vi "f dependence NLH_2Dsweep.vi"() -> ()   [LabVIEW 2022 SP3]
uses:
  C:/Program Files/National Instruments/LabVIEW 2022/instr.lib/OptiCool/QDInstrument.dll
  <vilib>/Analysis/baseanly.llb/Mean (DBL).vi
  <vilib>/Utility/file.llb/Write Delimited Spreadsheet (DBL).vi
  <vilib>/Analysis/NI_AALBase.lvlib
panel:
  in  "Log Step":dbl=1.0
  in  "End Value (Hz)":dbl=40000.0
  in  "Start Value (Hz)":dbl=17.7
  out "Frequency":dbl
  out "error out":errorcluster
  out "Instrument Ref Out":refnum<k24>
  in  "Temperature \n& Field Function":bool=TRUE
  in  "IP Address 2":string="169.254.170.239"
  in  "Remote":bool=TRUE
  in  "Delay":dbl=5.0
  in  "WaitForTemperature":bool=TRUE
  in  "WaitForField":bool=TRUE
  in  "Set  T  (K)":dbl=2.0
  in  "T  Rate (K/min)":dbl=10.0
  in  "Temperature Approach":i32(ring)=1 items=["FastSettle", "NoOvershoot"]
  in  "Mode":i32(ring) items=["Persistent", "Driven"]
  in  "Set F (Oe)":dbl format="%#_13g"
  in  "F Rate (Oe/s)":dbl=100.0 format="%#_13g"
  in  "Field Approach":i32(ring) items=["Linear", "NoOvershoot", "Oscillate"]
  out "Measuring":bool
  out "Temperature":dbl=2.045465922355652
  out "Field":dbl=-0.1023246817290783
  out "Field Status":i32(ring)=4 items=["MagnetUnknown"=0, "StablePersistent"=1, "WarmingSwitch"=2, "CoolingSwitch"=3, "StableDriven"=4, "Iterating"=5, "Charging"=6, "Discharging"=7, "CurrentError"=8, "MagnetFailure"=15]
  out "Temperature Status":i32(ring)=1 items=["TemperatureUnknown"=0, "Stable"=1, "Tracking"=2, "Near"=5, "Chasing"=6, "Filling"=7, "Standby"=10, "Disabled"=13, "ImpedanceNotFunction"=14, "TempFailure"=15]
  out "Ri_2 phase":cluster{dbl[], dbl[]}(graph)={[0.09999999999999998, 0.12, 0.14, 0.16000000000000003, 0.17999999999999994, 0.19999999999999996, 0.21999999999999997, 0.24, 0.26, 0.28, 0.29999999999999993, 0.31999999999999995, 0.33999999999999997, 0.36, 0.38, 0.4, 0.42000000000000004, 0.43999999999999995, 0.45999999999999996, 0.48, 0.5, 0.52, 0.54, 0.56, 0.5800000000000001, 0.6, 0.62, 0.64, 0.6599999999999999, 0.6799999999999999, 0.7, 0.72, 0.74, 0.76, 0.78, 0.8, 0.8200000000000001, 0.84, 0.86, 0.88, 0.9, 0.92, 0.94, 0.96, 0.98, 1.0, 0.98, 0.96, 0.94, 0.92, 0.9, 0.88, 0.86, 0.84, 0.82, 0.8, 0.78, 0.76, 0.74, 0.72, 0.7, 0.6799999999999999, 0.66, 0.64, 0.62, 0.6, 0.58, 0.56, 0.54, 0.52, 0.5, 0.48, 0.45999999999999996, 0.44000000000000006, 0.42000000000000004, 0.4, 0.38, 0.36, 0.33999999999999997, 0.32, 0.30000000000000004, 0.28, 0.26, 0.24000000000000002, 0.22, 0.2, 0.18, 0.16, 0.14, 0.12000000000000001, 0.1, 0.09999999999999998, 0.12, 0.14, 0.16000000000000003, 0.17999999999999994, 0.19999999999999996, 0.21999999999999997, 0.24, 0.26, 0.28, 0.29999999999999993, 0.31999999999999995, 0.33999999999999997, 0.36, 0.38, 0.4, 0.42000000000000004, 0.43999999999999995, 0.45999999999999996, 0.48, 0.5, 0.52, 0.54, 0.56, 0.5800000000000001, 0.6, 0.62, 0.64, 0.6599999999999999, 0.6799999999999999, 0.7, 0.72, 0.74, 0.76, 0.78, 0.8, 0.8200000000000001, 0.84, 0.86, 0.88, 0.9, 0.92, 0.94, 0.96, 0.98, 1.0, 0.98, 0.96, 0.94, 0.92, 0.9, 0.88, 0.86, 0.84, 0.82, 0.8, 0.78, 0.76, 0.74, 0.72, 0.7, 0.6799999999999999, 0.66, 0.64, 0.62, 0.6, 0.58, 0.56, 0.54, 0.52, 0.5, 0.48, 0.45999999999999996, 0.44000000000000006, 0.42000000000000004, 0.4, 0.38, 0.36, 0.33999999999999997, 0.32, 0.30000000000000004, 0.28, 0.26, 0.24000000000000002, 0.22, 0.2, 0.18, 0.16, 0.14, 0.12000000000000001, 0.1], [-135.0737798780838, -134.6738634306522, -134.37974821597692, -134.1329191164491, -133.93959648319287, -133.82499792211388, -133.72512789792637, -133.65178972403427, -133.51483265219323, -133.47620113245185, -133.49883143367305, -133.37910330366344, -133.21293365173887, -133.27350677537933, -133.27106017405902, -133.21754869761966, -133.21281374202516, -133.1841427403462, -133.16708735849346, -133.1229624716472, -133.09716887007846, -133.0742714725264, -133.06316615999822, -133.04544862618698, -133.02604088036725, -133.03034506308185, -133.00064263870803, -132.98704248472112, -132.95992367769645, -132.96773298284512, -132.9462513593375, -132.92388738374774, -132.93487095070657, -132.92245049681333, -132.91747172466938, -132.90231743575433, -132.88556409154268, -132.881237082976, -132.87117074587596, -132.86576987764798, -132.85386852066148, -132.84708304664974, -132.84538130977083, -132.83586557346655, -132.8255489140817, -132.82629889245763, -132.8177816715776, -132.82326025843324, -132.8336140133908, -132.8454189176914, -132.8516410833353, -132.85806140932092, -132.84285801056097, -132.84644282891838, -132.84700096802584, -132.84976756233482, -132.86482634382176, -132.86727458409388, -132.8588624021069, -132.88644179903636, -132.9058800327217, -132.87699682828833, -132.88999304396324, -132.91108879474103, -132.92301179840743, -132.92346083291895, -132.93641029158624, -132.94113870472373, -132.9606516890803, -132.96437166584263, -132.98433647368265, -132.9875119411151, -133.01231262066918, -133.0688900958854, -133.09190630466588, -133.1264003742024, -133.15155411140012, -133.93832528791813, -133.13251976736467, -133.22378740142432, -133.3539090592655, -133.3970887669385, -133.4425242756172, -133.49287186771852, -133.60223065290106, -133.75321879185125, -133.92848825397414, -134.11303813477105, -134.45190508345792, -135.10675452695267, -124.76072580560799, -89.50174321642196, -89.14605038980542, -88.84594353514626, -88.65669391405325, -88.50217230984028, -88.2292578588941, -88.20060177628105, -88.09441994431185, -88.00398201709041, -87.92508441731627, -87.88589798731445, -87.82014491326349, -87.79601841325153, -87.73700247935645, -87.69563779511853, -87.64024863816759, -87.6394010617623, -87.60257219060512, -87.55344363152862, -87.54324222165285, -87.51258348919042, -87.49839628540947, -87.48024090287525, -87.4663422228203, -87.44267105162086, -87.43676483856159, -87.40019935701899, -87.40049945685288, -87.38876942892429, -87.3757429912223, -87.35429406648153, -87.34428274476673, -87.33889962417248, -87.33853163161574, -87.32024261424039, -87.31903405804312, -87.30663336163828, -87.28680101385758, -87.28627293404885, -87.27451339574941, -87.26365333274687, -87.25364549630169, -87.24446928127777, -87.23761000479438, -87.24664691292533, -87.2206145740333, -87.22117860050086, -87.2360405527259, -87.23323381946209, -87.26842924538664, -87.23137885199706, -87.2385360459189, -87.25273929485618, -87.26039540250387, -87.25517989532322, -87.26120027002698, -87.25416045268364, -87.28418213348777, -87.29625747302379, -87.29755965406775, -87.29328958611812, -87.29095955610856, -87.30159590257846, -87.29739952834753, -87.32502449307063, -87.31280059465371, -87.34807549336224, -87.35104915499241, -87.35270893749001, -87.38974493852264, -87.42258216936716, -87.38265602907923, -87.42896961420581, -87.45151311724116, -87.47074471126548, -87.51773574830506, -87.56305113613072, -87.39521544539879, -87.67315367482476, -87.74315739254689, -87.74764259560797, -87.78722254082936, -87.87871776739563, -88.01195362145981, -88.22210844624024, -88.26255081520787, -88.37855415135323, -88.88064210120181, -89.15599768975594, -89.43545944095864, -67.88194047928333, -67.88194047928333]}
  out "Ri_1 phase":cluster{dbl[], dbl[]}(graph)={[0.09999999999999998, 0.12, 0.14, 0.16000000000000003, 0.17999999999999994, 0.19999999999999996, 0.21999999999999997, 0.24, 0.26, 0.28, 0.29999999999999993, 0.31999999999999995, 0.33999999999999997, 0.36, 0.38, 0.4, 0.42000000000000004, 0.43999999999999995, 0.45999999999999996, 0.48, 0.5, 0.52, 0.54, 0.56, 0.5800000000000001, 0.6, 0.62, 0.64, 0.6599999999999999, 0.6799999999999999, 0.7, 0.72, 0.74, 0.76, 0.78, 0.8, 0.8200000000000001, 0.84, 0.86, 0.88, 0.9, 0.92, 0.94, 0.96, 0.98, 1.0, 0.98, 0.96, 0.94, 0.92, 0.9, 0.88, 0.86, 0.84, 0.82, 0.8, 0.78, 0.76, 0.74, 0.72, 0.7, 0.6799999999999999, 0.66, 0.64, 0.62, 0.6, 0.58, 0.56, 0.54, 0.52, 0.5, 0.48, 0.45999999999999996, 0.44000000000000006, 0.42000000000000004, 0.4, 0.38, 0.36, 0.33999999999999997, 0.32, 0.30000000000000004, 0.28, 0.26, 0.24000000000000002, 0.22, 0.2, 0.18, 0.16, 0.14, 0.12000000000000001, 0.1, 0.09999999999999998, 0.12, 0.14, 0.16000000000000003, 0.17999999999999994, 0.19999999999999996, 0.21999999999999997, 0.24, 0.26, 0.28, 0.29999999999999993, 0.31999999999999995, 0.33999999999999997, 0.36, 0.38, 0.4, 0.42000000000000004, 0.43999999999999995, 0.45999999999999996, 0.48, 0.5, 0.52, 0.54, 0.56, 0.5800000000000001, 0.6, 0.62, 0.64, 0.6599999999999999, 0.6799999999999999, 0.7, 0.72, 0.74, 0.76, 0.78, 0.8, 0.8200000000000001, 0.84, 0.86, 0.88, 0.9, 0.92, 0.94, 0.96, 0.98, 1.0, 0.98, 0.96, 0.94, 0.92, 0.9, 0.88, 0.86, 0.84, 0.82, 0.8, 0.78, 0.76, 0.74, 0.72, 0.7, 0.6799999999999999, 0.66, 0.64, 0.62, 0.6, 0.58, 0.56, 0.54, 0.52, 0.5, 0.48, 0.45999999999999996, 0.44000000000000006, 0.42000000000000004, 0.4, 0.38, 0.36, 0.33999999999999997, 0.32, 0.30000000000000004, 0.28, 0.26, 0.24000000000000002, 0.22, 0.2, 0.18, 0.16, 0.14, 0.12000000000000001, 0.1], [126.78108864351137, 127.45286903626857, 127.95719233953537, 128.14548768192813, 128.2402724756276, 128.4605048589487, 128.66016247507395, 128.78004628646207, 128.85380119553557, 128.945308050546, 129.00594825216675, 129.1174793127654, 125.93035564325805, 128.99616398776885, 129.01096513526798, 128.99858528612694, 129.03821355303282, 129.0423277101241, 129.1060564530601, 129.12134565618365, 129.12218412588027, 129.16712187372542, 129.1716351205436, 129.1576166175744, 129.1739493965666, 129.22295454798373, 129.2303923286002, 129.2532206876488, 129.22564402818136, 129.24977504964798, 129.25454428704774, 129.2236334227617, 129.24706199685042, 129.2433757601247, 129.26065634538244, 129.24704726302411, 129.26737715657828, 129.25153494751845, 129.246018320394, 129.27084220325727, 129.26200021632502, 129.2815900734443, 129.25572165721184, 129.2713787153919, 129.27714146359114, 129.26320898916032, 129.26130754745333, 129.23228748819213, 129.23260322371937, 129.24085101357815, 129.20001021516066, 129.18928968116475, 129.22736479334458, 129.23076137993036, 129.21676154055228, 129.16377399211459, 129.1488883594887, 129.14107631735763, 129.17351120766202, 129.13764733091995, 129.13942445055497, 129.13611111142535, 129.12439365492142, 129.09365051881986, 129.04689998820783, 129.07255318625485, 129.0762023274164, 129.03056853240804, 128.98843713843775, 129.00993007515308, 128.96980878114644, 128.97196179961242, 128.93367450266246, 128.8432547892745, 128.77294830523502, 128.77850864107342, 128.26159472371137, 120.9819473629494, 128.91362581026087, 128.85130036343432, 128.75506679568952, 128.64553318215607, 128.5269184940437, 128.37639368365402, 128.19973263276748, 128.11080720159285, 127.84397610864357, 127.57598196631716, 127.36840896927713, 126.4699555939904, 122.15900482546692, -155.25487809300571, -154.75930960822615, -154.06908162364144, -153.69651442588355, -153.35566603542182, -153.23294540243333, -153.1114136645777, -152.8025382830503, -152.64398344398305, -152.52815097235072, -152.39578139944246, -152.4164853144777, -160.759413971048, -152.37498784365977, -152.3997145906726, -152.3686132746472, -152.27205329420735, -152.22153743200627, -152.20204337088634, -152.06607044245763, -152.0586998411544, -152.08655249501595, -152.03743666503073, -151.98381101431457, -151.9606367889107, -151.91112648537748, -151.92318997154743, -151.88886269968575, -151.86095513823875, -151.84712349726647, -151.8467203751335, -151.83654816655485, -151.83466546583742, -151.77972437121562, -151.75955524254454, -151.74101876892612, -151.74814437160126, -151.73846749290755, -151.71965063994767, -151.73507745360297, -151.70148169603394, -151.68277714268805, -151.68376267193642, -151.6789107792956, -151.68539186653047, -151.6809435268432, -151.69581765024503, -151.69398875114774, -151.71075155504255, -151.74117286964352, -151.75504731698328, -151.7397603042772, -151.78231484385356, -151.79544209254783, -151.80143331080117, -151.84067413704435, -151.85962716508706, -151.87822739965404, -151.91103936506607, -151.91923332818104, -151.93509570614805, -151.98136529122525, -151.97685217566038, -152.0012327141608, -152.02285309703487, -152.09741752528834, -152.1068998768356, -152.12333750684087, -152.15249427417922, -152.21610575405555, -152.28574184251096, -152.29089791668042, -152.30516178154488, -152.35145853535226, -152.450566439704, -152.50934427301326, -152.70530235536185, -153.48538331429216, -152.54768281995285, -152.61612358031286, -152.75102902160276, -152.87046583001037, -153.08098511590293, -153.26088730787697, -153.53049426796596, -153.64021310128948, -153.88983077611812, -154.39490952060976, -154.97594326878533, -154.724275972751, -25.54701889784434]}
  out "Ri_2":cluster{dbl[], dbl[]}(graph)={[0.09999999999999998, 0.12, 0.14, 0.16000000000000003, 0.17999999999999994, 0.19999999999999996, 0.21999999999999997, 0.24, 0.26, 0.28, 0.29999999999999993, 0.31999999999999995, 0.33999999999999997, 0.36, 0.38, 0.4, 0.42000000000000004, 0.43999999999999995, 0.45999999999999996, 0.48, 0.5, 0.52, 0.54, 0.56, 0.5800000000000001, 0.6, 0.62, 0.64, 0.6599999999999999, 0.6799999999999999, 0.7, 0.72, 0.74, 0.76, 0.78, 0.8, 0.8200000000000001, 0.84, 0.86, 0.88, 0.9, 0.92, 0.94, 0.96, 0.98, 1.0, 0.98, 0.96, 0.94, 0.92, 0.9, 0.88, 0.86, 0.84, 0.82, 0.8, 0.78, 0.76, 0.74, 0.72, 0.7, 0.6799999999999999, 0.66, 0.64, 0.62, 0.6, 0.58, 0.56, 0.54, 0.52, 0.5, 0.48, 0.45999999999999996, 0.44000000000000006, 0.42000000000000004, 0.4, 0.38, 0.36, 0.33999999999999997, 0.32, 0.30000000000000004, 0.28, 0.26, 0.24000000000000002, 0.22, 0.2, 0.18, 0.16, 0.14, 0.12000000000000001, 0.1, 0.09999999999999998, 0.12, 0.14, 0.16000000000000003, 0.17999999999999994, 0.19999999999999996, 0.21999999999999997, 0.24, 0.26, 0.28, 0.29999999999999993, 0.31999999999999995, 0.33999999999999997, 0.36, 0.38, 0.4, 0.42000000000000004, 0.43999999999999995, 0.45999999999999996, 0.48, 0.5, 0.52, 0.54, 0.56, 0.5800000000000001, 0.6, 0.62, 0.64, 0.6599999999999999, 0.6799999999999999, 0.7, 0.72, 0.74, 0.76, 0.78, 0.8, 0.8200000000000001, 0.84, 0.86, 0.88, 0.9, 0.92, 0.94, 0.96, 0.98, 1.0, 0.98, 0.96, 0.94, 0.92, 0.9, 0.88, 0.86, 0.84, 0.82, 0.8, 0.78, 0.76, 0.74, 0.72, 0.7, 0.6799999999999999, 0.66, 0.64, 0.62, 0.6, 0.58, 0.56, 0.54, 0.52, 0.5, 0.48, 0.45999999999999996, 0.44000000000000006, 0.42000000000000004, 0.4, 0.38, 0.36, 0.33999999999999997, 0.32, 0.30000000000000004, 0.28, 0.26, 0.24000000000000002, 0.22, 0.2, 0.18, 0.16, 0.14, 0.12000000000000001, 0.1], [27.371127865925015, 28.03873360270576, 28.46790461906138, 28.806943395600985, 29.071407285608636, 29.323295423352075, 29.462283711911706, 29.588953410180608, 29.706307017591357, 29.804227381977352, 29.87886111106559, 29.996116648909492, 30.195931132223937, 29.9884898058237, 30.055397066752594, 30.063982766666918, 30.109896580846595, 30.179554870002743, 30.170072825304572, 30.175397841954556, 30.20266242174663, 30.199676710261986, 30.20862007206962, 30.232010687672023, 30.25006843906505, 30.208577391057474, 30.285871424440206, 30.25536260196531, 30.24120314721451, 30.23077945837067, 30.230477005377466, 30.22206486695692, 30.225997495742032, 30.230263862260664, 30.20740393202253, 30.211300547061118, 30.21208431622353, 30.184907444070042, 30.182773909229088, 30.17902335943376, 30.16788755735149, 30.146107050335754, 30.134406107300926, 30.122307887553678, 30.13298693800453, 31.202979545844265, 31.210305140532736, 31.274406560955054, 31.305924728646062, 31.32743742693625, 31.375770721793792, 31.41382858703819, 31.45271665563307, 31.46916619733765, 31.532341922014098, 31.579997682637718, 31.59500614453121, 31.646800008509103, 31.695365022790494, 31.746853486268666, 31.798078625890966, 31.824707946574527, 31.89690056166134, 31.94018053437305, 32.01268881637008, 32.06636872763467, 32.135039395345515, 32.19692297138488, 32.260290459052655, 32.31072327457344, 32.380782444119205, 32.46545102212157, 32.534119464205524, 32.65882509715479, 32.72562027716687, 32.772164759910204, 31.414326516917146, 27.175202751891387, 32.99406085081532, 33.1423739100909, 33.28288253006214, 33.48812700032473, 33.73611411646078, 33.9781939345709, 34.29950602104752, 34.61918175500793, 35.06293433592041, 35.49518695051094, 36.256808448279884, 38.31013406059865, 501.19496515581875, 26.805737505344652, 27.450048924243337, 27.884394712122138, 28.24044516317822, 28.53430295508529, 28.764528334010045, 28.96197838575729, 29.105816365304005, 29.355232984041944, 29.34777886019463, 29.43287936231009, 29.62774349540086, 29.86465695141408, 29.608272863377074, 29.66921999186081, 29.70063847337968, 29.714424220713198, 29.786978685230352, 29.814319234323147, 29.826654999997462, 29.858808079716006, 29.84850588904362, 29.835423649303713, 29.871251466983324, 29.904019985626224, 29.899198678955656, 29.906795896054145, 29.90400614385718, 29.903859410313423, 29.90866679269539, 29.906609993632678, 29.89947029239501, 29.889654317635724, 29.914131514562797, 29.89903218199667, 29.896801089141448, 29.893727436511856, 29.88599371103664, 29.87423537654639, 29.86604845504494, 29.873501668548162, 29.84836006279222, 29.8497650723906, 29.851025865972254, 29.855406310478582, 30.90378884193393, 30.92260344391088, 30.965941923321747, 31.007698997219396, 31.03181453129471, 31.079098855420387, 31.111474766773938, 31.14532041453912, 31.190307610789297, 31.239550892642928, 31.26858596616326, 31.30525453943163, 31.36698598822591, 31.407572289858972, 31.432621279246682, 31.48459816196743, 31.533379016650517, 31.569188358430146, 31.66020477677031, 31.70991492962698, 31.733959217395633, 31.78738364022895, 31.87665028118242, 31.942457880633185, 31.988808527675072, 32.0825556507543, 32.17690322547313, 32.158098239659864, 32.263369173607806, 32.348466821304804, 32.43680396652162, 31.651152253438767, 28.498596681427244, 32.633886474836245, 32.72261637427303, 32.90277867221614, 33.09550043742226, 33.27705165299585, 33.54280965027385, 33.79957889026999, 34.12170714222017, 34.63130452806735, 35.09460603644337, 35.815529001325366, 38.05801784237739, 581.0849422120803, 581.0849422120803]}
  out "Ri_1":cluster{dbl[], dbl[]}(graph)={[0.09999999999999998, 0.12, 0.14, 0.16000000000000003, 0.17999999999999994, 0.19999999999999996, 0.21999999999999997, 0.24, 0.26, 0.28, 0.29999999999999993, 0.31999999999999995, 0.33999999999999997, 0.36, 0.38, 0.4, 0.42000000000000004, 0.43999999999999995, 0.45999999999999996, 0.48, 0.5, 0.52, 0.54, 0.56, 0.5800000000000001, 0.6, 0.62, 0.64, 0.6599999999999999, 0.6799999999999999, 0.7, 0.72, 0.74, 0.76, 0.78, 0.8, 0.8200000000000001, 0.84, 0.86, 0.88, 0.9, 0.92, 0.94, 0.96, 0.98, 1.0, 0.98, 0.96, 0.94, 0.92, 0.9, 0.88, 0.86, 0.84, 0.82, 0.8, 0.78, 0.76, 0.74, 0.72, 0.7, 0.6799999999999999, 0.66, 0.64, 0.62, 0.6, 0.58, 0.56, 0.54, 0.52, 0.5, 0.48, 0.45999999999999996, 0.44000000000000006, 0.42000000000000004, 0.4, 0.38, 0.36, 0.33999999999999997, 0.32, 0.30000000000000004, 0.28, 0.26, 0.24000000000000002, 0.22, 0.2, 0.18, 0.16, 0.14, 0.12000000000000001, 0.1, 0.09999999999999998, 0.12, 0.14, 0.16000000000000003, 0.17999999999999994, 0.19999999999999996, 0.21999999999999997, 0.24, 0.26, 0.28, 0.29999999999999993, 0.31999999999999995, 0.33999999999999997, 0.36, 0.38, 0.4, 0.42000000000000004, 0.43999999999999995, 0.45999999999999996, 0.48, 0.5, 0.52, 0.54, 0.56, 0.5800000000000001, 0.6, 0.62, 0.64, 0.6599999999999999, 0.6799999999999999, 0.7, 0.72, 0.74, 0.76, 0.78, 0.8, 0.8200000000000001, 0.84, 0.86, 0.88, 0.9, 0.92, 0.94, 0.96, 0.98, 1.0, 0.98, 0.96, 0.94, 0.92, 0.9, 0.88, 0.86, 0.84, 0.82, 0.8, 0.78, 0.76, 0.74, 0.72, 0.7, 0.6799999999999999, 0.66, 0.64, 0.62, 0.6, 0.58, 0.56, 0.54, 0.52, 0.5, 0.48, 0.45999999999999996, 0.44000000000000006, 0.42000000000000004, 0.4, 0.38, 0.36, 0.33999999999999997, 0.32, 0.30000000000000004, 0.28, 0.26, 0.24000000000000002, 0.22, 0.2, 0.18, 0.16, 0.14, 0.12000000000000001, 0.1], [6066.597237124425, 4258.732617987017, 3060.2224219718946, 1956.8734062299268, 1038.0191464746251, 253.0540373770548, -431.9467240937055, -1043.0122865040687, -1600.4653309971861, -2077.4338083601374, -2508.623622234725, -2744.538661435745, -3936.952362108022, -3555.4039565792923, -3857.551091423043, -4130.164045633881, -4342.495968947174, -4553.498226383564, -4773.544199138, -4976.971516505818, -5143.30957699489, -5285.2330025634155, -5437.2139442330545, -5587.455286087704, -5697.776044037766, -5822.271287616122, -5918.291526951003, -6006.124748885252, -6104.734647303527, -6217.145779571478, -6284.653534409701, -6367.082275540494, -6427.74394785674, -6501.458553625916, -6563.2851119177085, -6610.946750304625, -6654.752154465894, -6717.997649264144, -6776.302014832963, -6811.8846905801065, -6866.421210638462, -6910.9932666402, -6932.8353919940055, -6977.756396192704, -7013.447964342136, -7340.511127882765, -7307.932336482773, -7283.562030272092, -7252.008088733441, -7219.7129418001405, -7199.750700574299, -7149.615192573897, -7266.801072885218, -6837.783974413332, -7016.019884518875, -6959.342919603375, -6906.791111511307, -6845.792766487819, -6779.338051555759, -6720.698513348367, -6640.697566589129, -6593.507323035513, -6481.977415599831, -6388.907798747582, -6316.355328198112, -6210.1538518181305, -6091.766024112317, -5964.802511827463, -5773.517304986142, -5685.708933994015, -5558.036451448384, -5380.233892175308, -5201.1388726949035, -5006.763343731122, -4784.755489704853, -4548.303581449232, -4328.3194364048195, -4534.454062871044, -3664.772067185334, -3327.2281124532806, -3253.0751194454115, -1533.3096848405557, -1815.2518132117295, -1177.2580303103216, -433.2441539712868, 409.11394693386774, 1409.3861561511105, 2668.486059312522, 4257.1583901951535, 6367.063356134498, 36021.945440264695, 5196.440467020697, 3987.848204197968, 2958.0575085274236, 2085.994326776163, 1268.099887963653, 576.6532930777661, -34.47519840886286, -560.8751683866506, -1036.0325927169301, -1469.1055632432299, -1912.2938248842124, -2276.1991334113027, -2737.8397332598956, -2923.399200819077, -3174.10756748418, -3421.81325318595, -3692.5208095883113, -3905.8004897911337, -4117.5254916475005, -4301.602150888721, -4496.604091630743, -4658.696530591691, -4791.3891291791115, -4934.475050566723, -5063.416086831616, -5191.4053801297905, -5299.8207430649, -5405.425838948669, -5514.139422466482, -5623.424619229143, -5711.845721659744, -5804.735296293655, -5889.212343534356, -5962.737083520788, -6038.641970231026, -6098.696983683368, -6158.8454259840155, -6215.560795392968, -6269.139290286868, -6306.302154071724, -6368.55452203165, -6419.0286790626815, -6452.160269300591, -6501.054373654349, -6544.163041352561, -6854.592808596113, -6823.216437688578, -6787.546246385524, -6746.546459667489, -6709.89241991804, -6666.633718684863, -6621.921127645494, -6573.718240260894, -6520.9134940134145, -6470.041163400641, -6403.675173138959, -6340.6832737763825, -6278.99285489665, -6202.58030000932, -6118.575661359277, -6050.134088288392, -5956.307086959962, -5882.863404327877, -5761.921801607788, -5652.712017396368, -5539.048836720829, -5415.161988102774, -5299.501542289932, -5155.236062465217, -5274.484367495612, -4329.459128124873, -4661.700890388149, -4490.845523775327, -4297.377050379922, -4021.9232816316244, -3763.681884465588, -3502.238532819534, -3262.4614614960683, -2854.591928334535, -2419.2512007316145, -2011.3588168814365, -1548.008313191706, -1018.6261652521694, -451.06428223908335, 1206.5403387077765, 985.6235797520325, 1959.9304792325481, 3794.9473315345517, 5561.473045619704, 6614.127068683538, 5775.2823286764105]}
  out "Device 2 phase":dbl=-135.0737798780838 format="%.3p"
  out "Device 1 phase":dbl=126.78108864351137 format="%.3p"
  out "Ri_2(Ohm)":dbl=27.371127865925015
  out "Ri_1(Ohm)":dbl=6066.597237124425
  out "Device2 Current(mA)":dbl=0.015156225082873367
  out "Device1 Current(mA)":dbl=0.0003008227313801997
  in  "R2(Kohm)":dbl=1.9997 format="%#_13g"
  in  "R1(Kohm)":dbl=2.0265 format="%#_13g"
  in  "R2 Sensitivity":u16(ring)=26 items=["1 nV/fA", "2 nV/fA", "5 nV/fA", "10 nV/fA", "20 nV/fA", "50 nV/fA", "100 nV/fA", "200 nV/fA", "500 nV/fA", "1 uV/pA", "2 uV/pA", "5 uV/pA", "10 uV/pA", "20 uV/pA", "50 uV/pA", "100 uV/pA", "200 uV/pA", "500 uV/pA", "1 mV/nA", "2 mV/nA", "5 mV/nA", "10 mV/nA", "20 mV/nA", "50 mV/nA", "100 mV/nA", "200 mV/nA", "500 mV/nA", "1 V/uA"]
  in  "R2 Current T Constant":u8(ring)=9 items=["10 us", "30 us", "100 us", "300 us", "1 ms", "3 ms", "10 ms", "30 ms", "100 ms", "300 ms", "1 s", "3 s", "10 s", "30 s", "100 s", "300 s", "1 ks", "3 ks"]
  in  "R1 Current T Constant":u8(ring)=9 items=["10 us", "30 us", "100 us", "300 us", "1 ms", "3 ms", "10 ms", "30 ms", "100 ms", "300 ms", "1 s", "3 s", "10 s", "30 s", "100 s", "300 s", "1 ks", "3 ks"]
  in  "R1 Current sensitivity":u16(ring)=26 items=["1 nV/fA", "2 nV/fA", "5 nV/fA", "10 nV/fA", "20 nV/fA", "50 nV/fA", "100 nV/fA", "200 nV/fA", "500 nV/fA", "1 uV/pA", "2 uV/pA", "5 uV/pA", "10 uV/pA", "20 uV/pA", "50 uV/pA", "100 uV/pA", "200 uV/pA", "500 uV/pA", "1 mV/nA", "2 mV/nA", "5 mV/nA", "10 mV/nA", "20 mV/nA", "50 mV/nA", "100 mV/nA", "200 mV/nA", "500 mV/nA", "1 V/uA"]
  in  "LOCKIN3 address":refnum<visa-resource-name>="COM5"
  in  "Current measurement?":bool=TRUE
  in  "Parameter 1B 1":u16(ring)=2 items=["X", "Y", "R", "Theta", "Frequency", "Noise", "Xh1", "Yh1", "Rh1", "Theta h1", "Xh2", "Yh2", "Rh2", "Theta h2"]
  in  "Phase 1B 1":u16(ring)=3 items=["X", "Y", "R", "Theta", "Frequency", "Noise", "Xh1", "Yh1", "Rh1", "Theta h1", "Xh2", "Yh2", "Rh2", "Theta h2"]
  out "Vab_1(1w)/mV":dbl=1.8249703510553426
  out "phase Vab_1":dbl=0.0018169224795393922
  out "Vab_1/mV":cluster{dbl[], dbl[]}(graph)={[0.09999999999999998, 0.12, 0.14, 0.16000000000000003, 0.17999999999999994, 0.19999999999999996, 0.21999999999999997, 0.24, 0.26, 0.28, 0.29999999999999993, 0.31999999999999995, 0.33999999999999997, 0.36, 0.38, 0.4, 0.42000000000000004, 0.43999999999999995, 0.45999999999999996, 0.48, 0.5, 0.52, 0.54, 0.56, 0.5800000000000001, 0.6, 0.62, 0.64, 0.6599999999999999, 0.6799999999999999, 0.7, 0.72, 0.74, 0.76, 0.78, 0.8, 0.8200000000000001, 0.84, 0.86, 0.88, 0.9, 0.92, 0.94, 0.96, 0.98, 1.0, 0.98, 0.96, 0.94, 0.92, 0.9, 0.88, 0.86, 0.84, 0.82, 0.8, 0.78, 0.76, 0.74, 0.72, 0.7, 0.6799999999999999, 0.66, 0.64, 0.62, 0.6, 0.58, 0.56, 0.54, 0.52, 0.5, 0.48, 0.45999999999999996, 0.44000000000000006, 0.42000000000000004, 0.4, 0.38, 0.36, 0.33999999999999997, 0.32, 0.30000000000000004, 0.28, 0.26, 0.24000000000000002, 0.22, 0.2, 0.18, 0.16, 0.14, 0.12000000000000001, 0.1, 0.09999999999999998, 0.12, 0.14, 0.16000000000000003, 0.17999999999999994, 0.19999999999999996, 0.21999999999999997, 0.24, 0.26, 0.28, 0.29999999999999993, 0.31999999999999995, 0.33999999999999997, 0.36, 0.38, 0.4, 0.42000000000000004, 0.43999999999999995, 0.45999999999999996, 0.48, 0.5, 0.52, 0.54, 0.56, 0.5800000000000001, 0.6, 0.62, 0.64, 0.6599999999999999, 0.6799999999999999, 0.7, 0.72, 0.74, 0.76, 0.78, 0.8, 0.8200000000000001, 0.84, 0.86, 0.88, 0.9, 0.92, 0.94, 0.96, 0.98, 1.0, 0.98, 0.96, 0.94, 0.92, 0.9, 0.88, 0.86, 0.84, 0.82, 0.8, 0.78, 0.76, 0.74, 0.72, 0.7, 0.6799999999999999, 0.66, 0.64, 0.62, 0.6, 0.58, 0.56, 0.54, 0.52, 0.5, 0.48, 0.45999999999999996, 0.44000000000000006, 0.42000000000000004, 0.4, 0.38, 0.36, 0.33999999999999997, 0.32, 0.30000000000000004, 0.28, 0.26, 0.24000000000000002, 0.22, 0.2, 0.18, 0.16, 0.14, 0.12000000000000001, 0.1], [1.8249703510553426, 1.6321149961963433, 1.387429363236547, 1.0496619190193917, 0.6471446776639771, 0.1800489178618506, -0.3462389934889975, -0.9377648702143228, -1.5996699791173674, -2.278121399132181, -3.023922122416686, -3.7848219685766087, -5.293703684189235, -5.453431430544369, -6.359391347059302, -7.264121027087279, -8.164509203653134, -9.144776240980534, -10.159757520784167, -11.222250518009227, -12.233873776890158, -13.26123254146302, -14.34467837465278, -15.454641196951263, -16.541126258814142, -17.69144060868247, -18.794544634046552, -19.961351956482858, -21.138144350209565, -22.358594990528132, -23.53216931064686, -24.758534174137946, -25.97319713914828, -27.21740619180225, -28.452475685651574, -29.729296230553242, -31.00620041732565, -32.26470320089088, -33.557758275765835, -34.83978053094051, -36.17345402403799, -37.48402936553257, -38.73492204768241, -40.14898379386943, -41.50322574980898, -42.848495089415806, -41.485622949379874, -40.16291660343985, -38.81321804865196, -37.491974519907366, -36.17225430151935, -34.847551661741115, -33.5098967566045, -30.921013545187265, -30.943928464049883, -29.65364978427231, -28.406729316879932, -27.152749943479876, -25.894715086040307, -24.672024924671376, -23.466325759880178, -22.259841199015597, -21.050922315436004, -19.86327973514115, -18.70985231440603, -17.57508945931816, -16.455161488254404, -15.357310078563257, -14.255041710842377, -13.175321361855332, -12.137899693138156, -11.106703193263897, -10.111806483923184, -9.12875234195201, -8.167419670608997, -7.248166581272961, -6.3237308678945245, -5.653528135186191, -4.610406575310699, -3.8263653809578284, -3.096803874573654, -1.3962148482952377, -1.5457179422405913, -0.8893752625453888, -0.28829608984595906, 0.2362450960782543, 0.6879448177663117, 1.0950792639997124, 1.4216584091719764, 1.663935194119896, 1.8021850368316876, 1.6022259761560622, 1.5215037735260863, 1.3583424734037821, 1.1328184494954519, 0.8051330391087875, 0.41499181259993395, -0.028040511695311885, -0.5143289120570268, -1.0540721791907601, -1.6454999650580293, -2.3397786237106946, -3.0280889473575483, -3.7668276361041513, -4.565001194423907, -5.317136927806049, -6.13690407660819, -7.06706473520211, -7.947865943754197, -8.877988236774966, -9.827942144003167, -10.833121108804441, -11.82362665819828, -12.80475083381254, -13.853527978122385, -14.893627794955687, -15.989007159220758, -17.059963178601585, -18.17887486896272, -19.323369053894222, -20.515333512033838, -21.684043142242544, -22.877402541603725, -24.041111183999035, -25.25487691721768, -26.502934001954365, -27.688152027553823, -28.918010657764086, -30.168335179342293, -31.428469040690175, -32.66256788683826, -33.93987161340675, -35.22628960912447, -36.49379313520381, -37.80072940368133, -39.101632365104955, -40.424102923426084, -39.10763466617498, -37.81000039915504, -36.51047421654706, -35.218608282796616, -33.92722147266897, -32.61964581867935, -31.361902727697732, -30.114218406814025, -28.889976026329695, -27.632820154125938, -26.362637993538744, -25.16893379488242, -23.978086805310344, -22.779432603112888, -21.596861759905917, -20.413211310952647, -19.277555758680194, -18.152513993547007, -17.023442726522727, -15.938833901733108, -14.846468076463639, -13.799799525151782, -12.753289600751971, -11.739168469488266, -9.395827755202186, -9.769592353727509, -8.841029918029962, -7.893220339062424, -6.964937468471132, -6.080508807589176, -5.277568728939468, -4.530215785492297, -3.6172027705457985, -2.829371558003297, -2.14306551907009, -1.4851489389142507, -0.879821596866845, -0.3036578955343671, 0.776132251286894, 0.5819694155273969, 0.9833305104059085, 1.2974768912725065, 1.760115343854087, 1.6802094475608393, 1.7443426093343017]}
  out "phase Vab_1":cluster{dbl[], dbl[]}(graph)={[0.09999999999999998, 0.12, 0.14, 0.16000000000000003, 0.17999999999999994, 0.19999999999999996, 0.21999999999999997, 0.24, 0.26, 0.28, 0.29999999999999993, 0.31999999999999995, 0.33999999999999997, 0.36, 0.38, 0.4, 0.42000000000000004, 0.43999999999999995, 0.45999999999999996, 0.48, 0.5, 0.52, 0.54, 0.56, 0.5800000000000001, 0.6, 0.62, 0.64, 0.6599999999999999, 0.6799999999999999, 0.7, 0.72, 0.74, 0.76, 0.78, 0.8, 0.8200000000000001, 0.84, 0.86, 0.88, 0.9, 0.92, 0.94, 0.96, 0.98, 1.0, 0.98, 0.96, 0.94, 0.92, 0.9, 0.88, 0.86, 0.84, 0.82, 0.8, 0.78, 0.76, 0.74, 0.72, 0.7, 0.6799999999999999, 0.66, 0.64, 0.62, 0.6, 0.58, 0.56, 0.54, 0.52, 0.5, 0.48, 0.45999999999999996, 0.44000000000000006, 0.42000000000000004, 0.4, 0.38, 0.36, 0.33999999999999997, 0.32, 0.30000000000000004, 0.28, 0.26, 0.24000000000000002, 0.22, 0.2, 0.18, 0.16, 0.14, 0.12000000000000001, 0.1, 0.09999999999999998, 0.12, 0.14, 0.16000000000000003, 0.17999999999999994, 0.19999999999999996, 0.21999999999999997, 0.24, 0.26, 0.28, 0.29999999999999993, 0.31999999999999995, 0.33999999999999997, 0.36, 0.38, 0.4, 0.42000000000000004, 0.43999999999999995, 0.45999999999999996, 0.48, 0.5, 0.52, 0.54, 0.56, 0.5800000000000001, 0.6, 0.62, 0.64, 0.6599999999999999, 0.6799999999999999, 0.7, 0.72, 0.74, 0.76, 0.78, 0.8, 0.8200000000000001, 0.84, 0.86, 0.88, 0.9, 0.92, 0.94, 0.96, 0.98, 1.0, 0.98, 0.96, 0.94, 0.92, 0.9, 0.88, 0.86, 0.84, 0.82, 0.8, 0.78, 0.76, 0.74, 0.72, 0.7, 0.6799999999999999, 0.66, 0.64, 0.62, 0.6, 0.58, 0.56, 0.54, 0.52, 0.5, 0.48, 0.45999999999999996, 0.44000000000000006, 0.42000000000000004, 0.4, 0.38, 0.36, 0.33999999999999997, 0.32, 0.30000000000000004, 0.28, 0.26, 0.24000000000000002, 0.22, 0.2, 0.18, 0.16, 0.14, 0.12000000000000001, 0.1], [0.0018169224795393922, 0.0016286017899875692, 0.0013841724629621924, 0.0010451879278479245, 0.0006435810413141405, 0.00017530405517735708, -0.00035036914856200423, -0.0009430541055727321, -0.0016050871104377328, -0.002283121347803712, -0.0030225912390716815, -0.0037744287749389644, -0.00529863269633907, -0.005453317215155266, -0.006367383397624385, -0.007263417155237933, -0.008172017192326214, -0.009156796540115716, -0.010170489949214392, -0.01122607997658626, -0.01224091993502362, -0.013266871902537706, -0.014355696174730129, -0.015459993526366294, -0.016545898231592672, -0.017699187656370845, -0.01879689218278246, -0.01996946989165384, -0.021146012757372545, -0.02237784005418682, -0.023538801526883625, -0.024764707356456965, -0.02598352985619563, -0.02722552684431387, -0.028460209070076386, -0.029737304505969904, -0.031012095625060805, -0.032270829049713505, -0.03356344608111662, -0.03484930692660819, -0.03618176278809369, -0.03749293800476279, -0.03874212004308652, -0.040156747765477306, -0.04151309935020002, -0.04284266817793264, -0.04148214277996096, -0.040159310258309586, -0.03880530437492672, -0.037482835708526265, -0.036163890261814394, -0.034840044229961696, -0.03348827739390091, -0.030919837880955682, -0.03094274238612631, -0.029648697779789478, -0.028395444193222662, -0.02714762136937891, -0.02588563209244695, -0.024662445514676667, -0.02345820364395689, -0.022254493453886123, -0.021045229940519647, -0.019867053333630456, -0.018704948032995567, -0.017566319330435128, -0.016446396131051293, -0.01535555870973688, -0.014247622023505028, -0.013171515468594552, -0.012133585518585595, -0.011099710491904403, -0.010104349735440957, -0.009124384025776627, -0.008163133924839357, -0.007245198403983279, -0.00631475043105319, -0.005680716892248068, -0.004595309101790705, -0.0038300022219878737, -0.0030794611780201216, -0.0013968056573670745, -0.0015416262846490094, -0.0008875687815929868, -0.00028660156534344674, 0.00023688824317147692, 0.0006911357959818779, 0.001096391030429825, 0.0014221769877048288, 0.0016651907130233866, 0.0017940197621080563, 0.0016016426400879528, 0.001521909998770395, 0.0013580904729947742, 0.0011312007058540078, 0.0008015310710498673, 0.00041208031671264233, -3.123540602349157e-05, -0.0005129698706260962, -0.0010577290290732552, -0.0016494024796198316, -0.0023565406774138835, -0.003043674851001929, -0.0037550859511077312, -0.004572449852172398, -0.005330823461728843, -0.0061490169202117525, -0.007074321297173722, -0.007959818759217394, -0.008887280884498366, -0.009834486921317047, -0.010840396640262234, -0.011831069165134347, -0.012809259679543022, -0.01385914535171158, -0.014899011627456465, -0.0159948551931848, -0.017062228101559652, -0.018188310995764977, -0.019331322552236224, -0.02052245412252963, -0.02169162583340293, -0.022884462169802326, -0.024045647662858646, -0.02526001962577018, -0.026507327911419985, -0.027700422393136914, -0.028926981963448277, -0.03017636542592243, -0.03143659103893886, -0.032668676924134804, -0.033947943675467065, -0.035228121800822534, -0.03650244133088703, -0.03781139809375217, -0.03911142220454173, -0.04041868673754902, -0.03909909605011214, -0.03780658849372983, -0.03650605717713579, -0.03521223608773907, -0.033919393265272345, -0.032610814762468944, -0.03135649684399219, -0.030109111400274963, -0.028882133826852986, -0.027624754339764836, -0.02635410008244062, -0.025163928171947576, -0.023969777159217685, -0.022773172588454394, -0.021588663155385976, -0.02040368402872009, -0.01926997484479164, -0.018143660076434375, -0.017017045456944647, -0.015933409166174854, -0.014839643773129504, -0.013794748733095556, -0.012750455770033756, -0.011724317662098032, -0.009397261663947044, -0.009764373784469505, -0.008827262831347108, -0.007888999808574049, -0.00696686179679942, -0.0060719231917014645, -0.005280792147825468, -0.004533996452992602, -0.0036194311463449633, -0.002823643269299049, -0.002139265812857773, -0.0014788783608078058, -0.0008839232944956039, -0.00031002567850181475, 0.0007750348143549825, 0.0005837992131248255, 0.0009856130937742021, 0.0013018046138473026, 0.001760747911829679, 0.0016811044159116266, 0.0017353621173214141]}
  out "Vab_2(1w)/mV":dbl=0.41484297470806686
  in  "Parameter 2B 1":u16(ring)=2 items=["X", "Y", "R", "Theta", "Frequency", "Noise", "Xh1", "Yh1", "Rh1", "Theta h1", "Xh2", "Yh2", "Rh2", "Theta h2"]
  in  "Phase 2B 1":u16(ring)=3 items=["X", "Y", "R", "Theta", "Frequency", "Noise", "Xh1", "Yh1", "Rh1", "Theta h1", "Xh2", "Yh2", "Rh2", "Theta h2"]
  out "Vab_2/mV":cluster{dbl[], dbl[]}(graph)={[0.09999999999999998, 0.12, 0.14, 0.16000000000000003, 0.17999999999999994, 0.19999999999999996, 0.21999999999999997, 0.24, 0.26, 0.28, 0.29999999999999993, 0.31999999999999995, 0.33999999999999997, 0.36, 0.38, 0.4, 0.42000000000000004, 0.43999999999999995, 0.45999999999999996, 0.48, 0.5, 0.52, 0.54, 0.56, 0.5800000000000001, 0.6, 0.62, 0.64, 0.6599999999999999, 0.6799999999999999, 0.7, 0.72, 0.74, 0.76, 0.78, 0.8, 0.8200000000000001, 0.84, 0.86, 0.88, 0.9, 0.92, 0.94, 0.96, 0.98, 1.0, 0.98, 0.96, 0.94, 0.92, 0.9, 0.88, 0.86, 0.84, 0.82, 0.8, 0.78, 0.76, 0.74, 0.72, 0.7, 0.6799999999999999, 0.66, 0.64, 0.62, 0.6, 0.58, 0.56, 0.54, 0.52, 0.5, 0.48, 0.45999999999999996, 0.44000000000000006, 0.42000000000000004, 0.4, 0.38, 0.36, 0.33999999999999997, 0.32, 0.30000000000000004, 0.28, 0.26, 0.24000000000000002, 0.22, 0.2, 0.18, 0.16, 0.14, 0.12000000000000001, 0.1, 0.09999999999999998, 0.12, 0.14, 0.16000000000000003, 0.17999999999999994, 0.19999999999999996, 0.21999999999999997, 0.24, 0.26, 0.28, 0.29999999999999993, 0.31999999999999995, 0.33999999999999997, 0.36, 0.38, 0.4, 0.42000000000000004, 0.43999999999999995, 0.45999999999999996, 0.48, 0.5, 0.52, 0.54, 0.56, 0.5800000000000001, 0.6, 0.62, 0.64, 0.6599999999999999, 0.6799999999999999, 0.7, 0.72, 0.74, 0.76, 0.78, 0.8, 0.8200000000000001, 0.84, 0.86, 0.88, 0.9, 0.92, 0.94, 0.96, 0.98, 1.0, 0.98, 0.96, 0.94, 0.92, 0.9, 0.88, 0.86, 0.84, 0.82, 0.8, 0.78, 0.76, 0.74, 0.72, 0.7, 0.6799999999999999, 0.66, 0.64, 0.62, 0.6, 0.58, 0.56, 0.54, 0.52, 0.5, 0.48, 0.45999999999999996, 0.44000000000000006, 0.42000000000000004, 0.4, 0.38, 0.36, 0.33999999999999997, 0.32, 0.30000000000000004, 0.28, 0.26, 0.24000000000000002, 0.22, 0.2, 0.18, 0.16, 0.14, 0.12000000000000001, 0.1], [0.41484297470806686, 0.49493546480043765, 0.5756299750895625, 0.65422962835786, 0.7330948233404262, 0.8139118343157201, 0.8929573341649203, 0.9712489593687404, 1.050257506906536, 1.1290618918453497, 1.2078902562606806, 1.285513279347725, 1.3594124837103052, 1.4427700967411636, 1.521115950761339, 1.5981546581739174, 1.6764422344174124, 1.7542564427084308, 1.8317260261062935, 1.9086880231415269, 1.9871520283257933, 2.062992038473203, 2.141190454399677, 2.2183201860573347, 2.295152045046516, 2.3714296068722502, 2.453083556466876, 2.526947108694858, 2.6014507759793273, 2.6773785164461623, 2.7553708773349785, 2.830959374673886, 2.908247529647836, 2.9831597660889666, 3.0586188130688474, 3.1343412124058743, 3.211074054882647, 3.2854333757739522, 3.362561541061358, 3.4370695911213334, 3.5124629844941744, 3.585945157791819, 3.661377683414448, 3.736568846134733, 3.8111518534810287, 3.875138695157801, 3.7959169824084174, 3.723895390872345, 3.6476856347119657, 3.572085724830787, 3.4982535122674796, 3.4217482661701117, 3.34680394536362, 3.2698261058413864, 3.196716824702422, 3.1195889750840307, 3.0435199934022674, 2.9691737121993436, 2.893060466349757, 2.815601251551684, 2.739460062855177, 2.6629768718746356, 2.587280814270321, 2.511763335805597, 2.433967713381551, 2.3566558956813144, 2.28159346868964, 2.2035333879050496, 2.1263267611570114, 2.047127375477458, 1.9706664568435, 1.891842645293161, 1.8135414954701174, 1.7377472462375398, 1.6593393524050657, 1.5814072706550528, 1.5054324494258289, 1.5904194971722239, 1.3375674961879955, 1.2600356826723336, 1.1823148619124095, 1.105557280493995, 1.026820160339296, 0.9485883746446329, 0.8692031318003061, 0.790869363534512, 0.7117978610139974, 0.6334168304460623, 0.5550795469057512, 0.47459182993613663, 0.37445179632959436, 0.405723989118416, 0.4845256320791325, 0.5641778406577294, 0.6423915747280513, 0.7217785818528762, 0.7995138646773673, 0.8775931266674061, 0.9567548088253074, 1.0338895840229254, 1.11172955985341, 1.1913781080722214, 1.2687942787699376, 1.337515533906143, 1.4242461025259914, 1.5005662845216459, 1.5770196011124886, 1.6552798314299182, 1.73259048945942, 1.8083510047400835, 1.8854339412893666, 1.96327549749382, 2.0375359167171463, 2.1150524895505303, 2.193022045170706, 2.2695416013346708, 2.344420648387712, 2.42109225731397, 2.4978559926473936, 2.5727511527498943, 2.6514156542669087, 2.7253673526114075, 2.7999497653558203, 2.875941835156512, 2.9521016899697696, 3.026888385389616, 3.1013641745632303, 3.178360975778151, 3.253076836038171, 3.32820811117078, 3.403149990907622, 3.478521295172941, 3.5521862924151604, 3.626086330437451, 3.701393769265117, 3.77516270813167, 3.8375323885382353, 3.7630487471727294, 3.6887866349689564, 3.6135011523832867, 3.539159069967253, 3.464403070247352, 3.388647606252283, 3.3144088015166737, 3.2412277684080797, 3.16587618054626, 3.091048895785437, 3.0154512577305392, 2.9415608440853416, 2.864872309462221, 2.7896077237038717, 2.714045412239261, 2.6378164241441153, 2.5615012175479603, 2.4865480093667824, 2.410619473285794, 2.334072262579441, 2.2574185090389234, 2.181839533796144, 2.1040361606925386, 2.0283804083449954, 1.9527952239845678, 1.8744605849213996, 1.7956791565395904, 1.7180748042983611, 1.641141462886408, 1.5626630133255561, 1.4876592996286764, 1.5061717932978584, 1.3221523818118703, 1.2447278209568204, 1.1692629075898042, 1.0914348209506244, 1.0136318684472372, 0.9358271324526373, 0.8577874577033563, 0.781081879214504, 0.7027024372975224, 0.6248595920777948, 0.5459610082442521, 0.46724047807290975, 0.46724047807290975]}
  out "phase Vab_2":dbl=0.00041662413928722134
  out "phase Vab_2":cluster{dbl[], dbl[]}(graph)={[0.09999999999999998, 0.12, 0.14, 0.16000000000000003, 0.17999999999999994, 0.19999999999999996, 0.21999999999999997, 0.24, 0.26, 0.28, 0.29999999999999993, 0.31999999999999995, 0.33999999999999997, 0.36, 0.38, 0.4, 0.42000000000000004, 0.43999999999999995, 0.45999999999999996, 0.48, 0.5, 0.52, 0.54, 0.56, 0.5800000000000001, 0.6, 0.62, 0.64, 0.6599999999999999, 0.6799999999999999, 0.7, 0.72, 0.74, 0.76, 0.78, 0.8, 0.8200000000000001, 0.84, 0.86, 0.88, 0.9, 0.92, 0.94, 0.96, 0.98, 1.0, 0.98, 0.96, 0.94, 0.92, 0.9, 0.88, 0.86, 0.84, 0.82, 0.8, 0.78, 0.76, 0.74, 0.72, 0.7, 0.6799999999999999, 0.66, 0.64, 0.62, 0.6, 0.58, 0.56, 0.54, 0.52, 0.5, 0.48, 0.45999999999999996, 0.44000000000000006, 0.42000000000000004, 0.4, 0.38, 0.36, 0.33999999999999997, 0.32, 0.30000000000000004, 0.28, 0.26, 0.24000000000000002, 0.22, 0.2, 0.18, 0.16, 0.14, 0.12000000000000001, 0.1, 0.09999999999999998, 0.12, 0.14, 0.16000000000000003, 0.17999999999999994, 0.19999999999999996, 0.21999999999999997, 0.24, 0.26, 0.28, 0.29999999999999993, 0.31999999999999995, 0.33999999999999997, 0.36, 0.38, 0.4, 0.42000000000000004, 0.43999999999999995, 0.45999999999999996, 0.48, 0.5, 0.52, 0.54, 0.56, 0.5800000000000001, 0.6, 0.62, 0.64, 0.6599999999999999, 0.6799999999999999, 0.7, 0.72, 0.74, 0.76, 0.78, 0.8, 0.8200000000000001, 0.84, 0.86, 0.88, 0.9, 0.92, 0.94, 0.96, 0.98, 1.0, 0.98, 0.96, 0.94, 0.92, 0.9, 0.88, 0.86, 0.84, 0.82, 0.8, 0.78, 0.76, 0.74, 0.72, 0.7, 0.6799999999999999, 0.66, 0.64, 0.62, 0.6, 0.58, 0.56, 0.54, 0.52, 0.5, 0.48, 0.45999999999999996, 0.44000000000000006, 0.42000000000000004, 0.4, 0.38, 0.36, 0.33999999999999997, 0.32, 0.30000000000000004, 0.28, 0.26, 0.24000000000000002, 0.22, 0.2, 0.18, 0.16, 0.14, 0.12000000000000001, 0.1], [0.00041662413928722134, 0.0004965340984944219, 0.0005772122930365349, 0.0006557866814989885, 0.0007346710882456997, 0.0008155196799592574, 0.0008946635825651629, 0.0009727973705783476, 0.0010517312159807435, 0.001130558816622925, 0.0012094288742935913, 0.0012871895757558653, 0.0013599138307394142, 0.0014444746119866383, 0.0015226620934262929, 0.0015997686385838053, 0.001678101846934105, 0.0017558350085036096, 0.0018332577425914376, 0.0019102060752449277, 0.00198890854041113, 0.0020646656541167523, 0.0021428131740823557, 0.002219906352550648, 0.0022964524768372173, 0.002372986569172244, 0.0024555649400488633, 0.002528600301946239, 0.0026029324383869358, 0.002678819074674399, 0.002757078896076804, 0.002832541838640954, 0.0029101074104581825, 0.0029847172182425547, 0.0030601706371869456, 0.003135949174907637, 0.0032126466357683377, 0.0032868412765393847, 0.0033641990503374803, 0.0034386512322428543, 0.003514052085894783, 0.003587419763104087, 0.003663068003977296, 0.0037381887247362883, 0.0038129030341692285, 0.0038735699392995434, 0.0037976407696913863, 0.0037222156926721346, 0.003646062824165148, 0.0035703722593558285, 0.0034965864066133895, 0.003419989512826952, 0.0033451786687171267, 0.0032681352070463646, 0.003195164012614235, 0.003117833985843309, 0.0030418538575051625, 0.002967689970016326, 0.002891693668786285, 0.0028138108784215347, 0.0027375796509897837, 0.0026613568283931728, 0.002585705490864972, 0.002510170370602529, 0.002432335999270111, 0.0023548778663956093, 0.0022800219292722626, 0.0022018161972396414, 0.0021246490348139488, 0.0020455117176168282, 0.001968950438941788, 0.001890203793441763, 0.0018117456127197198, 0.0017360356865505785, 0.0016577259938267718, 0.0015799346064337473, 0.0015041987758266325, 0.001623543849333546, 0.0013359331615684807, 0.0012584811754691025, 0.0011808437633327846, 0.0011039325904912093, 0.001025046004557354, 0.0009469352937393286, 0.0008673588311775115, 0.0007892306137792021, 0.0007100334758760659, 0.0006317888303707224, 0.0005534424214581255, 0.00047284929175636723, 0.00036657894177415063, 0.0004072916893019786, 0.00048610459030511003, 0.0005659041279296239, 0.0006440596190959337, 0.0007235947559758895, 0.0008011937636369669, 0.0008791390724947436, 0.0009584989636302482, 0.0010355832706191075, 0.0011131864061023843, 0.0011933645695701802, 0.0012705361045698665, 0.0013374059205799615, 0.001426145071516011, 0.0015021759736507166, 0.0015785828252983269, 0.0016569990060811516, 0.0017342100097986254, 0.0018099813629986333, 0.0018868241395258271, 0.0019647962106564983, 0.0020390103486243537, 0.0021166435005883022, 0.002194591967032686, 0.002271002089891192, 0.0023458863690512767, 0.002422571824471677, 0.0024994333719393757, 0.0025742773834777, 0.0026498161402082345, 0.0027268765880292607, 0.0028016328451467877, 0.0028774515669155827, 0.0029537155104540913, 0.0030286663849686353, 0.003102841460345407, 0.0031799882924257858, 0.0032547709117558624, 0.00332963803575483, 0.003404920971582629, 0.003480128886241681, 0.0035538391658988993, 0.003627749045167766, 0.003702934073537857, 0.0037767260923387397, 0.003835836485959453, 0.0037614974433019615, 0.003687144649920443, 0.00361181275586003, 0.0035377997943400264, 0.003462699921649067, 0.0033869348716172587, 0.0033128608833372527, 0.0032397309143703096, 0.003164103705066053, 0.003089582168522298, 0.0030138765518761407, 0.0029399526697735856, 0.002863154251323821, 0.002788103091056089, 0.002712300983394243, 0.002636227818602749, 0.0025597821607451026, 0.002484737803973982, 0.0024089777640904537, 0.002332593347965706, 0.002259093390973955, 0.0021803216012019353, 0.002102215395194003, 0.0020268698310267974, 0.0019511420364369141, 0.0018728044353045746, 0.0017936837305290096, 0.0017162847886273674, 0.0016396459326942186, 0.0015609954962311017, 0.001486379946346497, 0.0015279111360180834, 0.0013204730653924139, 0.0012430117929804016, 0.0011678191344663955, 0.0010897560389874598, 0.0010118908664464795, 0.0009342498217453273, 0.0008562029047293179, 0.0007796310043839651, 0.0007010627615340637, 0.000623225095225132, 0.0005442177459152283, 0.0004653444282152289, 0.0004653444282152289]}
  in  "path2 (folder + filename)":string="G:\\My Drive\\Opticool\\Measurement\\NLH\\f dependence\\TaI28_A1215_B1211"
  out "phase Vaa_1":cluster{dbl[], dbl[]}(graph)={[0.09999999999999998, 0.12, 0.14, 0.16000000000000003, 0.17999999999999994, 0.19999999999999996, 0.21999999999999997, 0.24, 0.26, 0.28, 0.29999999999999993, 0.31999999999999995, 0.33999999999999997, 0.36, 0.38, 0.4, 0.42000000000000004, 0.43999999999999995, 0.45999999999999996, 0.48, 0.5, 0.52, 0.54, 0.56, 0.5800000000000001, 0.6, 0.62, 0.64, 0.6599999999999999, 0.6799999999999999, 0.7, 0.72, 0.74, 0.76, 0.78, 0.8, 0.8200000000000001, 0.84, 0.86, 0.88, 0.9, 0.92, 0.94, 0.96, 0.98, 1.0, 0.98, 0.96, 0.94, 0.92, 0.9, 0.88, 0.86, 0.84, 0.82, 0.8, 0.78, 0.76, 0.74, 0.72, 0.7, 0.6799999999999999, 0.66, 0.64, 0.62, 0.6, 0.58, 0.56, 0.54, 0.52, 0.5, 0.48, 0.45999999999999996, 0.44000000000000006, 0.42000000000000004, 0.4, 0.38, 0.36, 0.33999999999999997, 0.32, 0.30000000000000004, 0.28, 0.26, 0.24000000000000002, 0.22, 0.2, 0.18, 0.16, 0.14, 0.12000000000000001, 0.1, 0.09999999999999998, 0.12, 0.14, 0.16000000000000003, 0.17999999999999994, 0.19999999999999996, 0.21999999999999997, 0.24, 0.26, 0.28, 0.29999999999999993, 0.31999999999999995, 0.33999999999999997, 0.36, 0.38, 0.4, 0.42000000000000004, 0.43999999999999995, 0.45999999999999996, 0.48, 0.5, 0.52, 0.54, 0.56, 0.5800000000000001, 0.6, 0.62, 0.64, 0.6599999999999999, 0.6799999999999999, 0.7, 0.72, 0.74, 0.76, 0.78, 0.8, 0.8200000000000001, 0.84, 0.86, 0.88, 0.9, 0.92, 0.94, 0.96, 0.98, 1.0, 0.98, 0.96, 0.94, 0.92, 0.9, 0.88, 0.86, 0.84, 0.82, 0.8, 0.78, 0.76, 0.74, 0.72, 0.7, 0.6799999999999999, 0.66, 0.64, 0.62, 0.6, 0.58, 0.56, 0.54, 0.52, 0.5, 0.48, 0.45999999999999996, 0.44000000000000006, 0.42000000000000004, 0.4, 0.38, 0.36, 0.33999999999999997, 0.32, 0.30000000000000004, 0.28, 0.26, 0.24000000000000002, 0.22, 0.2, 0.18, 0.16, 0.14, 0.12000000000000001, 0.1], [-0.1824400805609028, -0.18620433705902234, -0.2074751866736631, -0.22048063824950095, -0.22047014246081958, -0.2300001296482231, -0.23287754743998496, -0.24188605535554847, -0.24591538885188613, -0.2434472644799872, -0.24833923811565173, -0.25411872341860003, -0.26444456459859533, -0.2619852721400308, -0.2742809482344235, -0.2820086843663061, -0.28948396597840464, -0.29431454014791514, -0.30511254887637074, -0.3023014407241319, -0.3138274759143691, -0.3167636987582855, -0.3271582978935714, -0.324156455799124, -0.33651766644825004, -0.32999415030036117, -0.340858757532962, -0.33995966795622434, -0.344067624465512, -0.33801117825139626, -0.35033121127627015, -0.35779242991058025, -0.3562051177756105, -0.36139845721348407, -0.36606913783893347, -0.3659287575316707, -0.3712330082810784, -0.3748286745814472, -0.3785468496969955, -0.38421449496876814, -0.3869060728271091, -0.38922359471622414, -0.39271302352950677, -0.3949191737506116, -0.3993053101908427, -0.4033411503160675, -0.40561313617255224, -0.4076928783469804, -0.40988483421837135, -0.41094600247326724, -0.41254782942079427, -0.4178783769698777, -0.4164123887065159, -0.4191424159689901, -0.4254257831640434, -0.4246139012765321, -0.42790708426597723, -0.4282253343779655, -0.4292333181762629, -0.43473770604637973, -0.4350114658796154, -0.43893077437586203, -0.4394238686704557, -0.4410748697639758, -0.43838749624520873, -0.4435638901330389, -0.4453569769694282, -0.4467559522897841, -0.44616855657936955, -0.46076800140399526, -0.4550426392295967, -0.46341621675125255, -0.457471583491227, -0.45618994424010983, -0.452034675954941, -0.44818090486838447, -0.4438510759695939, -0.4345494571436224, -0.4471106255669583, -0.45099797755962745, -0.45080571535776615, -0.444869652209429, -0.45718915636224605, -0.46056424408068297, -0.46174782318576113, -0.4571709053205698, -0.46348910589756037, -0.4576640113936262, -0.44006285954219876, -0.4451961696760861, -0.4576576986384441, 0.26496831420163713, 0.2708933996335404, 0.2607347775660769, 0.2638838394416675, 0.26335491960266355, 0.2667872653568081, 0.26724337621568234, 0.26712176300768065, 0.2674620670917106, 0.26893079605958264, 0.2634684269928984, 0.26688111172431317, 0.2615259463397597, 0.2599566061270767, 0.2587746765167529, 0.2509445030721138, 0.2400527662998992, 0.2472333124835985, 0.23609704048746583, 0.2427272655431036, 0.23868111177798204, 0.24226079662598493, 0.2459713068688641, 0.24330647431824132, 0.2391472550064376, 0.23921115735354728, 0.2422326323818404, 0.23723019726007682, 0.23601541641080917, 0.23345434046895291, 0.23268569112904278, 0.23577729593921473, 0.23167995698161947, 0.23327746294717322, 0.23063894872245516, 0.23154633329610547, 0.22513484660716596, 0.2290475052624073, 0.2251983912674212, 0.22402542728511404, 0.22423160420174187, 0.22168151443084588, 0.21886329602048632, 0.21834051098628726, 0.21530942329509534, 0.21371313846834483, 0.20975631012996382, 0.20809544521095277, 0.20079612815574133, 0.1966692106554847, 0.1946595090625177, 0.19289471208438408, 0.18618988037907386, 0.18236323133097213, 0.1779413544023653, 0.17313238016181692, 0.16793529533957924, 0.16325647765948104, 0.16083007661392346, 0.1528416868389246, 0.14735827537889915, 0.14621060581222697, 0.1437499595822624, 0.1355342087456147, 0.13027536391362968, 0.12884570291702852, 0.12151592365705081, 0.11264163782982568, 0.10846461320285561, 0.10286447326412881, 0.08736645483771163, 0.09229955450292285, 0.08883362313107258, 0.09016286648002067, 0.08967970461206556, 0.09222927679488681, 0.08699903997834149, 0.0743482565687268, 0.08278851387008015, 0.07952793113240596, 0.07030622973359793, 0.06938740966650045, 0.06376458777381558, 0.059071115139876215, 0.033929348307887526, 0.047883061468017234, 0.04436657416341557, 0.02841159836568414, -0.007485553969095675, 0.010041020552594208, 0.015825498267562944]}
  out "Vaa_1/mV":cluster{dbl[], dbl[]}(graph)={[0.09999999999999998, 0.12, 0.14, 0.16000000000000003, 0.17999999999999994, 0.19999999999999996, 0.21999999999999997, 0.24, 0.26, 0.28, 0.29999999999999993, 0.31999999999999995, 0.33999999999999997, 0.36, 0.38, 0.4, 0.42000000000000004, 0.43999999999999995, 0.45999999999999996, 0.48, 0.5, 0.52, 0.54, 0.56, 0.5800000000000001, 0.6, 0.62, 0.64, 0.6599999999999999, 0.6799999999999999, 0.7, 0.72, 0.74, 0.76, 0.78, 0.8, 0.8200000000000001, 0.84, 0.86, 0.88, 0.9, 0.92, 0.94, 0.96, 0.98, 1.0, 0.98, 0.96, 0.94, 0.92, 0.9, 0.88, 0.86, 0.84, 0.82, 0.8, 0.78, 0.76, 0.74, 0.72, 0.7, 0.6799999999999999, 0.66, 0.64, 0.62, 0.6, 0.58, 0.56, 0.54, 0.52, 0.5, 0.48, 0.45999999999999996, 0.44000000000000006, 0.42000000000000004, 0.4, 0.38, 0.36, 0.33999999999999997, 0.32, 0.30000000000000004, 0.28, 0.26, 0.24000000000000002, 0.22, 0.2, 0.18, 0.16, 0.14, 0.12000000000000001, 0.1, 0.09999999999999998, 0.12, 0.14, 0.16000000000000003, 0.17999999999999994, 0.19999999999999996, 0.21999999999999997, 0.24, 0.26, 0.28, 0.29999999999999993, 0.31999999999999995, 0.33999999999999997, 0.36, 0.38, 0.4, 0.42000000000000004, 0.43999999999999995, 0.45999999999999996, 0.48, 0.5, 0.52, 0.54, 0.56, 0.5800000000000001, 0.6, 0.62, 0.64, 0.6599999999999999, 0.6799999999999999, 0.7, 0.72, 0.74, 0.76, 0.78, 0.8, 0.8200000000000001, 0.84, 0.86, 0.88, 0.9, 0.92, 0.94, 0.96, 0.98, 1.0, 0.98, 0.96, 0.94, 0.92, 0.9, 0.88, 0.86, 0.84, 0.82, 0.8, 0.78, 0.76, 0.74, 0.72, 0.7, 0.6799999999999999, 0.66, 0.64, 0.62, 0.6, 0.58, 0.56, 0.54, 0.52, 0.5, 0.48, 0.45999999999999996, 0.44000000000000006, 0.42000000000000004, 0.4, 0.38, 0.36, 0.33999999999999997, 0.32, 0.30000000000000004, 0.28, 0.26, 0.24000000000000002, 0.22, 0.2, 0.18, 0.16, 0.14, 0.12000000000000001, 0.1], [0.642747805090089, 0.8506714432721977, 1.0173060818714441, 1.2229309774435462, 1.4398052740385832, 1.6571604268655313, 1.8800682738279855, 2.1205229610573633, 2.3737477912149285, 2.610312084361251, 2.8824398871126573, 3.214844948414449, 3.5905478072507657, 3.68656018942935, 3.9701698255073707, 4.241369700631268, 4.5349229580110535, 4.845433394069812, 5.139220614981783, 5.443215161966466, 5.742985580575448, 6.056337209404007, 6.365640083224472, 6.6756615932047785, 7.000578266667725, 7.325321562970057, 7.6205530212241825, 8.002406772611815, 8.330513362273553, 8.645063054674486, 8.987986071850369, 9.330047844586572, 9.685680187050494, 10.02635388058023, 10.364786131492085, 10.747654988038457, 11.132697098702184, 11.45238139412986, 11.800030350530724, 12.172748348430723, 12.521419344071901, 12.883079617145308, 13.256237531926761, 13.642877389052936, 14.031029177937134, 14.154170631374713, 13.781093030485572, 13.412008715669305, 13.033043284278321, 12.670764017971468, 12.277206173862071, 11.93274686621078, 11.471075677789734, 10.957071844193804, 10.8488429523072, 10.498911849543918, 10.15108550170916, 9.810042295103866, 9.457451996078749, 9.105619614940883, 8.787443506276368, 8.400964503993315, 8.106943840961943, 7.7729423249798995, 7.416392250112723, 7.099834032071507, 6.788805804309607, 6.496411457909396, 6.152753680934036, 5.866985821166226, 5.541846288999364, 5.247441178291986, 4.95207104850739, 4.654154141306654, 4.363508191248042, 4.082869431312876, 3.740564083352161, 3.507583022566204, 3.24288608448896, 2.9733831802403214, 2.610012372445045, 2.2231816708621923, 2.2139342382795295, 1.9699340958501144, 1.737709799211624, 1.5121632627218005, 1.2807616607487784, 1.079370652364624, 0.8840873727837274, 0.6979403060954856, 0.4177953600291347, 0.6452084594720114, 0.8200154775096731, 1.0098769186648195, 1.2135918347436323, 1.4405192685464512, 1.647091951582843, 1.8745994762567157, 2.1357666925001233, 2.382239153025236, 2.6322170087630288, 2.8914332755652414, 3.160659022276161, 3.4186047756603957, 3.711626965899161, 3.9872638143453583, 4.275490941012708, 4.564698272136846, 4.852290275863386, 5.147380320255485, 5.451021703184579, 5.751690956130852, 6.060210325279208, 6.373935110345776, 6.697802605429004, 7.013441550431839, 7.343386559703698, 7.665838414521016, 8.00596454896485, 8.340142321277463, 8.67275068614269, 9.017117811369562, 9.359492655977412, 9.677231095133486, 10.036269464425706, 10.39630070487511, 10.743492683564595, 11.093227201555951, 11.458594222655682, 11.82737089138121, 12.209845630398204, 12.546264400162054, 12.907989420145253, 13.295159446638122, 13.65763771415592, 14.03700581181816, 14.163924614898415, 13.781446204647485, 13.418135044325874, 13.05090074099853, 12.682975409675834, 12.31405680210821, 11.937390046019505, 11.579228486737383, 11.225724673329402, 10.870986998844845, 10.52065195177664, 10.15165843102961, 9.807195160669117, 9.470691346796169, 9.140594288481557, 8.774963974357764, 8.43969687573813, 8.111277170841245, 7.784462699559414, 7.453869403813787, 7.13677972356102, 6.809006546432683, 6.481698972277128, 6.175554222851094, 5.732769353988787, 5.2582806158053215, 5.251201443303944, 4.942944679066435, 4.610824399798008, 4.358026456042018, 4.071492918342776, 3.7967543027968818, 3.4968522951482304, 3.2083507458775897, 2.9637299168250126, 2.7101528739897796, 2.4407851142926633, 2.208552174815502, 1.8444214443208897, 1.5172766495788794, 1.5134451801493285, 1.2921024861767016, 0.9827681352247983, 0.7143553575394094, 0.6974920233849868, 0.4192229324423554]}
  out "Phase1B-T":cluster{dbl[], dbl[]}(graph)={[0.09999999999999998, 0.12, 0.14, 0.16000000000000003, 0.17999999999999994, 0.19999999999999996, 0.21999999999999997, 0.24, 0.26, 0.28, 0.29999999999999993, 0.31999999999999995, 0.33999999999999997, 0.36, 0.38, 0.4, 0.42000000000000004, 0.43999999999999995, 0.45999999999999996, 0.48, 0.5, 0.52, 0.54, 0.56, 0.5800000000000001, 0.6, 0.62, 0.64, 0.6599999999999999, 0.6799999999999999, 0.7, 0.72, 0.74, 0.76, 0.78, 0.8, 0.8200000000000001, 0.84, 0.86, 0.88, 0.9, 0.92, 0.94, 0.96, 0.98, 1.0, 0.98, 0.96, 0.94, 0.92, 0.9, 0.88, 0.86, 0.84, 0.82, 0.8, 0.78, 0.76, 0.74, 0.72, 0.7, 0.6799999999999999, 0.66, 0.64, 0.62, 0.6, 0.58, 0.56, 0.54, 0.52, 0.5, 0.48, 0.45999999999999996, 0.44000000000000006, 0.42000000000000004, 0.4, 0.38, 0.36, 0.33999999999999997, 0.32, 0.30000000000000004, 0.28, 0.26, 0.24000000000000002, 0.22, 0.2, 0.18, 0.16, 0.14, 0.12000000000000001, 0.1, 0.09999999999999998, 0.12, 0.14, 0.16000000000000003, 0.17999999999999994, 0.19999999999999996, 0.21999999999999997, 0.24, 0.26, 0.28, 0.29999999999999993, 0.31999999999999995, 0.33999999999999997, 0.36, 0.38, 0.4, 0.42000000000000004, 0.43999999999999995, 0.45999999999999996, 0.48, 0.5, 0.52, 0.54, 0.56, 0.5800000000000001, 0.6, 0.62, 0.64, 0.6599999999999999, 0.6799999999999999, 0.7, 0.72, 0.74, 0.76, 0.78, 0.8, 0.8200000000000001, 0.84, 0.86, 0.88, 0.9, 0.92, 0.94, 0.96, 0.98, 1.0, 0.98, 0.96, 0.94, 0.92, 0.9, 0.88, 0.86, 0.84, 0.82, 0.8, 0.78, 0.76, 0.74, 0.72, 0.7, 0.6799999999999999, 0.66, 0.64, 0.62, 0.6, 0.58, 0.56, 0.54, 0.52, 0.5, 0.48, 0.45999999999999996, 0.44000000000000006, 0.42000000000000004, 0.4, 0.38, 0.36, 0.33999999999999997, 0.32, 0.30000000000000004, 0.28, 0.26, 0.24000000000000002, 0.22, 0.2, 0.18, 0.16, 0.14, 0.12000000000000001, 0.1], [-82.66180934000548, -82.31663084351848, -81.28479556546662, -79.7285481269931, -79.83639483259351, -78.93022910188402, -77.76625064717406, -76.98286963793183, -76.30338483017276, -75.3329388876501, -74.15487675040681, -73.63994904293313, -72.00519230686407, -70.98865992787974, -69.78260547877099, -68.46981695953193, -66.41471110064296, -63.727467767510845, -61.73122732271541, -61.24012537063011, -59.77241233729169, -59.030277248937296, -56.32614878714115, -57.18800917801351, -53.39789571974181, -55.19003110626528, -51.23804867909978, -51.22826215768248, -49.514500690914105, -50.67271589509581, -43.07642582076291, -40.06328619340774, -39.413931632303274, -36.99977134971505, -31.875606579535646, -26.93659911458971, -22.688622325891004, -17.47048958759187, -14.55798847194743, -7.800864266519929, -4.642690556338657, 3.1570021137885886, 6.743601613738856, 12.668918306151308, 15.557308911850686, 19.39129625930486, 16.203829879225133, 10.32861439888182, 5.749810917509566, 2.412215442972166, -2.888120750486132, -8.209518420307703, -14.820777936162278, -21.676053478160163, -23.863319970090707, -30.005001219141867, -33.765325812818304, -37.243570341822476, -37.988577230185754, -39.26402694104284, -42.46660284275954, -44.26966926749856, -47.57652334591893, -49.77965414220169, -51.573521417528696, -51.38633213706511, -53.74494347874671, -55.63422993694276, -58.674421986492135, -55.28995428563481, -59.243847142139956, -59.57511295356316, -63.47272556219632, -64.30799549280343, -68.42564447387139, -69.7311498344494, -71.71228843513832, -67.97845829178313, -72.72803989909792, -73.49252836592719, -74.15205281239723, -75.60919344462434, -76.64116785682184, -77.18615474869783, -78.27027561582172, -79.41768714667208, -79.45498048291918, -80.51961759154237, -81.32678467910651, -82.15025719060743, -82.07695958163313, -80.97148376112338, -81.73367989926514, -82.2177271257415, -82.96021047197411, -83.12064957002124, -84.49372585630113, -84.89497821728332, -85.85558799965068, -85.88106250810583, -86.77872322581511, -87.52581883144892, -87.18065787222568, -87.46951374559205, -87.31390048464922, -87.18864448576649, -86.66015032013496, -84.0135075502205, -86.93089402951506, -81.74464303991269, -86.14437894131098, -85.03345928384263, -89.13043658333932, -91.5954053174322, -91.29931288858792, -90.7934199455879, -94.59175759378834, -94.45326908568144, -100.12158624921842, -106.4868531449388, -117.77759677088582, -135.1393078684343, -168.06146887636237, 167.7477102916197, 149.34050397760709, 144.61946841096645, 138.20865205098738, 125.40183798569917, 125.17018640838492, 122.78991468391216, 120.38872207649936, 118.5661866824494, 117.5405373345621, 116.85853307464477, 115.77080570479272, 114.97137169127969, 114.66846354976944, 115.3675399395928, 119.32208614565397, 118.51400904244693, 119.22046446865468, 121.67591835901922, 123.20652651582668, 123.86929349448201, 128.28845984708235, 134.30507853160242, 139.45006622986256, 151.6086208278811, -107.56333518699628, -163.6867171884482, -137.01215371738678, -116.01894372473107, -107.09438253303601, -97.65679803851754, -96.18143050414834, -90.79515260675086, -89.83493074136871, -87.54496647365337, -84.35502024233972, -81.88265379920226, -85.15265070101468, -80.98527581110758, -83.80983909524252, -84.2891551215024, -85.71568576094415, -86.83813790486641, -88.92766155649683, -88.07306642626565, -86.00726023904289, -89.18743694730172, -88.30535287076512, -87.88229818087834, -87.23362091021392, -86.50942390208522, -85.66223203092242, -85.21369815775334, -84.9823863237167, -84.36261035155313, -83.6463610027926, -82.4453476280448, -81.4361173947326, -82.33301916423876]}
  out "R1B-T":cluster{dbl[], dbl[]}(graph)={[0.09999999999999998, 0.12, 0.14, 0.16000000000000003, 0.17999999999999994, 0.19999999999999996, 0.21999999999999997, 0.24, 0.26, 0.28, 0.29999999999999993, 0.31999999999999995, 0.33999999999999997, 0.36, 0.38, 0.4, 0.42000000000000004, 0.43999999999999995, 0.45999999999999996, 0.48, 0.5, 0.52, 0.54, 0.56, 0.5800000000000001, 0.6, 0.62, 0.64, 0.6599999999999999, 0.6799999999999999, 0.7, 0.72, 0.74, 0.76, 0.78, 0.8, 0.8200000000000001, 0.84, 0.86, 0.88, 0.9, 0.92, 0.94, 0.96, 0.98, 1.0, 0.98, 0.96, 0.94, 0.92, 0.9, 0.88, 0.86, 0.84, 0.82, 0.8, 0.78, 0.76, 0.74, 0.72, 0.7, 0.6799999999999999, 0.66, 0.64, 0.62, 0.6, 0.58, 0.56, 0.54, 0.52, 0.5, 0.48, 0.45999999999999996, 0.44000000000000006, 0.42000000000000004, 0.4, 0.38, 0.36, 0.33999999999999997, 0.32, 0.30000000000000004, 0.28, 0.26, 0.24000000000000002, 0.22, 0.2, 0.18, 0.16, 0.14, 0.12000000000000001, 0.1, 0.09999999999999998, 0.12, 0.14, 0.16000000000000003, 0.17999999999999994, 0.19999999999999996, 0.21999999999999997, 0.24, 0.26, 0.28, 0.29999999999999993, 0.31999999999999995, 0.33999999999999997, 0.36, 0.38, 0.4, 0.42000000000000004, 0.43999999999999995, 0.45999999999999996, 0.48, 0.5, 0.52, 0.54, 0.56, 0.5800000000000001, 0.6, 0.62, 0.64, 0.6599999999999999, 0.6799999999999999, 0.7, 0.72, 0.74, 0.76, 0.78, 0.8, 0.8200000000000001, 0.84, 0.86, 0.88, 0.9, 0.92, 0.94, 0.96, 0.98, 1.0, 0.98, 0.96, 0.94, 0.92, 0.9, 0.88, 0.86, 0.84, 0.82, 0.8, 0.78, 0.76, 0.74, 0.72, 0.7, 0.6799999999999999, 0.66, 0.64, 0.62, 0.6, 0.58, 0.56, 0.54, 0.52, 0.5, 0.48, 0.45999999999999996, 0.44000000000000006, 0.42000000000000004, 0.4, 0.38, 0.36, 0.33999999999999997, 0.32, 0.30000000000000004, 0.28, 0.26, 0.24000000000000002, 0.22, 0.2, 0.18, 0.16, 0.14, 0.12000000000000001, 0.1], [316.1348134738238, 340.0235154994667, 354.1002916001893, 367.58122947136815, 382.2662398891261, 388.8666611052246, 395.6423083273966, 403.37181356744827, 401.6536954469682, 390.3590369897094, 359.6569497817645, 374.57146797080196, 372.5306768228112, 367.7894019960707, 356.52042410715154, 358.3299828076831, 361.59496082792543, 336.7287792474283, 327.44509675934984, 328.1030235287556, 325.04779088287677, 319.06253858115565, 310.07116578685833, 298.67052393743216, 278.9962169036786, 270.0567927740529, 253.86523538886448, 253.72161300226227, 253.89633174401126, 247.92613470780717, 226.63319690832571, 222.67802272728687, 205.3247379927167, 215.53787621196108, 206.21068679937042, 190.81186004910316, 188.28418623179647, 179.28277237182965, 190.66344688409185, 184.98578405446898, 187.820361568895, 184.7173204473596, 197.44571685549525, 201.95014669567954, 226.71773096958216, 212.23672323083602, 201.14902429789572, 199.28231216775697, 197.9108390248407, 189.1174925305517, 185.4629274770452, 189.7402863786704, 203.39893140150687, 192.49162285301563, 198.75225235772282, 214.20578545098957, 227.31586933267354, 243.06766207202028, 234.30664586303763, 248.22756277895627, 238.15194935848763, 256.1566038603338, 261.80083946921735, 259.08562024489777, 269.2536317714124, 279.4383765950696, 285.2061387223687, 292.06243820623547, 302.7824759087376, 313.2014900152133, 331.22299761588926, 321.9697630978831, 328.9356733253529, 332.3411328057169, 335.5806789248518, 350.6060213753251, 335.9450989972192, 258.4950231069081, 374.7524949037159, 372.985322666713, 371.3410076270717, 380.67871626044655, 379.17056727729573, 381.43798184355586, 376.8390546332374, 368.3879496715273, 353.46912857900924, 335.55701160987013, 322.1393630779168, 301.97302598538323, 107.64812887089077, 241.93933037663646, 254.37196425752379, 267.45775870329277, 285.3375853150402, 286.45460008034155, 294.7024036773022, 299.11245027190114, 290.9038528963541, 286.9702276882903, 278.27824285751143, 272.2574121946683, 264.6379808315789, 278.9978411241572, 241.50252940072644, 238.0299614882674, 221.71195110604998, 203.49986479307194, 191.253400229917, 174.9815616122018, 173.60020300797387, 166.29082962596615, 164.97406346297737, 132.73457269733854, 131.47287744225392, 118.63516872186786, 98.39428881503297, 82.78783717889927, 85.88797198677958, 54.061701803949745, 48.34182407142167, 36.87982302029799, 33.356813182563165, 50.925736586905806, 49.919820325028255, 62.85971599534453, 91.83020467730896, 122.7682224804518, 131.7925806410895, 146.8140396204712, 179.06850725151153, 186.1554441185651, 201.48778418147933, 237.8668358106517, 253.01324363045296, 274.54910987207717, 254.4586090434102, 241.84398281388718, 218.17752369790944, 200.77101355437557, 174.6601549107784, 171.49974346503728, 140.61902116351555, 121.16159743870375, 104.82967469134786, 74.90693888273206, 60.98319362378109, 54.469994873584945, 39.844811915936894, 50.132594625303476, 46.65112333623544, 45.614430723728674, 75.30693162203784, 94.5695515271732, 105.36887560543917, 119.39050015573234, 119.34478545352546, 130.27597703050594, 153.74728577990925, 169.2056413332065, 188.5932097101584, 183.37918365458341, 186.48539068407132, 206.5956892010012, 215.16752894451383, 226.5593973332589, 238.81272173790737, 230.51619001179427, 238.41100556579718, 282.55068074769775, 282.66266065938316, 288.5968637167715, 296.3668715131189, 297.8265247247114, 306.7629938367472, 306.7288301983777, 296.82192676085987, 284.9537995639815, 256.3091460874779, 250.86528759389608, 242.31848432116743, 71.96866428410856]}
  out "phase 1B":dbl=-82.66180934000548
  in  "Phase 1B":u16(ring)=9 items=["X", "Y", "R", "Theta", "Frequency", "Noise", "Xh1", "Yh1", "Rh1", "Theta h1", "Xh2", "Yh2", "Rh2", "Theta h2"]
  out "phase Vaa_1":dbl=-0.1824400805609028
  in  "Phase 1A":u16(ring)=3 items=["X", "Y", "R", "Theta", "Frequency", "Noise", "Xh1", "Yh1", "Rh1", "Theta h1", "Xh2", "Yh2", "Rh2", "Theta h2"]
  out "Vaa_1(1w)/mV":dbl=0.642747805090089
  in  "T Clear Plot 1A":bool
  in  "Parameter 1A":u16(ring)=2 items=["X", "Y", "R", "Theta", "Frequency", "Noise", "Xh1", "Yh1", "Rh1", "Theta h1", "Xh2", "Yh2", "Rh2", "Theta h2"]
  out "para1B Measurement":dbl=316.1348134738238
  in  "T Clear Plot 1B":bool
  in  "Parameter 1B":u16(ring)=8 items=["X", "Y", "R", "Theta", "Frequency", "Noise", "Xh1", "Yh1", "Rh1", "Theta h1", "Xh2", "Yh2", "Rh2", "Theta h2"]
  out "phase Vaa_2":cluster{dbl[], dbl[]}(graph)={[0.09999999999999998, 0.12, 0.14, 0.16000000000000003, 0.17999999999999994, 0.19999999999999996, 0.21999999999999997, 0.24, 0.26, 0.28, 0.29999999999999993, 0.31999999999999995, 0.33999999999999997, 0.36, 0.38, 0.4, 0.42000000000000004, 0.43999999999999995, 0.45999999999999996, 0.48, 0.5, 0.52, 0.54, 0.56, 0.5800000000000001, 0.6, 0.62, 0.64, 0.6599999999999999, 0.6799999999999999, 0.7, 0.72, 0.74, 0.76, 0.78, 0.8, 0.8200000000000001, 0.84, 0.86, 0.88, 0.9, 0.92, 0.94, 0.96, 0.98, 1.0, 0.98, 0.96, 0.94, 0.92, 0.9, 0.88, 0.86, 0.84, 0.82, 0.8, 0.78, 0.76, 0.74, 0.72, 0.7, 0.6799999999999999, 0.66, 0.64, 0.62, 0.6, 0.58, 0.56, 0.54, 0.52, 0.5, 0.48, 0.45999999999999996, 0.44000000000000006, 0.42000000000000004, 0.4, 0.38, 0.36, 0.33999999999999997, 0.32, 0.30000000000000004, 0.28, 0.26, 0.24000000000000002, 0.22, 0.2, 0.18, 0.16, 0.14, 0.12000000000000001, 0.1, 0.09999999999999998, 0.12, 0.14, 0.16000000000000003, 0.17999999999999994, 0.19999999999999996, 0.21999999999999997, 0.24, 0.26, 0.28, 0.29999999999999993, 0.31999999999999995, 0.33999999999999997, 0.36, 0.38, 0.4, 0.42000000000000004, 0.43999999999999995, 0.45999999999999996, 0.48, 0.5, 0.52, 0.54, 0.56, 0.5800000000000001, 0.6, 0.62, 0.64, 0.6599999999999999, 0.6799999999999999, 0.7, 0.72, 0.74, 0.76, 0.78, 0.8, 0.8200000000000001, 0.84, 0.86, 0.88, 0.9, 0.92, 0.94, 0.96, 0.98, 1.0, 0.98, 0.96, 0.94, 0.92, 0.9, 0.88, 0.86, 0.84, 0.82, 0.8, 0.78, 0.76, 0.74, 0.72, 0.7, 0.6799999999999999, 0.66, 0.64, 0.62, 0.6, 0.58, 0.56, 0.54, 0.52, 0.5, 0.48, 0.45999999999999996, 0.44000000000000006, 0.42000000000000004, 0.4, 0.38, 0.36, 0.33999999999999997, 0.32, 0.30000000000000004, 0.28, 0.26, 0.24000000000000002, 0.22, 0.2, 0.18, 0.16, 0.14, 0.12000000000000001, 0.1], [-5.991413912020415, -5.979988859369443, -5.982388623443086, -5.980295318416438, -5.965793850837737, -5.968068679612129, -5.9710260501863255, -5.973167183982061, -5.966531257382558, -5.967571133664922, -5.9684439732269485, -5.959769913788831, -5.895868536940322, -5.954204968100507, -5.950462459403328, -5.953100187140218, -5.94960882390386, -5.945828489704732, -5.943820742976437, -5.940001403354066, -5.936042234973078, -5.935139213743516, -5.933937546281608, -5.926909271247344, -5.927945518612783, -5.923762795798652, -5.918900735711605, -5.915874146935932, -5.912306214302999, -5.91053988904595, -5.909964303815219, -5.9027341102599005, -5.903942926457917, -5.898443588576786, -5.898714922760397, -5.892951750517063, -5.891021136342391, -5.886348217351724, -5.883808843715175, -5.882525339281818, -5.881730492209092, -5.875903473307953, -5.8729910282218825, -5.868915653139875, -5.868224268076747, -5.864985752187354, -5.861545641971964, -5.86066831685703, -5.8576208646387755, -5.853008151058884, -5.850848982475911, -5.848993208601273, -5.848697015168506, -5.845399711289046, -5.843934970514621, -5.839820275129557, -5.838258318310208, -5.835204937131657, -5.829686946818253, -5.8300553382237466, -5.8269555935211255, -5.825677677526842, -5.819018646754119, -5.8181658931266975, -5.8143906804193515, -5.812179897181859, -5.808659613893017, -5.808044734236645, -5.802667357978848, -5.798525274470683, -5.797371551354982, -5.795450668277172, -5.789179278275684, -5.791465625824286, -5.7865581768694625, -5.781562845953529, -5.786149794109986, -6.268149626383197, -5.781596524336152, -5.777349022758058, -5.770810436030983, -5.773144804357341, -5.76894165248712, -5.758192728068769, -5.760882926366827, -5.753783351738976, -5.763366299397214, -5.744806800502745, -5.729755579517658, -5.7203697465918975, -5.678330585215506, 0.2962179782022508, 0.30102853783776923, 0.30434136427552366, 0.30463753895168055, 0.3061556588468413, 0.3189096909661974, 0.32010391006714306, 0.31684922212248556, 0.31863328149012543, 0.33046189398707493, 0.32772153291512746, 0.3323489579786564, 0.32694089498476625, 0.3442351172100254, 0.3410102949479862, 0.3433768357680843, 0.3494681628265216, 0.3470232477992118, 0.35478584859704465, 0.3563632005448358, 0.358304892861035, 0.3636758739796684, 0.3640290395388953, 0.3688621280083869, 0.37108166486451255, 0.37610332009482134, 0.3791221498272711, 0.3790386284173557, 0.3857679299923987, 0.383604126597844, 0.3868404166541435, 0.39074252633950557, 0.3953151546039985, 0.39399353695695427, 0.39807492645600473, 0.40477616060977084, 0.4073443412571948, 0.4106134188236932, 0.4127410324214205, 0.41552545472634284, 0.4178500586141789, 0.4205224266732469, 0.4241580616379161, 0.4281151085236381, 0.43138475787024005, 0.4349853234139168, 0.4369357381485342, 0.43927781989950176, 0.44051390327695295, 0.442744590975539, 0.44583341497986095, 0.4499681830508913, 0.4497658851092662, 0.45386365513452864, 0.4567672963066025, 0.45920240562596604, 0.4601459554506014, 0.46277059225447603, 0.46541378504788017, 0.46706840143577927, 0.46970345430945193, 0.4728214811049015, 0.47779948865853994, 0.47738854774417927, 0.4805793750759251, 0.4823478855771447, 0.48337674720174145, 0.48977353867022744, 0.4940593826436265, 0.49701377380032347, 0.4975685781448026, 0.5005601010990693, 0.5036378584416799, 0.5078210196051163, 0.5069823859614064, 0.510824020515842, 0.5127618894236552, 0.6465748656245204, 0.5101022639283228, 0.5166541119287336, 0.5248320114144162, 0.5258172391242222, 0.5182788851108857, 0.5319656778616797, 0.5239262414620721, 0.5330967218845937, 0.5335679769942729, 0.5436051421284256, 0.5478577854539874, 0.5393170574632166, 0.5393170574632166]}
  out "Vaa_2/mV":cluster{dbl[], dbl[]}(graph)={[0.09999999999999998, 0.12, 0.14, 0.16000000000000003, 0.17999999999999994, 0.19999999999999996, 0.21999999999999997, 0.24, 0.26, 0.28, 0.29999999999999993, 0.31999999999999995, 0.33999999999999997, 0.36, 0.38, 0.4, 0.42000000000000004, 0.43999999999999995, 0.45999999999999996, 0.48, 0.5, 0.52, 0.54, 0.56, 0.5800000000000001, 0.6, 0.62, 0.64, 0.6599999999999999, 0.6799999999999999, 0.7, 0.72, 0.74, 0.76, 0.78, 0.8, 0.8200000000000001, 0.84, 0.86, 0.88, 0.9, 0.92, 0.94, 0.96, 0.98, 1.0, 0.98, 0.96, 0.94, 0.92, 0.9, 0.88, 0.86, 0.84, 0.82, 0.8, 0.78, 0.76, 0.74, 0.72, 0.7, 0.6799999999999999, 0.66, 0.64, 0.62, 0.6, 0.58, 0.56, 0.54, 0.52, 0.5, 0.48, 0.45999999999999996, 0.44000000000000006, 0.42000000000000004, 0.4, 0.38, 0.36, 0.33999999999999997, 0.32, 0.30000000000000004, 0.28, 0.26, 0.24000000000000002, 0.22, 0.2, 0.18, 0.16, 0.14, 0.12000000000000001, 0.1, 0.09999999999999998, 0.12, 0.14, 0.16000000000000003, 0.17999999999999994, 0.19999999999999996, 0.21999999999999997, 0.24, 0.26, 0.28, 0.29999999999999993, 0.31999999999999995, 0.33999999999999997, 0.36, 0.38, 0.4, 0.42000000000000004, 0.43999999999999995, 0.45999999999999996, 0.48, 0.5, 0.52, 0.54, 0.56, 0.5800000000000001, 0.6, 0.62, 0.64, 0.6599999999999999, 0.6799999999999999, 0.7, 0.72, 0.74, 0.76, 0.78, 0.8, 0.8200000000000001, 0.84, 0.86, 0.88, 0.9, 0.92, 0.94, 0.96, 0.98, 1.0, 0.98, 0.96, 0.94, 0.92, 0.9, 0.88, 0.86, 0.84, 0.82, 0.8, 0.78, 0.76, 0.74, 0.72, 0.7, 0.6799999999999999, 0.66, 0.64, 0.62, 0.6, 0.58, 0.56, 0.54, 0.52, 0.5, 0.48, 0.45999999999999996, 0.44000000000000006, 0.42000000000000004, 0.4, 0.38, 0.36, 0.33999999999999997, 0.32, 0.30000000000000004, 0.28, 0.26, 0.24000000000000002, 0.22, 0.2, 0.18, 0.16, 0.14, 0.12000000000000001, 0.1], [0.18632339845641088, 0.2180539698872459, 0.25241196456840415, 0.2844895388360828, 0.3169658228684725, 0.35057613389142656, 0.3841505708456905, 0.4165075657163915, 0.4497324347592481, 0.48263398453018214, 0.5158605106735383, 0.5481327079667071, 0.5725448709146299, 0.6167837002807911, 0.6493587902757586, 0.6826125442201453, 0.7155872700368674, 0.7473574010923758, 0.7814665589473558, 0.8140703814932442, 0.8481175982194981, 0.8810211619871762, 0.9149262622144942, 0.9468545689938606, 0.9794040216134471, 1.0140018482343858, 1.0496505956154731, 1.0808255938395674, 1.1126844106664722, 1.1454370124974906, 1.1805273931380338, 1.2132325611299923, 1.2473493790491412, 1.2792171358617372, 1.3129804877983526, 1.345444518685826, 1.3796286687285215, 1.412357473084738, 1.446974510586548, 1.4790952017141745, 1.5127871605610737, 1.5455261666126474, 1.5793347786816687, 1.613554773713094, 1.6471183813536898, 1.6422328409352513, 1.6074630363094247, 1.5741494982941924, 1.5402444464251572, 1.5072396508833497, 1.474465962040132, 1.4399817871924805, 1.407820462181446, 1.3738617029632125, 1.3415230231430726, 1.306559443593991, 1.2746431458873704, 1.2425040679954167, 1.2093652997895734, 1.173976443491854, 1.140930088952352, 1.1093966137167175, 1.0751921055874127, 1.04307969058256, 1.0093778882869293, 0.9743205405386689, 0.9433863356197126, 0.9090997748976345, 0.8742252607426345, 0.8424574958908633, 0.8104107480554651, 0.7763698379254955, 0.7419387506111457, 0.7098599529176591, 0.6774469864797925, 0.6453081111880057, 0.6208088830001338, 0.939662173005609, 0.5440622425928409, 0.5113410393153434, 0.4788182888945911, 0.4462731873662959, 0.4121101974998194, 0.37944770137410755, 0.344964802685002, 0.31289294169243037, 0.2789052860737111, 0.24717680584662316, 0.21475973631967107, 0.17862812894197475, 0.07972397261858725, 0.18506701968816802, 0.21779531711160638, 0.2523718903779747, 0.28506358527337455, 0.31883489263248954, 0.3509991090561582, 0.3832560171084185, 0.4181455903610921, 0.45009530297806155, 0.4821245997572151, 0.5184267960823559, 0.5489519822404973, 0.5681470778168048, 0.6174260539584709, 0.6491921490874335, 0.6816727734677531, 0.7165902686589456, 0.7484759570401541, 0.7802326193414088, 0.8135266121989251, 0.847726323857494, 0.8796943762913876, 0.9147580916083741, 0.9478979776529892, 0.9805522178170337, 1.0132931969286574, 1.0463362703623131, 1.080731857064295, 1.113332607296091, 1.1481781288397694, 1.180378551035846, 1.21345801942141, 1.2469420703229983, 1.2803110088193157, 1.3140212656296342, 1.345507381160019, 1.3808722632511479, 1.4141783046438552, 1.4472419433861585, 1.4809475047554477, 1.5135926998912965, 1.5481922106702044, 1.5799733050141351, 1.6131530697946002, 1.6472451068607057, 1.642757983124434, 1.610023940489538, 1.5757835078267703, 1.5417213694490635, 1.5090466417104498, 1.4747154622910683, 1.4408349807306726, 1.4083270161784462, 1.37575582358476, 1.3410172155530742, 1.3092413188925909, 1.2752111424928734, 1.2424181948860082, 1.2075742598177903, 1.1763781776671551, 1.1423632708039875, 1.1097343076667883, 1.0756484891031075, 1.0416824711590171, 1.0090291590430427, 0.976854056361431, 0.9436015085739112, 0.9098420550575238, 0.876008999592259, 0.8436597096422096, 0.8109735474602997, 0.776051924434362, 0.7445411588201116, 0.7098161694095696, 0.6779632714300857, 0.6435661845155277, 0.6171949206905882, 0.7901540058685572, 0.5427759584405307, 0.5099841827400041, 0.4785218785628561, 0.444318733763329, 0.4117668330229793, 0.37839278914542834, 0.34528848635429044, 0.3132130093823999, 0.27861054757485065, 0.24675596269079902, 0.21291837750636805, 0.17833823206936966, 0.17833823206936966]}
  out "Phase2B-T":cluster{dbl[], dbl[]}(graph)={[0.09999999999999998, 0.12, 0.14, 0.16000000000000003, 0.17999999999999994, 0.19999999999999996, 0.21999999999999997, 0.24, 0.26, 0.28, 0.29999999999999993, 0.31999999999999995, 0.33999999999999997, 0.36, 0.38, 0.4, 0.42000000000000004, 0.43999999999999995, 0.45999999999999996, 0.48, 0.5, 0.52, 0.54, 0.56, 0.5800000000000001, 0.6, 0.62, 0.64, 0.6599999999999999, 0.6799999999999999, 0.7, 0.72, 0.74, 0.76, 0.78, 0.8, 0.8200000000000001, 0.84, 0.86, 0.88, 0.9, 0.92, 0.94, 0.96, 0.98, 1.0, 0.98, 0.96, 0.94, 0.92, 0.9, 0.88, 0.86, 0.84, 0.82, 0.8, 0.78, 0.76, 0.74, 0.72, 0.7, 0.6799999999999999, 0.66, 0.64, 0.62, 0.6, 0.58, 0.56, 0.54, 0.52, 0.5, 0.48, 0.45999999999999996, 0.44000000000000006, 0.42000000000000004, 0.4, 0.38, 0.36, 0.33999999999999997, 0.32, 0.30000000000000004, 0.28, 0.26, 0.24000000000000002, 0.22, 0.2, 0.18, 0.16, 0.14, 0.12000000000000001, 0.1, 0.09999999999999998, 0.12, 0.14, 0.16000000000000003, 0.17999999999999994, 0.19999999999999996, 0.21999999999999997, 0.24, 0.26, 0.28, 0.29999999999999993, 0.31999999999999995, 0.33999999999999997, 0.36, 0.38, 0.4, 0.42000000000000004, 0.43999999999999995, 0.45999999999999996, 0.48, 0.5, 0.52, 0.54, 0.56, 0.5800000000000001, 0.6, 0.62, 0.64, 0.6599999999999999, 0.6799999999999999, 0.7, 0.72, 0.74, 0.76, 0.78, 0.8, 0.8200000000000001, 0.84, 0.86, 0.88, 0.9, 0.92, 0.94, 0.96, 0.98, 1.0, 0.98, 0.96, 0.94, 0.92, 0.9, 0.88, 0.86, 0.84, 0.82, 0.8, 0.78, 0.76, 0.74, 0.72, 0.7, 0.6799999999999999, 0.66, 0.64, 0.62, 0.6, 0.58, 0.56, 0.54, 0.52, 0.5, 0.48, 0.45999999999999996, 0.44000000000000006, 0.42000000000000004, 0.4, 0.38, 0.36, 0.33999999999999997, 0.32, 0.30000000000000004, 0.28, 0.26, 0.24000000000000002, 0.22, 0.2, 0.18, 0.16, 0.14, 0.12000000000000001, 0.1], [-98.48741226130407, -85.09755048216388, -96.99948068589936, -95.94917130056298, -89.0690298104169, -90.023740037216, -91.98912281092412, -94.68856376204448, -93.14459079941199, -93.62977898915707, -94.13291757175685, -95.1315276711849, -108.65877425304534, -95.54685347031007, -94.89549162980308, -94.61940547830923, -93.9284047369021, -94.05796012384204, -94.04193477600606, -93.7857744958114, -93.67621299383521, -94.29280219193741, -93.95782448872076, -94.39852972913766, -94.16916096111666, -94.04658221476681, -93.833530357928, -94.30879141361335, -93.90636408500731, -93.96141956129749, -93.85207216960832, -94.11625081624418, -93.87835077611179, -94.1093872571277, -93.62890813296762, -93.75944061541372, -93.47876140768224, -93.60051631833707, -93.32842859359373, -93.14210585940145, -93.18952378889954, -93.54660731285192, -93.37421252494617, -93.26178067655738, -93.45483394041734, -93.16308726631102, -93.28355778391108, -93.5342934399672, -93.2456466584964, -93.4722147862377, -93.33213265967348, -93.4515533050843, -93.2451624941634, -93.34942460028265, -93.57046289046848, -93.38750015493653, -93.83552871366945, -93.52603296018883, -93.99146648138026, -93.69817444703719, -94.08688476031887, -93.58762549991108, -93.98356873675554, -93.85338677495592, -93.91416606446865, -93.78639574977272, -93.75817875839637, -93.58989129453072, -94.15257562173456, -93.84438089037216, -94.2807356933119, -93.40026017099754, -94.08495483915587, -93.31763435958747, -93.88018886545656, -93.61413898179524, -95.80264889665247, -119.35213953415004, -94.39040898937762, -93.82517101481153, -94.6281639048842, -97.0082528272998, -99.37592058219784, -95.33866067040341, -104.87918363202377, -90.82311612251904, -135.34214408770208, 106.29059203934045, 93.22818339513206, -107.69548266933842, -105.07169152318605, -115.13426959273696, -76.65173861611603, 81.97517341554878, -130.41400652477506, -75.95977189100012, -95.33599378876387, -87.78037450278607, -82.69130592535264, -80.48093518232342, -77.36480685278711, -80.73451267109897, -83.81326337384016, -141.1255432963907, -80.5033100036957, -81.37642333442544, -81.65603181354031, -81.84567558781607, -81.8225191219113, -82.07422208189632, -81.57648881799574, -81.86744984501496, -81.91868468017401, -81.62572400060897, -82.00397130217348, -81.58030154498319, -81.790289573425, -81.74474743034054, -81.51487135365707, -81.06117002190568, -81.45077217920104, -81.12297716288369, -81.28720520663225, -81.59333767755197, -81.2697243134574, -81.12593521658879, -81.0479591104079, -81.13021795073074, -81.05521501570517, -81.02419510731522, -80.97806585032171, -81.02842309372883, -80.82585924366751, -81.0053832563792, -80.73107027840295, -80.97591621329357, -80.8710250070493, -80.80421389953905, -80.64613049266973, -80.67615608740603, -80.78120223216631, -80.75536338785392, -80.88604180340617, -80.49769040906111, -80.95543218338427, -80.83081659844309, -80.9866627455965, -81.09217039533341, -81.24602311474312, -81.15847848161987, -80.9294077463881, -81.38418319054031, -81.4431347211551, -81.18090346300711, -81.05094892681473, -81.31767328791253, -80.91817863758617, -80.80507002293866, -81.37807734636932, -81.29822764671961, -81.37036264468522, -80.84119633798068, -81.4480540765968, -81.26679625577748, -81.32034798340723, -81.04353357834114, -80.49519794989519, -80.7856179068421, -95.81497250485411, -83.40548393331137, -84.0894873691096, -82.72805678241757, -81.0556612858808, -82.90743956199876, -81.11858478614775, -86.44850866732271, -73.80697456064397, -82.99773126470818, -81.24727554930442, -78.06821587504194, -169.40180889243814, -169.40180889243814]}
  out "R2B-T":cluster{dbl[], dbl[]}(graph)={[0.09999999999999998, 0.12, 0.14, 0.16000000000000003, 0.17999999999999994, 0.19999999999999996, 0.21999999999999997, 0.24, 0.26, 0.28, 0.29999999999999993, 0.31999999999999995, 0.33999999999999997, 0.36, 0.38, 0.4, 0.42000000000000004, 0.43999999999999995, 0.45999999999999996, 0.48, 0.5, 0.52, 0.54, 0.56, 0.5800000000000001, 0.6, 0.62, 0.64, 0.6599999999999999, 0.6799999999999999, 0.7, 0.72, 0.74, 0.76, 0.78, 0.8, 0.8200000000000001, 0.84, 0.86, 0.88, 0.9, 0.92, 0.94, 0.96, 0.98, 1.0, 0.98, 0.96, 0.94, 0.92, 0.9, 0.88, 0.86, 0.84, 0.82, 0.8, 0.78, 0.76, 0.74, 0.72, 0.7, 0.6799999999999999, 0.66, 0.64, 0.62, 0.6, 0.58, 0.56, 0.54, 0.52, 0.5, 0.48, 0.45999999999999996, 0.44000000000000006, 0.42000000000000004, 0.4, 0.38, 0.36, 0.33999999999999997, 0.32, 0.30000000000000004, 0.28, 0.26, 0.24000000000000002, 0.22, 0.2, 0.18, 0.16, 0.14, 0.12000000000000001, 0.1, 0.09999999999999998, 0.12, 0.14, 0.16000000000000003, 0.17999999999999994, 0.19999999999999996, 0.21999999999999997, 0.24, 0.26, 0.28, 0.29999999999999993, 0.31999999999999995, 0.33999999999999997, 0.36, 0.38, 0.4, 0.42000000000000004, 0.43999999999999995, 0.45999999999999996, 0.48, 0.5, 0.52, 0.54, 0.56, 0.5800000000000001, 0.6, 0.62, 0.64, 0.6599999999999999, 0.6799999999999999, 0.7, 0.72, 0.74, 0.76, 0.78, 0.8, 0.8200000000000001, 0.84, 0.86, 0.88, 0.9, 0.92, 0.94, 0.96, 0.98, 1.0, 0.98, 0.96, 0.94, 0.92, 0.9, 0.88, 0.86, 0.84, 0.82, 0.8, 0.78, 0.76, 0.74, 0.72, 0.7, 0.6799999999999999, 0.66, 0.64, 0.62, 0.6, 0.58, 0.56, 0.54, 0.52, 0.5, 0.48, 0.45999999999999996, 0.44000000000000006, 0.42000000000000004, 0.4, 0.38, 0.36, 0.33999999999999997, 0.32, 0.30000000000000004, 0.28, 0.26, 0.24000000000000002, 0.22, 0.2, 0.18, 0.16, 0.14, 0.12000000000000001, 0.1], [0.6133845465433322, 0.7891992873692255, 0.9820259720741601, 1.4788095977027398, 1.9347727758172022, 2.6082038404531245, 3.5008033487670556, 3.873602937475328, 4.6193993253494705, 5.437657592030816, 6.551198165614536, 7.239016907806838, 12.295861493372351, 13.324461937150385, 14.426114798181716, 15.771211350139685, 16.955862863210058, 17.697469873001705, 19.461049819351196, 20.339898492904446, 22.16459308841142, 23.178961379583527, 25.08575388876785, 26.229345753205788, 28.072045074770728, 29.853331767852517, 31.282041416515796, 32.94215466665539, 34.46668610226706, 36.011837509226865, 37.85841304676145, 39.83160518057286, 41.60421982486919, 43.11401692830019, 45.08293599391493, 47.312195111831755, 49.311496539634156, 51.55976755693881, 53.81394999403427, 55.17218166494065, 57.37829378555016, 59.294751628291216, 61.881312264594484, 63.8959505446495, 66.04331396782155, 64.56244767730811, 62.001420243383755, 60.21169829439571, 58.17578815519384, 56.04489245005349, 54.43165681712508, 52.46517602661579, 50.5782834111363, 47.87001447419264, 46.3535400486456, 44.24363245655938, 42.75043747609463, 40.963442162326, 38.92396312231167, 37.333064984215824, 35.64651504557411, 34.23163776052319, 32.040468770247564, 30.097662639710858, 28.747284763527574, 27.276398076087354, 25.375163957292934, 23.82498158743163, 22.078682673103206, 20.659617278540072, 19.27199768540878, 18.100532530657834, 17.010146745962597, 15.619847723046895, 14.25582510590062, 13.367101573859946, 14.822428863247614, 91.60869614321851, 4.2464914835029495, 3.5595374627225476, 3.0417953645012643, 2.664219016905471, 1.9359518766765778, 1.4812900148542822, 0.8699070640950887, 0.5601838655860433, 0.3099093038821114, 0.31949267123408726, 0.2373958734000886, 0.20966166391244134, 0.8723119611449491, 0.10760603318337188, 0.2181956034531614, 0.19200700168245038, 0.3971943943507168, 0.4081922327588383, 1.0623970413910977, 1.741542820123643, 2.0115035007873017, 3.052454311460798, 3.478516373492089, 4.412543240604152, 4.704969429990765, 6.194960595619982, 11.144314555727789, 11.992839969795865, 13.043308753515626, 14.631596193274525, 15.806989389411985, 17.135536679831706, 18.478756709759644, 19.708769572894983, 21.47975066174653, 22.783862745260514, 24.49894207715948, 25.685710734701527, 27.386804799356526, 29.291133551182277, 30.9894672813123, 32.6087034699189, 34.6024623572124, 36.28391562412697, 38.20155235510096, 39.7372332034121, 41.413942752708905, 43.58419176439716, 44.98565030199216, 47.45590930798401, 49.16743586398944, 51.02531330264897, 53.01814308454968, 55.21644975954524, 56.988785876369626, 59.501015790176794, 61.4465806395587, 63.67042697135304, 62.099974510235235, 59.885047150968234, 57.81520707623663, 55.474278584971934, 53.28031557786307, 51.2510770660829, 49.63376413035412, 47.54720723357401, 45.79155780678471, 44.214300495365066, 42.044457382030814, 40.5891097822193, 38.48745729194203, 36.604911538905675, 34.761966274169616, 33.07984061273967, 31.39589420087976, 29.260331572092213, 27.83564682221339, 25.896616872815233, 24.591125983055136, 23.27098844010322, 21.995197533953544, 19.858689579898062, 18.5523121235052, 17.18994474247456, 16.453582578269305, 16.307654981096277, 14.774342711309783, 13.369325275819989, 12.51632559126757, 11.981824500635627, 24.32528943829096, 6.723647162462803, 5.55766397020405, 4.9364684873381, 4.068239311047243, 3.3002843357024645, 2.3681172661367365, 1.6024199347042798, 1.1077235423701095, 0.6678780214627806, 0.4212116645420182, 0.040622381402178234, 0.14030823760254163, 0.14030823760254163]}
  out "phase 2B":dbl=-98.48741226130407
  in  "Phase 2B":u16(ring)=9 items=["X", "Y", "R", "Theta", "Frequency", "Noise", "Xh1", "Yh1", "Rh1", "Theta h1", "Xh2", "Yh2", "Rh2", "Theta h2"]
  out "phase Vaa_2":dbl=-5.991413912020415
  in  "Phase 2A":u16(ring)=3 items=["X", "Y", "R", "Theta", "Frequency", "Noise", "Xh1", "Yh1", "Rh1", "Theta h1", "Xh2", "Yh2", "Rh2", "Theta h2"]
  out "Vaa_2(1w)/mV":dbl=0.18632339845641088
  in  "T Clear Plot 2A":bool
  in  "Parameter 2A":u16(ring)=2 items=["X", "Y", "R", "Theta", "Frequency", "Noise", "Xh1", "Yh1", "Rh1", "Theta h1", "Xh2", "Yh2", "Rh2", "Theta h2"]
  out "para2B Measurement":dbl=0.6133845465433322
  in  "T Clear Plot 2B":bool
  in  "Parameter 2B":u16(ring)=8 items=["X", "Y", "R", "Theta", "Frequency", "Noise", "Xh1", "Yh1", "Rh1", "Theta h1", "Xh2", "Yh2", "Rh2", "Theta h2"]
  in  "Save data or not":bool=TRUE
  in  "path1 (folder + filename)":string="G:\\My Drive\\Opticool\\Measurement\\NLH\\f dependence\\TaI27_A34_B38"
  in  "V Loop#":i32=1
  in  "Two Devices ?":bool=TRUE
  in  "LOCKIN2 address":refnum<visa-resource-name>="COM4"
  in  "2B Input Connection (0: Single-Ended)":u16(ring)=1 items=["Single-Ended Voltage", "Differential Voltage", "1 MOhm Current Gain", "100 MOhm Current Gain"]
  in  "2B harmonic 1":u8=2
  in  "2B harmonic 2":u8=3
  in  "2B reference Manual Phase":dbl
  in  "auto phase 2B":bool=TRUE
  in  "2B Sample time (s)":dbl=0.001 min=0.001 max=100.0 step=0.001
  in  "2B Sensitivity":u16(ring)=26 items=["1 nV/fA", "2 nV/fA", "5 nV/fA", "10 nV/fA", "20 nV/fA", "50 nV/fA", "100 nV/fA", "200 nV/fA", "500 nV/fA", "1 uV/pA", "2 uV/pA", "5 uV/pA", "10 uV/pA", "20 uV/pA", "50 uV/pA", "100 uV/pA", "200 uV/pA", "500 uV/pA", "1 mV/nA", "2 mV/nA", "5 mV/nA", "10 mV/nA", "20 mV/nA", "50 mV/nA", "100 mV/nA", "200 mV/nA", "500 mV/nA", "1 V/uA"]
  in  "Enable Sync Filter 2B (open when f<200Hz)":bool
  in  "2B Time Constant":u8(ring)=9 items=["10 us", "30 us", "100 us", "300 us", "1 ms", "3 ms", "10 ms", "30 ms", "100 ms", "300 ms", "1 s", "3 s", "10 s", "30 s", "100 s", "300 s", "1 ks", "3 ks"]
  in  "2B Reference Source":u8(ring)=3 items=["External", "Internal", "Internal Sweep", "Channel-A"]
  in  "2B Low Pass Filter Slope":u8(ring)=2 items=["6 dB/oct", "12 dB/oct", "18 db/oct", "24 dB/oct"]
  in  "2A Input Connection (0: Single-Ended)":u16(ring)=1 items=["Single-Ended Voltage", "Differential Voltage", "1 MOhm Current Gain", "100 MOhm Current Gain"]
  in  "2A harmonic 1":u8=2
  in  "2A harmonic 2":u8=3
  in  "2A reference Manual Phase":dbl
  in  "auto phase 2A":bool=TRUE
  in  "2A Reference Source":u8(ring)=1 items=["External", "Internal", "Internal Sweep"]
  in  "2A Sample time (s)":dbl=0.001 min=0.001 max=100.0 step=0.001
  in  "2A Time Constant":u8(ring)=9 items=["10 us", "30 us", "100 us", "300 us", "1 ms", "3 ms", "10 ms", "30 ms", "100 ms", "300 ms", "1 s", "3 s", "10 s", "30 s", "100 s", "300 s", "1 ks", "3 ks"]
  in  "Enable Sync Filter 2A (open when f<200Hz)":bool
  in  "2A Sensitivity":u16(ring)=26 items=["1 nV/fA", "2 nV/fA", "5 nV/fA", "10 nV/fA", "20 nV/fA", "50 nV/fA", "100 nV/fA", "200 nV/fA", "500 nV/fA", "1 uV/pA", "2 uV/pA", "5 uV/pA", "10 uV/pA", "20 uV/pA", "50 uV/pA", "100 uV/pA", "200 uV/pA", "500 uV/pA", "1 mV/nA", "2 mV/nA", "5 mV/nA", "10 mV/nA", "20 mV/nA", "50 mV/nA", "100 mV/nA", "200 mV/nA", "500 mV/nA", "1 V/uA"]
  in  "2A Low Pass Filter Slope":u8(ring)=2 items=["6 dB/oct", "12 dB/oct", "18 db/oct", "24 dB/oct"]
  out "Sine voltage T":dbl=0.09999999999999998 format="%#_13g"
  in  "Initialization?":bool
  in  "V Step(mV)":i32=20
  out "V Loop Run T":i32
  in  "High Value (V)":dbl=1.5
  in  "Low Value (V)":dbl=0.1
  in  "System Stablization (s)":dbl=0.5 format="%#_13g"
  in  "LOCKIN1 address":refnum<visa-resource-name>="COM3"
  in  "B Input Connection (0: Single-Ended)":u16(ring)=1 items=["Single-Ended Voltage", "Differential Voltage", "1 MOhm Current Gain", "100 MOhm Current Gain"]
  in  "B harmonic 1":u8=2
  in  "B harmonic 2":u8=3
  in  "B reference Manual Phase":dbl
  in  "auto phase B":bool=TRUE
  in  "B Sample time (s)":dbl=0.001 min=0.001 max=100.0 step=0.001
  in  "B Sensitivity":u16(ring)=26 items=["1 nV/fA", "2 nV/fA", "5 nV/fA", "10 nV/fA", "20 nV/fA", "50 nV/fA", "100 nV/fA", "200 nV/fA", "500 nV/fA", "1 uV/pA", "2 uV/pA", "5 uV/pA", "10 uV/pA", "20 uV/pA", "50 uV/pA", "100 uV/pA", "200 uV/pA", "500 uV/pA", "1 mV/nA", "2 mV/nA", "5 mV/nA", "10 mV/nA", "20 mV/nA", "50 mV/nA", "100 mV/nA", "200 mV/nA", "500 mV/nA", "1 V/uA"]
  in  "Enable Sync Filter B (open when f<200Hz)":bool
  in  "B Time Constant":u8(ring)=9 items=["10 us", "30 us", "100 us", "300 us", "1 ms", "3 ms", "10 ms", "30 ms", "100 ms", "300 ms", "1 s", "3 s", "10 s", "30 s", "100 s", "300 s", "1 ks", "3 ks"]
  in  "B Reference Source":u8(ring)=3 items=["External", "Internal", "Internal Sweep", "Channel-A"]
  in  "B Low Pass Filter Slope":u8(ring)=2 items=["6 dB/oct", "12 dB/oct", "18 db/oct", "24 dB/oct"]
  in  "A Input Connection (0: Single-Ended)":u16(ring)=1 items=["Single-Ended Voltage", "Differential Voltage", "1 MOhm Current Gain", "100 MOhm Current Gain"]
  in  "A harmonic 1":u8=2
  in  "A harmonic 2":u8=3
  in  "A reference Manual Phase":dbl
  in  "auto phase A":bool=TRUE
  in  "A Reference Source":u8(ring)=1 items=["External", "Internal", "Internal Sweep"]
  in  "A Sample time (s)":dbl=0.001 min=0.001 max=100.0 step=0.001
  in  "A Time Constant":u8(ring)=9 items=["10 us", "30 us", "100 us", "300 us", "1 ms", "3 ms", "10 ms", "30 ms", "100 ms", "300 ms", "1 s", "3 s", "10 s", "30 s", "100 s", "300 s", "1 ks", "3 ks"]
  in  "Enable Sync Filter A (open when f<200Hz)":bool
  in  "A Sensitivity":u16(ring)=26 items=["1 nV/fA", "2 nV/fA", "5 nV/fA", "10 nV/fA", "20 nV/fA", "50 nV/fA", "100 nV/fA", "200 nV/fA", "500 nV/fA", "1 uV/pA", "2 uV/pA", "5 uV/pA", "10 uV/pA", "20 uV/pA", "50 uV/pA", "100 uV/pA", "200 uV/pA", "500 uV/pA", "1 mV/nA", "2 mV/nA", "5 mV/nA", "10 mV/nA", "20 mV/nA", "50 mV/nA", "100 mV/nA", "200 mV/nA", "500 mV/nA", "1 V/uA"]
  in  "A Low Pass Filter Slope":u8(ring)=2 items=["6 dB/oct", "12 dB/oct", "18 db/oct", "24 dB/oct"]
  # "Mesurement 1T"
  # "Ri_1 Measurement"
  # "Lock-in Setting"
  # "Channel 1A"
  # "Sweep Setting"
  # "Channel 1B"
  # "Channel 2A"
  # "Current Measurement"
  # "Channel 2B"
  # "Mesurement 2T"
  # "Ri_2 Measurement"
  # "Sweep frequency Mesurement"
  # "Temprature and Field Setting"
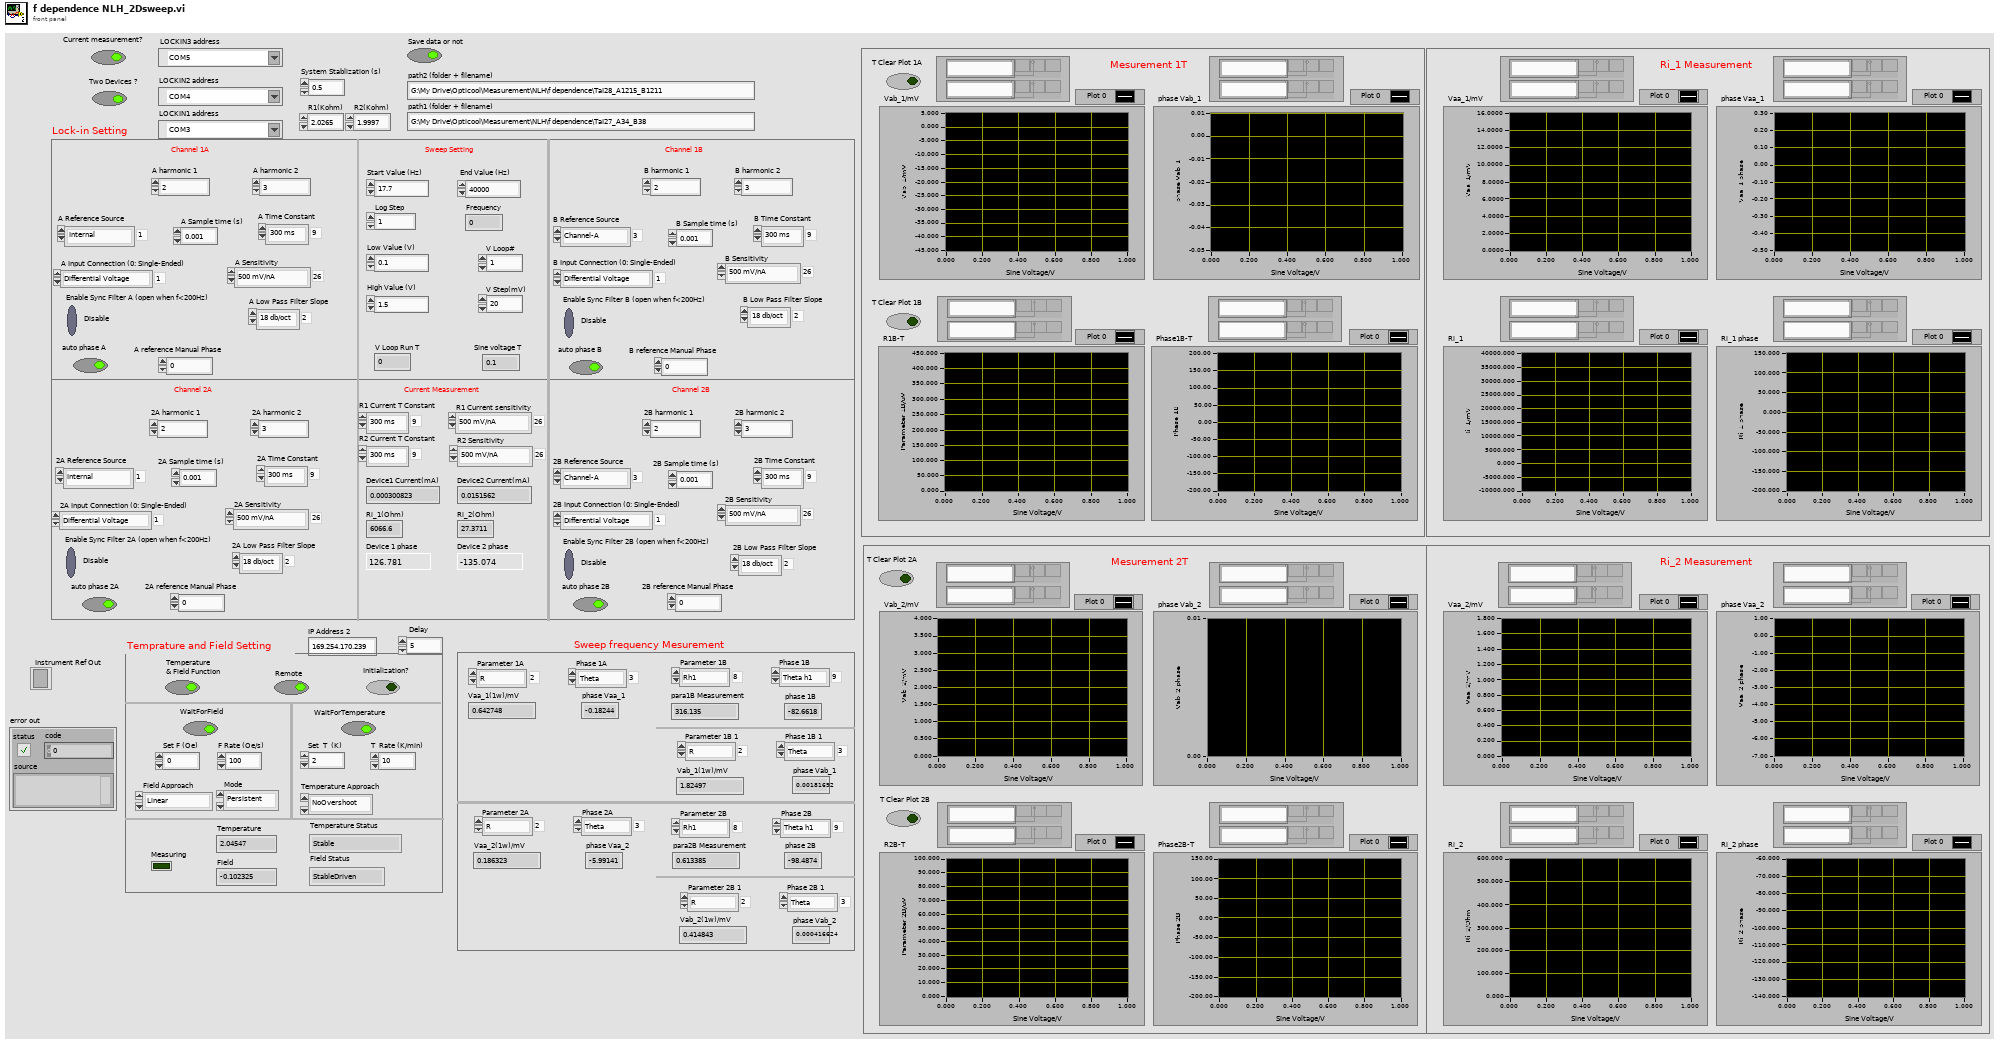
[diagram p1: front panel]
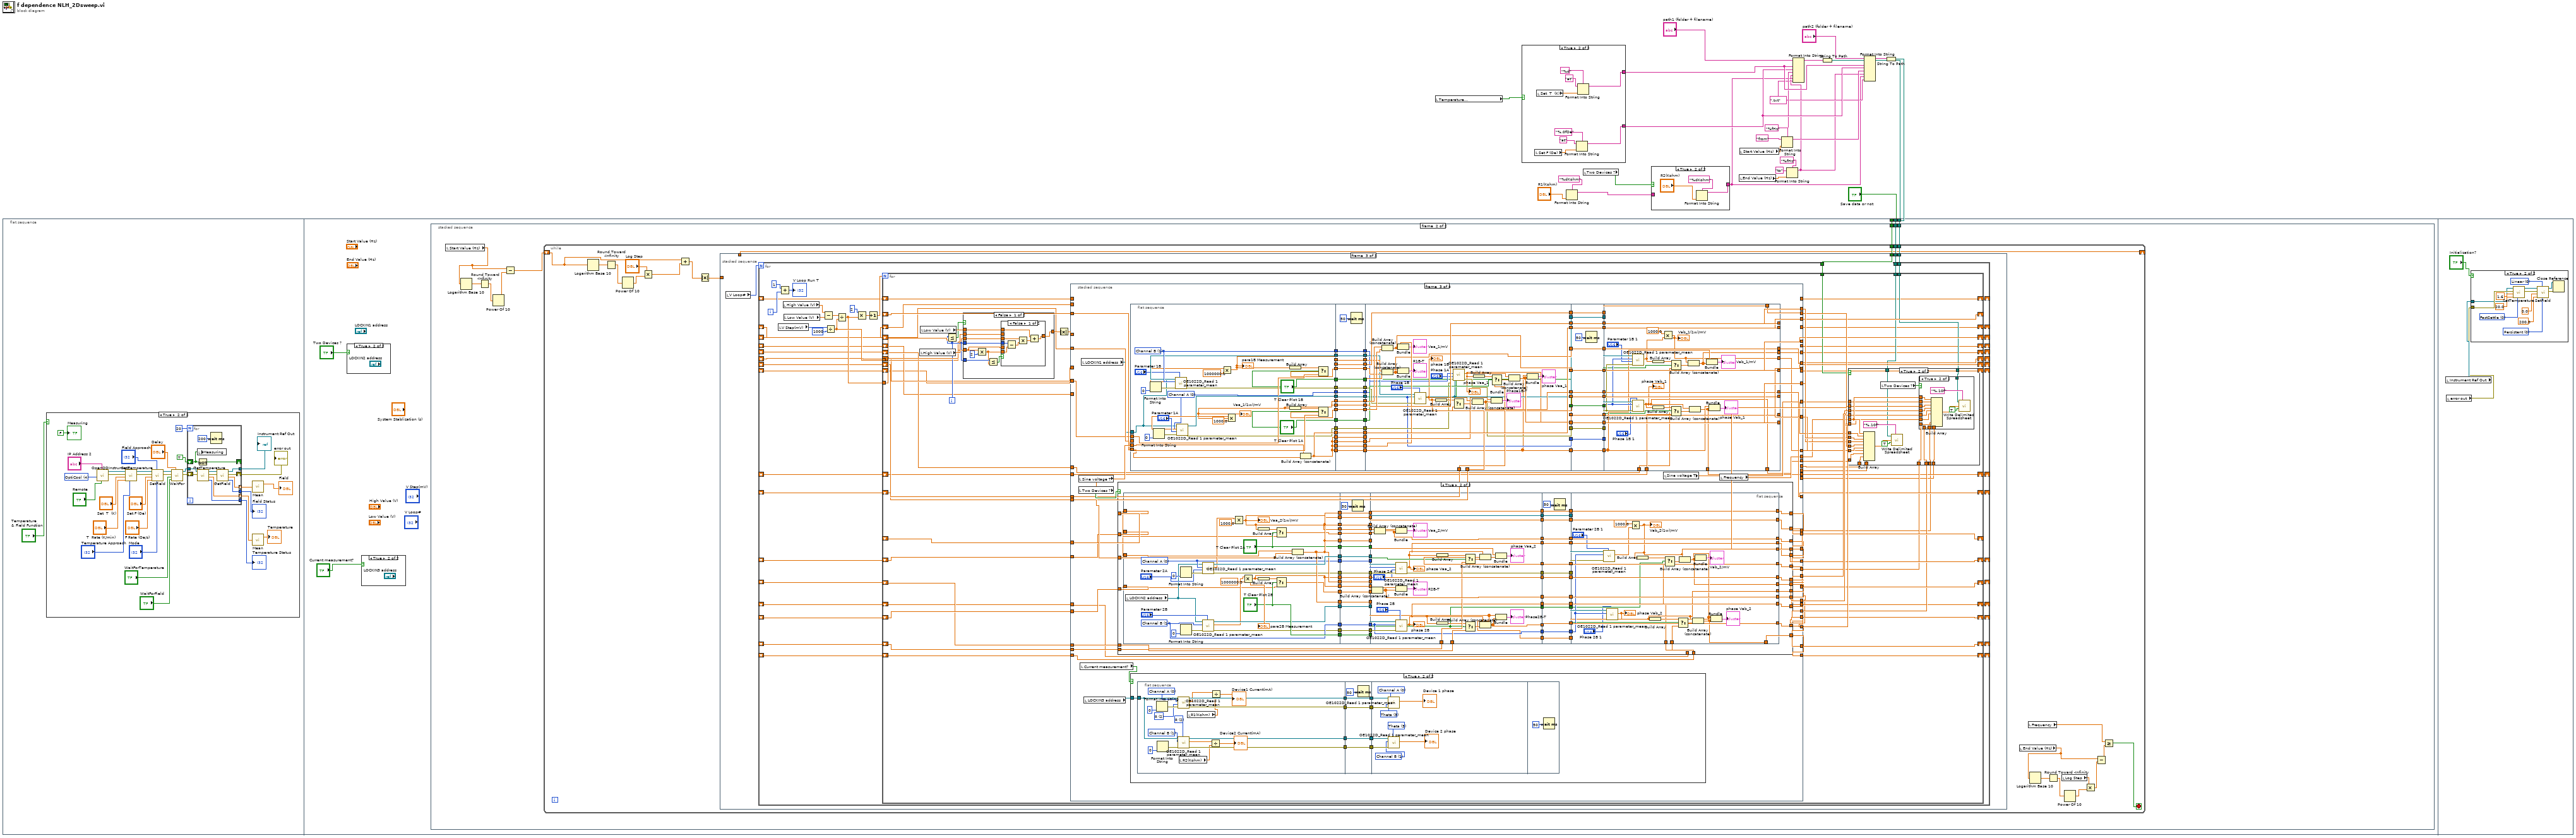
[diagram p0: block diagram]
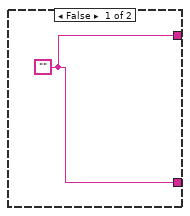
[diagram p3: hidden frame]
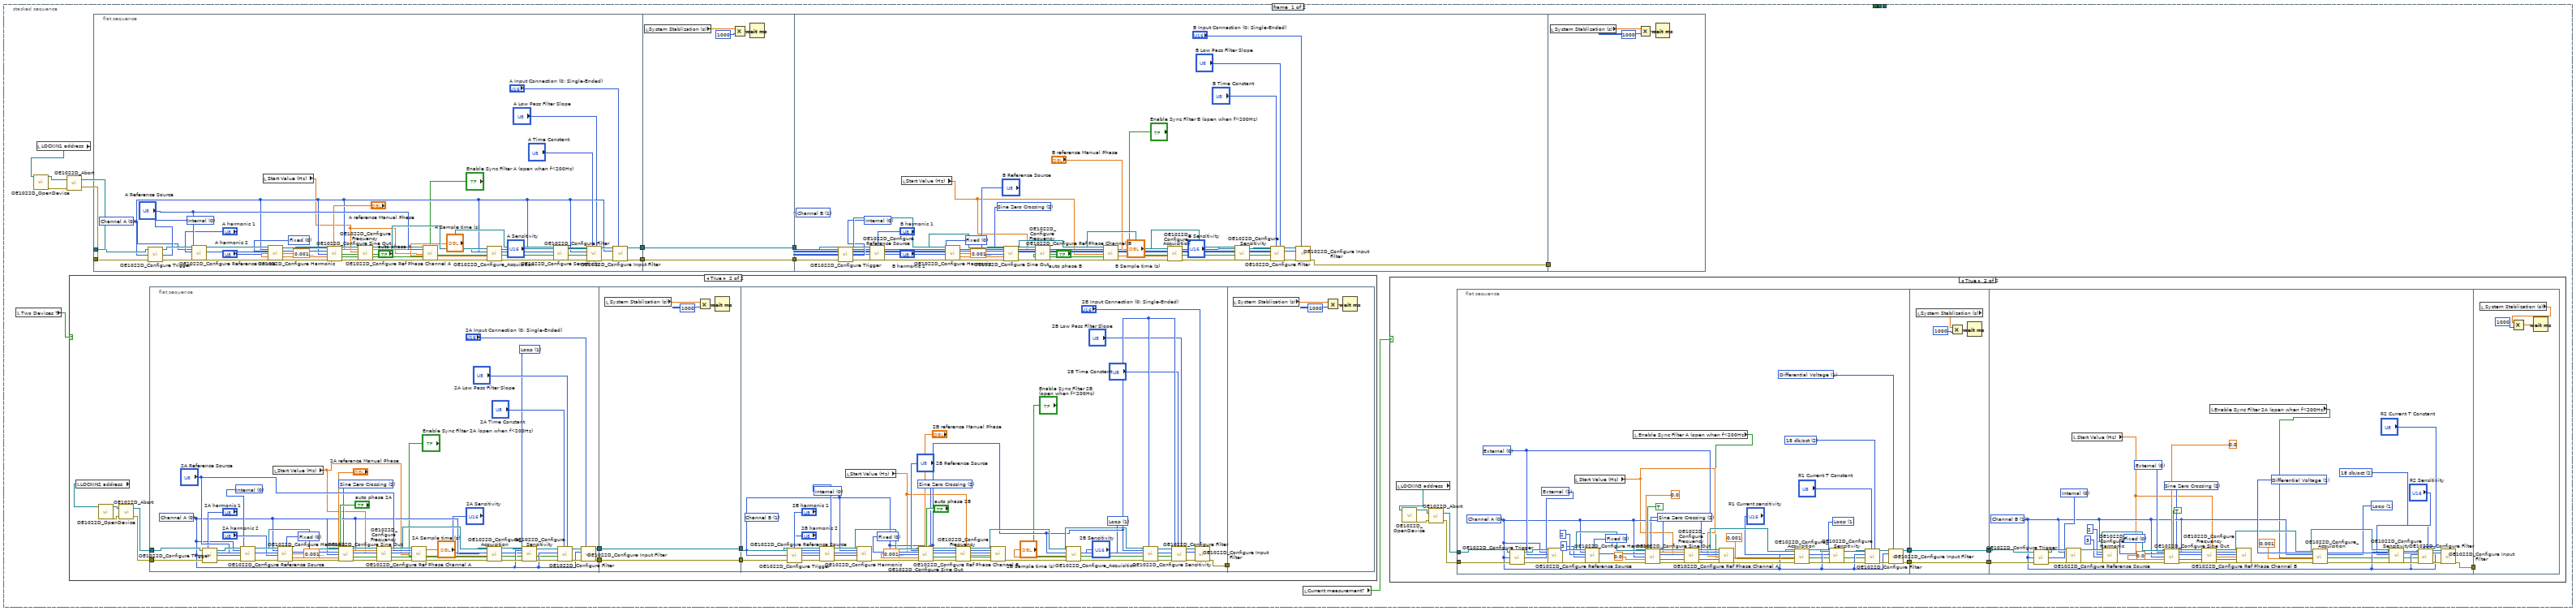
[diagram p7: hidden frame]
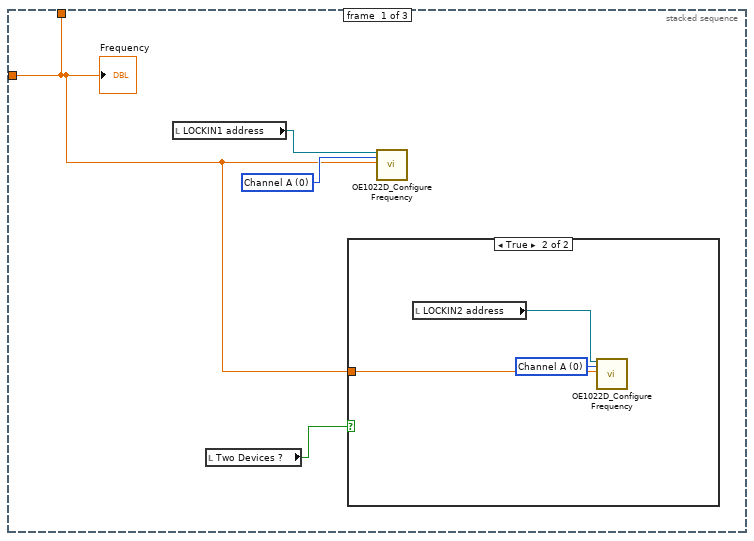
[diagram p10: hidden frame]
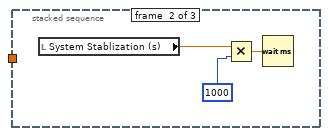
[diagram p12: hidden frame]
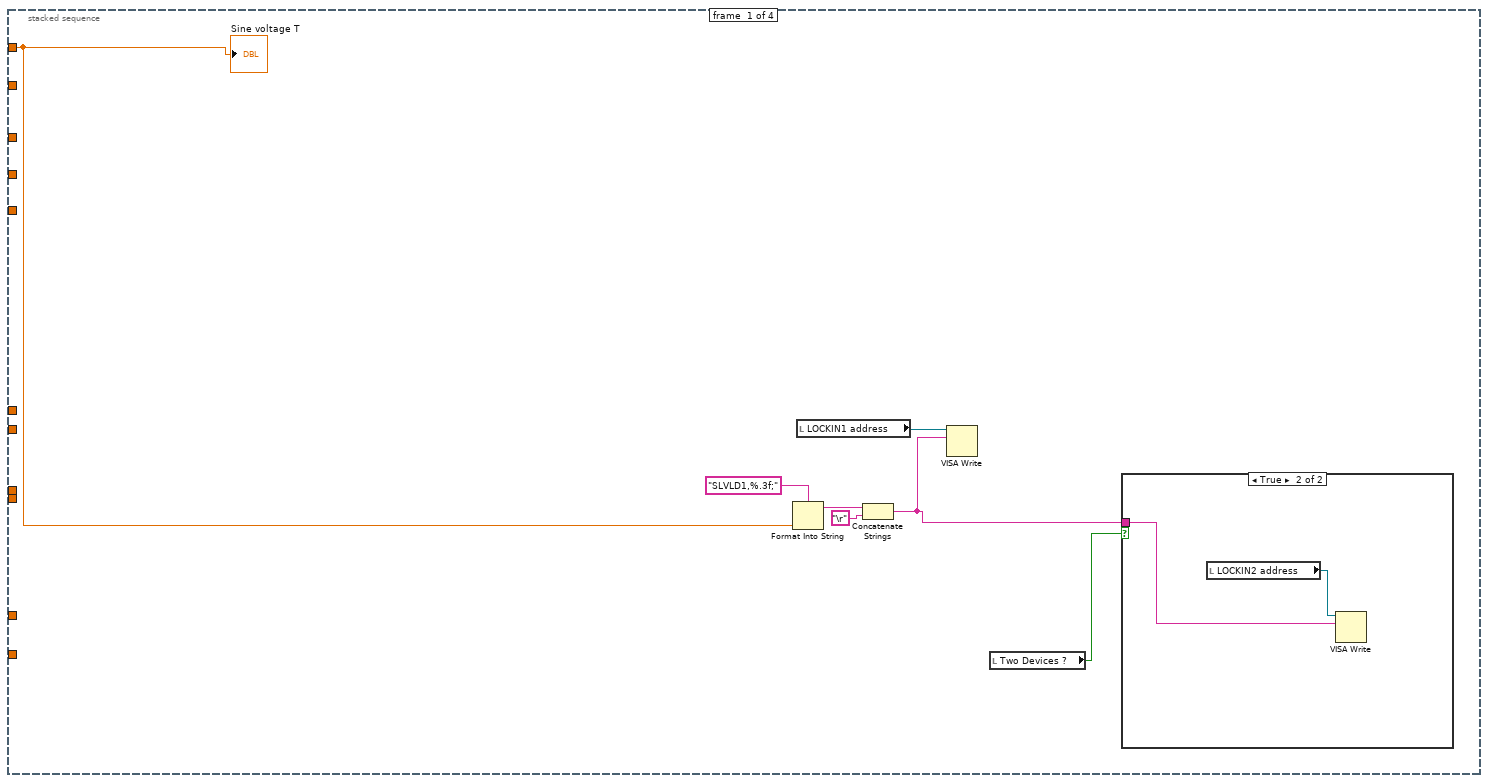
[diagram p13: hidden frame]
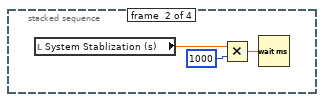
[diagram p15: hidden frame]
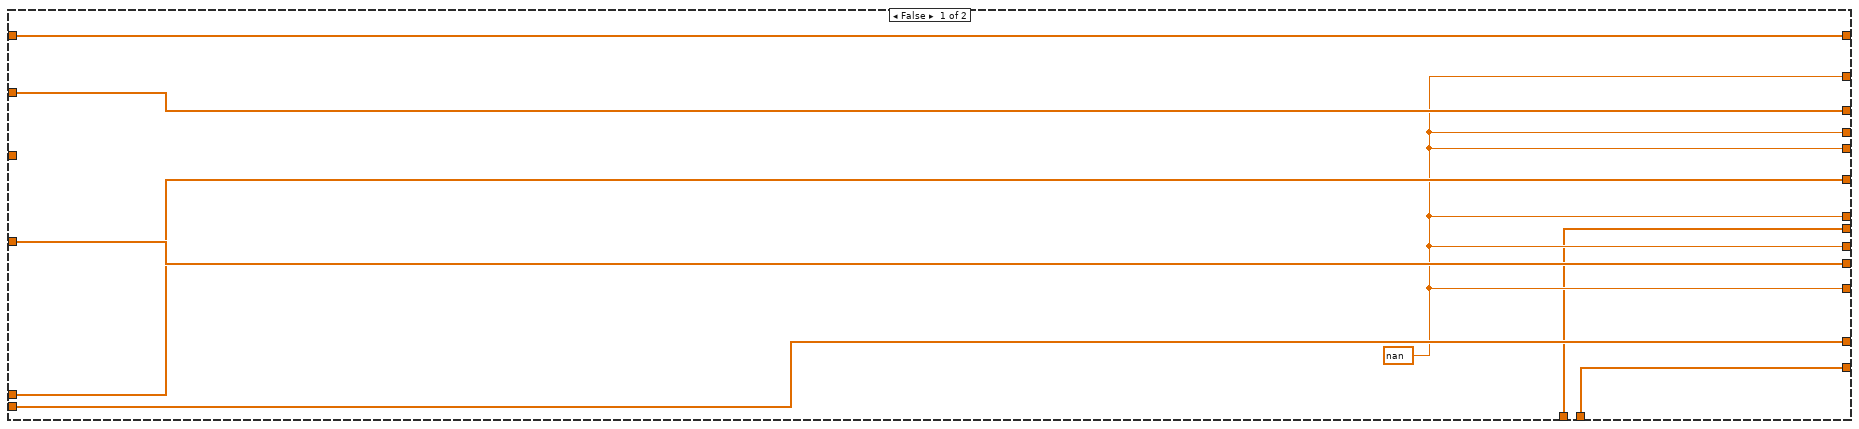
[diagram p17: hidden frame]
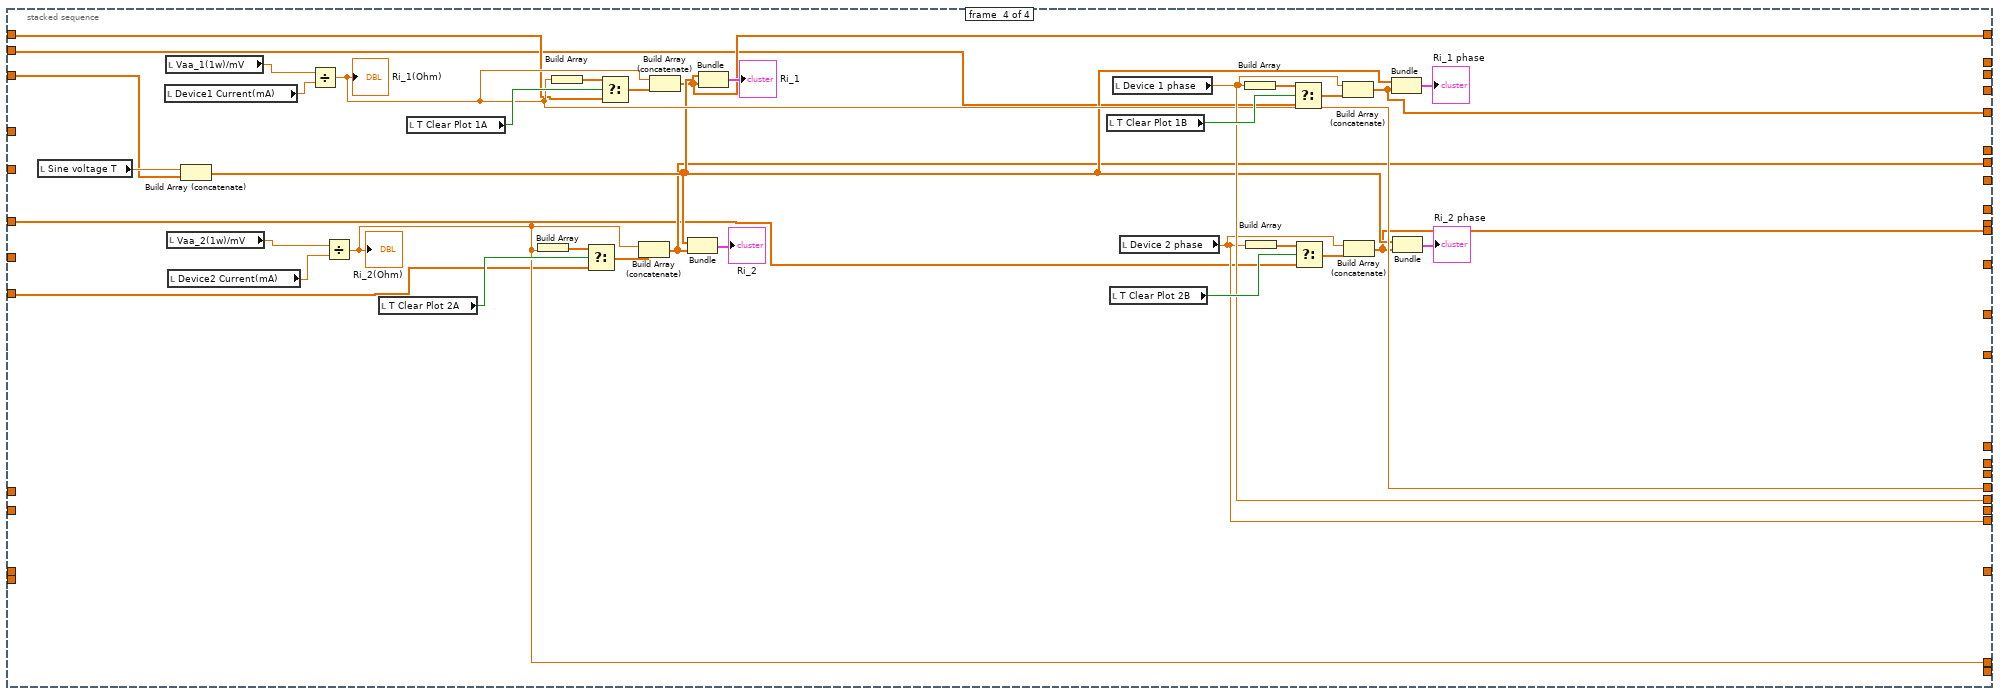
[diagram p18: hidden frame]
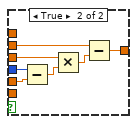
[diagram p19: hidden frame]
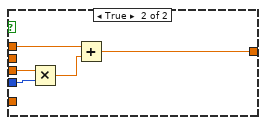
[diagram p20: hidden frame]
diagram:
  w13 = ".txt"
  n1 = flat-sequence {
    tunnel: w12 -> [w74]
    tunnel: w11 -> [w73]
    tunnel: "Save data or not" -> [w72]
    frame #0 {
      n2 = case shown="True" "Temperature \n& Field Function" {
        frame False {
        }
        frame True {
          w49 = 4 items=["PPMS", "VersaLab", "DynaCool", "SVSM", "OptiCool"] ("InstrumentType")
          n3 = call "OpenQDInstrument.vi"("Remote"="Remote", "IP Address"="IP Address 2", "InstrumentType"=w49) -> ("error out"=w40:errorcluster, "Instrument Ref"=w41:refnum<k24>)  [unwired: 5 in]
          n4 = call "SetTemperature.vi"("Approach"="Temperature Approach", "Rate"="T  Rate (K/min)", "Temperature"="Set  T  (K)", "error in (no error)"=w40, "Instrument Ref In"=w41) -> ("error out"=w54:errorcluster, "Instrument Ref Out"=w53:refnum<k24>)  [unwired: 2 in, 1 out]
          n5 = call "SetField.vi"("Mode"="Mode", "Approach"="Field Approach", "Rate"="F Rate (Oe/s)", "Field"="Set F (Oe)", "error in (no error)"=w54, "Instrument Ref In"=w53) -> ("error out"=w38:errorcluster, "Instrument Ref Out"=w39:refnum<k24>)  [unwired: 1 in, 1 out]
          n6 = call "WaitFor.vi"("Delay"="Delay", "Wait For Field"="WaitForField", "Wait For Temperature"="WaitForTemperature", "error in (no error)"=w38, "Instrument Ref In"=w39) -> ("error out"=w48:errorcluster, "Instrument Ref Out"=w44:refnum<k24>)  [unwired: 5 in]
          n7 = for {
            N: 20 -> [_]
            shift-right: [w70] -> _
            shift-left: TRUE -> [w68]
            shift-right: [w65] -> w26
            shift-left: w48 -> [w67]
            tunnel: w44 -> [w64]
            tunnel: [w62] -> w27
            tunnel: [w59] -> w29
            tunnel: [w58] -> w28
            tunnel: [w60] -> w42 mode=indexing
            tunnel: [w61] -> w43 mode=indexing
            n8 = Not(x=w68) -> (.not. x?=w70:bool)
            n9 = local write "Measuring"(w68) -> ()
            n10 = call "GetTemperature.vi"("error in (no error)"=w67, "Instrument Ref In"=w64) -> ("Temperature\nStatus"=w58:i32, "Temperature"=w61:dbl, "error out"=w66:errorcluster, "Instrument Ref Out"=w63:refnum<k24>)  [unwired: 3 in, 1 out]
            n11 = Wait (ms)(milliseconds to wait=u32 200) -> ()  [unwired: 1 out]
            n12 = call "GetField.vi"("error in (no error)"=w66, "Instrument Ref In"=w63) -> ("Field\nStatus"=w59:i32, "Field"=w60:dbl, "error out"=w65:errorcluster, "Instrument Ref Out"=w62:refnum<k24>)  [unwired: 3 in, 1 out]
          }
          "Field Status" <- w29
          "Temperature Status" <- w28
          "Instrument Ref Out" <- w27
          "error out" <- w26
          n13 = call-poly <vilib>:"Mean.vi"("X"=w42) -> ("mean"=→"Field":dbl)  [unwired: 1 out]
          n14 = call-poly <vilib>:"Mean.vi"("X"=w43) -> ("mean"=→"Temperature":dbl)  [unwired: 1 out]
          "Measuring" <- FALSE
        }
      }
    }
    frame #1 {
      n15 = case shown="True" "Two Devices ?" {
        frame False {
        }
        frame True {
        }
      }
      n16 = case shown="True" "Current measurement?" {
        frame False {
        }
        frame True {
        }
      }
      n17 = stacked-sequence {
        tunnel: w74 -> [_ w372]
        tunnel: w73 -> [_ w371]
        tunnel: w72 -> [_ w373]
        frame #0 {
          n18 = local read "Two Devices ?"() -> (w77:bool)
          n19 = local read "LOCKIN1 address"() -> (w78:refnum<visa-resource-name>)
          n20 = call "OE1022D_OpenDevice.vi"("VISA resource name"=w78) -> ("VISA资源名称输出"=w79:refnum<visa-resource-name>, "错误输出"=w80:errorcluster)  [unwired: 17 in]
          n21 = call "OE1022D_Abort.vi"("error in (no error)"=w80, "VISA resource name"=w79) -> ("error out"=w85:errorcluster, "VISA resource name out"=w86:refnum<visa-resource-name>)
          n22 = case shown="True" w77 {
            frame False {
            }
            frame True {
              n23 = local read "LOCKIN2 address"() -> (w185:refnum<visa-resource-name>)
              n24 = call "OE1022D_OpenDevice.vi"("VISA resource name"=w185) -> ("VISA资源名称输出"=w188:refnum<visa-resource-name>, "错误输出"=w189:errorcluster)  [unwired: 17 in]
              n25 = call "OE1022D_Abort.vi"("error in (no error)"=w189, "VISA resource name"=w188) -> ("error out"=w186:errorcluster, "VISA resource name out"=w187:refnum<visa-resource-name>)
              n26 = flat-sequence {
                tunnel: w187 -> [w234]
                tunnel: [w222] -> w194
                tunnel: w186 -> [w233]
                tunnel: [w211] -> w193
                tunnel: w194 -> [w239]
                tunnel: [w239] -> w192
                tunnel: w193 -> [w238]
                tunnel: [w238] -> w191
                tunnel: w192 -> [w261]
                tunnel: [w260] -> w190
                tunnel: w191 -> [w259]
                tunnel: w190 -> [_]
                frame #0 {
                  w196 = u8 2 items=["TTL Pos", "TTL Neg", "Sine Zero Crossing"] ("External Ref Trigger")
                  w197 = u8 1 items=["Single", "Loop"] ("Sample Mode (Single/Loop)")
                  w210 = u8 0 items=["Fixed", "Linear", "Log"] ("SineOut Mode")
                  w212 = u16 0 items=["Internal", "External"] ("Trigger Source (0: Internal)")
                  w201 = u8 0 items=["Channel A", "Channel B"] ("OE1022D A/B")
                  n27 = call "OE1022D_Configure Trigger.vi"("Trigger Source (0: Internal)"=w212, "error in (no error)   2"=w233, "OE1022D A/B"=w201, "VISA resource name   2"=w234) -> ("error out   2"=w227:errorcluster, "VISA resource name out   2"=w228:refnum<visa-resource-name>)
                  n28 = call "OE1022D_Configure Reference Source.vi"("VISA resource name"=w228, "OE1022D A/B"=w201, "Reference Source"="2A Reference Source", "error in (no error)"=w227) -> ("VISA resource name out"=w226:refnum<visa-resource-name>, "error out"=w224:errorcluster)  [unwired: 14 in]
                  n29 = local read "Start Value (Hz)"() -> (w195:dbl)
                  n30 = call "OE1022D_Configure Harmonic.vi"("VISA resource name"=w226, "OE1022D A/B"=w201, "Harmonic 1"="2A harmonic 1", "Harmonic 2"="2A harmonic 2", "error in (no error)"=w224) -> ("VISA resource name out"=w225:refnum<visa-resource-name>, "error out"=w223:errorcluster)  [unwired: 13 in]
                  n31 = call "OE1022D_Configure Sine Out.vi"("VISA resource name"=w225, "SineOut Mode"=w210, "OE1022D A/B"=w201, "Sine Output Amplitude (V)"=sgl 0.001, "error in (no error)"=w223) -> ("VISA resource name out"=w231:refnum<visa-resource-name>, "error out"=w230:errorcluster)  [unwired: 9 in]
                  n32 = call "OE1022D_Configure Frequency.vi"("VISA resource name"=w231, "OE1022D A/B"=w201, "Internal Frequency(Hz)"=w195, "error in (no error)"=w230) -> ("VISA resource name out"=w221:refnum<visa-resource-name>, "error out"=w218:errorcluster)  [unwired: 14 in]
                  n33 = call "OE1022D_Configure Ref Phase Channel A.vi"("VISA resource name"=w221, "Reference Source"="2A Reference Source", "External Ref Trigger"=w196, "Internal Frequency(Hz)"=w195, "Auto Phase (T: Enabled)"="auto phase 2A", "error in (no error)"=w218, "Manual Phase  (degree)"="2A reference Manual Phase") -> ("VISA resource name out"=w220:refnum<visa-resource-name>, "error out"=w219:errorcluster)  [unwired: 11 in]
                  n34 = call "OE1022D_Configure_Acquisition.vi"("VISA resource name"=w220, "OE1022D A/B"=w201, "Sample time (s)"="2A Sample time (s)", "error in (no error)"=w219, "Sample Mode (Single/Loop)"=w197) -> ("VISA resource name out"=w204:refnum<visa-resource-name>, "error out"=w203:errorcluster)  [unwired: 3 in]
                  n35 = call "OE1022D_Configure Sensitivity.vi"("VISA resource name"=w204, "OE1022D A/B"=w201, "Sensitivity"="2A Sensitivity", "error in (no error)"=w203) -> ("VISA resource name out"=w208:refnum<visa-resource-name>, "error out"=w207:errorcluster)  [unwired: 14 in]
                  n36 = call "OE1022D_Configure Filter.vi"("Low Pass Filter Slope (1: 12dB/oct)"="2A Low Pass Filter Slope", "Time Constant (8: 100ms)"="2A Time Constant", "error in (no error)"=w207, "Enable Sync Filter (F: Disable)"="Enable Sync Filter 2A (open when f<200Hz)", "OE1022D A/B"=w201, "VISA resource name"=w208) -> ("error out"=w205:errorcluster, "VISA resource name out"=w206:refnum<visa-resource-name>)  [unwired: 4 in]
                  n37 = call "OE1022D_Configure Input Filter.vi"("VISA resource name"=w206, "Input Source"="2A Input Connection (0: Single-Ended)", "OE1022D A/B"=w201, "error in (no error)"=w205) -> ("VISA resource name out"=w211:refnum<visa-resource-name>, "error out"=w222:errorcluster)  [unwired: 10 in]
                }
                frame #1 {
                  n38 = local read "System Stablization (s)"() -> (w235:dbl)
                  n39 = Multiply(x=w235, y=1000) -> (x*y=w237:dbl)
                  n40 = Wait (ms)(milliseconds to wait=w237) -> ()  [unwired: 1 out]
                }
                frame #2 {
                  w242 = u8 1 items=["Single", "Loop"] ("Sample Mode (Single/Loop)")
                  w244 = u8 2 items=["TTL Pos", "TTL Neg", "Sine Zero Crossing"] ("External Ref Trigger")
                  w256 = u8 0 items=["Fixed", "Linear", "Log"] ("SineOut Mode")
                  w262 = u16 0 items=["Internal", "External"] ("Trigger Source (0: Internal)")
                  w248 = u8 1 items=["Channel A", "Channel B"] ("OE1022D A/B")
                  n41 = call "OE1022D_Configure Trigger.vi"("Trigger Source (0: Internal)"=w262, "error in (no error)   2"=w261, "OE1022D A/B"=w248, "VISA resource name   2"=w259) -> ("error out   2"=w274:errorcluster, "VISA resource name out   2"=w275:refnum<visa-resource-name>)
                  n42 = call "OE1022D_Configure Reference Source.vi"("VISA resource name"=w275, "OE1022D A/B"=w248, "error in (no error)"=w274) -> ("VISA resource name out"=w273:refnum<visa-resource-name>, "error out"=w271:errorcluster)  [unwired: 15 in]
                  n43 = local read "Start Value (Hz)"() -> (w240:dbl)
                  n44 = call "OE1022D_Configure Harmonic.vi"("VISA resource name"=w273, "OE1022D A/B"=w248, "Harmonic 1"="2B harmonic 1", "Harmonic 2"="2B harmonic 2", "error in (no error)"=w271) -> ("VISA resource name out"=w272:refnum<visa-resource-name>, "error out"=w270:errorcluster)  [unwired: 13 in]
                  n45 = call "OE1022D_Configure Sine Out.vi"("VISA resource name"=w272, "SineOut Mode"=w256, "OE1022D A/B"=w248, "Sine Output Amplitude (V)"=sgl 0.001, "error in (no error)"=w270) -> ("VISA resource name out"=w277:refnum<visa-resource-name>, "error out"=w276:errorcluster)  [unwired: 9 in]
                  n46 = call "OE1022D_Configure Frequency.vi"("VISA resource name"=w277, "OE1022D A/B"=w248, "Internal Frequency(Hz)"=w240, "error in (no error)"=w276) -> ("VISA resource name out"=w269:refnum<visa-resource-name>, "error out"=w266:errorcluster)  [unwired: 14 in]
                  n47 = call "OE1022D_Configure Ref Phase Channel B.vi"("VISA resource name"=w269, "Reference Source"="2B Reference Source", "External Ref Trigger"=w244, "Internal Frequency(Hz)"=w240, "Auto Phase (T: Enabled)"="auto phase 2B", "error in (no error)"=w266, "Manual Phase  (degree)"="2B reference Manual Phase") -> ("VISA resource name out"=w268:refnum<visa-resource-name>, "error out"=w267:errorcluster)  [unwired: 11 in]
                  n48 = call "OE1022D_Configure_Acquisition.vi"("VISA resource name"=w268, "OE1022D A/B"=w248, "Sample time (s)"="2B Sample time (s)", "error in (no error)"=w267, "Sample Mode (Single/Loop)"=w242) -> ("VISA resource name out"=w249:refnum<visa-resource-name>, "error out"=w250:errorcluster)  [unwired: 3 in]
                  n49 = call "OE1022D_Configure Sensitivity.vi"("VISA resource name"=w249, "OE1022D A/B"=w248, "Sensitivity"="2B Sensitivity", "error in (no error)"=w250) -> ("VISA resource name out"=w253:refnum<visa-resource-name>, "error out"=w252:errorcluster)  [unwired: 14 in]
                  n50 = call "OE1022D_Configure Filter.vi"("Low Pass Filter Slope (1: 12dB/oct)"="2B Low Pass Filter Slope", "Time Constant (8: 100ms)"="2B Time Constant", "error in (no error)"=w252, "Enable Sync Filter (F: Disable)"="Enable Sync Filter 2B (open when f<200Hz)", "OE1022D A/B"=w248, "VISA resource name"=w253) -> ("error out"=w251:errorcluster, "VISA resource name out"=w241:refnum<visa-resource-name>)  [unwired: 4 in]
                  n51 = call "OE1022D_Configure Input Filter.vi"("VISA resource name"=w241, "Input Source"="2B Input Connection (0: Single-Ended)", "OE1022D A/B"=w248, "error in (no error)"=w251) -> ("error out"=w260:errorcluster)  [unwired: 10 in, 1 out]
                }
                frame #3 {
                  n52 = local read "System Stablization (s)"() -> (w279:dbl)
                  n53 = Multiply(x=w279, y=1000) -> (x*y=w281:dbl)
                  n54 = Wait (ms)(milliseconds to wait=w281) -> ()  [unwired: 1 out]
                }
              }
            }
          }
          n55 = flat-sequence {
            tunnel: w86 -> [w319]
            tunnel: [w307] -> w84
            tunnel: w85 -> [w318]
            tunnel: [w296] -> w82
            tunnel: w84 -> [w324]
            tunnel: [w324] -> w83
            tunnel: w82 -> [w323]
            tunnel: [w323] -> w81
            tunnel: w83 -> [w345]
            tunnel: [w344] -> w87
            tunnel: w81 -> [w343]
            tunnel: w87 -> [_]
            frame #0 {
              w295 = u8 0 items=["Fixed", "Linear", "Log"] ("SineOut Mode")
              w297 = u16 0 items=["Internal", "External"] ("Trigger Source (0: Internal)")
              w286 = u8 0 items=["Channel A", "Channel B"] ("OE1022D A/B")
              n56 = call "OE1022D_Configure Trigger.vi"("Trigger Source (0: Internal)"=w297, "error in (no error)   2"=w318, "OE1022D A/B"=w286, "VISA resource name   2"=w319) -> ("error out   2"=w312:errorcluster, "VISA resource name out   2"=w313:refnum<visa-resource-name>)
              n57 = call "OE1022D_Configure Reference Source.vi"("VISA resource name"=w313, "OE1022D A/B"=w286, "Reference Source"="A Reference Source", "error in (no error)"=w312) -> ("VISA resource name out"=w311:refnum<visa-resource-name>, "error out"=w309:errorcluster)  [unwired: 14 in]
              n58 = local read "Start Value (Hz)"() -> (w282:dbl)
              n59 = call "OE1022D_Configure Harmonic.vi"("VISA resource name"=w311, "OE1022D A/B"=w286, "Harmonic 1"="A harmonic 1", "Harmonic 2"="A harmonic 2", "error in (no error)"=w309) -> ("VISA resource name out"=w310:refnum<visa-resource-name>, "error out"=w308:errorcluster)  [unwired: 13 in]
              n60 = call "OE1022D_Configure Sine Out.vi"("VISA resource name"=w310, "SineOut Mode"=w295, "OE1022D A/B"=w286, "Sine Output Amplitude (V)"=sgl 0.001 ("A Sine Output Amplitude (V)"), "error in (no error)"=w308) -> ("VISA resource name out"=w316:refnum<visa-resource-name>, "error out"=w315:errorcluster)  [unwired: 9 in]
              n61 = call "OE1022D_Configure Frequency.vi"("VISA resource name"=w316, "OE1022D A/B"=w286, "Internal Frequency(Hz)"=w282, "error in (no error)"=w315) -> ("VISA resource name out"=w306:refnum<visa-resource-name>, "error out"=w303:errorcluster)  [unwired: 14 in]
              n62 = call "OE1022D_Configure Ref Phase Channel A.vi"("VISA resource name"=w306, "Reference Source"="A Reference Source", "Internal Frequency(Hz)"=w282, "Auto Phase (T: Enabled)"="auto phase A", "error in (no error)"=w303, "Manual Phase  (degree)"="A reference Manual Phase") -> ("VISA resource name out"=w305:refnum<visa-resource-name>, "error out"=w304:errorcluster)  [unwired: 12 in]
              n63 = call "OE1022D_Configure_Acquisition.vi"("VISA resource name"=w305, "OE1022D A/B"=w286, "Sample time (s)"="A Sample time (s)", "error in (no error)"=w304) -> ("VISA resource name out"=w289:refnum<visa-resource-name>, "error out"=w288:errorcluster)  [unwired: 4 in]
              n64 = call "OE1022D_Configure Sensitivity.vi"("VISA resource name"=w289, "OE1022D A/B"=w286, "Sensitivity"="A Sensitivity", "error in (no error)"=w288) -> ("VISA resource name out"=w293:refnum<visa-resource-name>, "error out"=w292:errorcluster)  [unwired: 14 in]
              n65 = call "OE1022D_Configure Filter.vi"("Low Pass Filter Slope (1: 12dB/oct)"="A Low Pass Filter Slope", "Time Constant (8: 100ms)"="A Time Constant", "error in (no error)"=w292, "Enable Sync Filter (F: Disable)"="Enable Sync Filter A (open when f<200Hz)", "OE1022D A/B"=w286, "VISA resource name"=w293) -> ("error out"=w290:errorcluster, "VISA resource name out"=w291:refnum<visa-resource-name>)  [unwired: 4 in]
              n66 = call "OE1022D_Configure Input Filter.vi"("VISA resource name"=w291, "Input Source"="A Input Connection (0: Single-Ended)", "OE1022D A/B"=w286, "error in (no error)"=w290) -> ("VISA resource name out"=w296:refnum<visa-resource-name>, "error out"=w307:errorcluster)  [unwired: 10 in]
            }
            frame #1 {
              n67 = local read "System Stablization (s)"() -> (w320:dbl)
              n68 = Multiply(x=w320, y=1000) -> (x*y=w322:dbl)
              n69 = Wait (ms)(milliseconds to wait=w322) -> ()  [unwired: 1 out]
            }
            frame #2 {
              w328 = u8 2 items=["TTL Pos", "TTL Neg", "Sine Zero Crossing"] ("External Ref Trigger")
              w340 = u8 0 items=["Fixed", "Linear", "Log"] ("SineOut Mode")
              w346 = u16 0 items=["Internal", "External"] ("Trigger Source (0: Internal)")
              w332 = u8 1 items=["Channel A", "Channel B"] ("OE1022D A/B")
              n70 = call "OE1022D_Configure Trigger.vi"("Trigger Source (0: Internal)"=w346, "error in (no error)   2"=w345, "OE1022D A/B"=w332, "VISA resource name   2"=w343) -> ("error out   2"=w358:errorcluster, "VISA resource name out   2"=w359:refnum<visa-resource-name>)
              n71 = call "OE1022D_Configure Reference Source.vi"("VISA resource name"=w359, "OE1022D A/B"=w332, "error in (no error)"=w358) -> ("VISA resource name out"=w357:refnum<visa-resource-name>, "error out"=w355:errorcluster)  [unwired: 15 in]
              n72 = local read "Start Value (Hz)"() -> (w325:dbl)
              n73 = call "OE1022D_Configure Harmonic.vi"("VISA resource name"=w357, "OE1022D A/B"=w332, "Harmonic 1"="B harmonic 1", "Harmonic 2"="B harmonic 2", "error in (no error)"=w355) -> ("VISA resource name out"=w356:refnum<visa-resource-name>, "error out"=w354:errorcluster)  [unwired: 13 in]
              n74 = call "OE1022D_Configure Sine Out.vi"("VISA resource name"=w356, "SineOut Mode"=w340, "OE1022D A/B"=w332, "Sine Output Amplitude (V)"=sgl 0.001, "error in (no error)"=w354) -> ("VISA resource name out"=w361:refnum<visa-resource-name>, "error out"=w360:errorcluster)  [unwired: 9 in]
              n75 = call "OE1022D_Configure Frequency.vi"("VISA resource name"=w361, "OE1022D A/B"=w332, "Internal Frequency(Hz)"=w325, "error in (no error)"=w360) -> ("VISA resource name out"=w353:refnum<visa-resource-name>, "error out"=w350:errorcluster)  [unwired: 14 in]
              n76 = call "OE1022D_Configure Ref Phase Channel B.vi"("VISA resource name"=w353, "Reference Source"="B Reference Source", "External Ref Trigger"=w328, "Internal Frequency(Hz)"=w325, "Auto Phase (T: Enabled)"="auto phase B", "error in (no error)"=w350, "Manual Phase  (degree)"="B reference Manual Phase") -> ("VISA resource name out"=w352:refnum<visa-resource-name>, "error out"=w351:errorcluster)  [unwired: 11 in]
              n77 = call "OE1022D_Configure_Acquisition.vi"("VISA resource name"=w352, "OE1022D A/B"=w332, "Sample time (s)"="B Sample time (s)", "error in (no error)"=w351) -> ("VISA resource name out"=w333:refnum<visa-resource-name>, "error out"=w334:errorcluster)  [unwired: 4 in]
              n78 = call "OE1022D_Configure Sensitivity.vi"("VISA resource name"=w333, "OE1022D A/B"=w332, "Sensitivity"="B Sensitivity", "error in (no error)"=w334) -> ("VISA resource name out"=w337:refnum<visa-resource-name>, "error out"=w336:errorcluster)  [unwired: 14 in]
              n79 = call "OE1022D_Configure Filter.vi"("Low Pass Filter Slope (1: 12dB/oct)"="B Low Pass Filter Slope", "Time Constant (8: 100ms)"="B Time Constant", "error in (no error)"=w336, "Enable Sync Filter (F: Disable)"="Enable Sync Filter B (open when f<200Hz)", "OE1022D A/B"=w332, "VISA resource name"=w337) -> ("error out"=w335:errorcluster, "VISA resource name out"=w326:refnum<visa-resource-name>)  [unwired: 4 in]
              n80 = call "OE1022D_Configure Input Filter.vi"("VISA resource name"=w326, "Input Source"="B Input Connection (0: Single-Ended)", "OE1022D A/B"=w332, "error in (no error)"=w335) -> ("error out"=w344:errorcluster)  [unwired: 10 in, 1 out]
            }
            frame #3 {
              n81 = local read "System Stablization (s)"() -> (w363:dbl)
              n82 = Multiply(x=w363, y=1000) -> (x*y=w365:dbl)
              n83 = Wait (ms)(milliseconds to wait=w365) -> ()  [unwired: 1 out]
            }
          }
          n84 = local read "Current measurement?"() -> (w76:bool)
          n85 = case shown="True" w76 {
            frame False {
            }
            frame True {
              n86 = local read "LOCKIN3 address"() -> (w88:refnum<visa-resource-name>)
              n87 = call "OE1022D_OpenDevice.vi"("VISA resource name"=w88) -> ("VISA资源名称输出"=w91:refnum<visa-resource-name>, "错误输出"=w92:errorcluster)  [unwired: 17 in]
              n88 = call "OE1022D_Abort.vi"("error in (no error)"=w92, "VISA resource name"=w91) -> ("error out"=w89:errorcluster, "VISA resource name out"=w90:refnum<visa-resource-name>)
              n89 = flat-sequence {
                tunnel: w90 -> [w137]
                tunnel: [w125] -> w97
                tunnel: w89 -> [w136]
                tunnel: [w114] -> w96
                tunnel: w97 -> [w142]
                tunnel: [w142] -> w95
                tunnel: w96 -> [w141]
                tunnel: [w141] -> w94
                tunnel: w95 -> [w164]
                tunnel: [w163] -> w93
                tunnel: w94 -> [w162]
                tunnel: w93 -> [_]
                frame #0 {
                  w135 = u16 1 items=["Single-Ended Voltage", "Differential Voltage", "1 MOhm Current Gain", "100 MOhm Current Gain"] ("2A Input Connection (0: Single-Ended)  2")
                  w102 = u8 2 items=["6 dB/oct", "12 dB/oct", "18 db/oct", "24 dB/oct"] ("2A Low Pass Filter Slope 2")
                  w120 = u8 0 items=["External", "Internal", "Internal Sweep"] ("2A Reference Source 2")
                  w115 = u16 1 items=["Internal", "External"] ("Trigger Source (0: Internal)")
                  w100 = u8 2 items=["TTL Pos", "TTL Neg", "Sine Zero Crossing"] ("External Ref Trigger")
                  w101 = u8 1 items=["Single", "Loop"] ("Sample Mode (Single/Loop)")
                  w113 = u8 0 items=["Fixed", "Linear", "Log"] ("SineOut Mode")
                  w104 = u8 0 items=["Channel A", "Channel B"] ("OE1022D A/B")
                  n90 = call "OE1022D_Configure Trigger.vi"("Trigger Source (0: Internal)"=w115, "error in (no error)   2"=w136, "OE1022D A/B"=w104, "VISA resource name   2"=w137) -> ("error out   2"=w130:errorcluster, "VISA resource name out   2"=w131:refnum<visa-resource-name>)
                  n91 = call "OE1022D_Configure Reference Source.vi"("VISA resource name"=w131, "OE1022D A/B"=w104, "Reference Source"=w120, "error in (no error)"=w130) -> ("VISA resource name out"=w129:refnum<visa-resource-name>, "error out"=w127:errorcluster)  [unwired: 14 in]
                  n92 = local read "Start Value (Hz)"() -> (w99:dbl)
                  n93 = call "OE1022D_Configure Harmonic.vi"("VISA resource name"=w129, "OE1022D A/B"=w104, "Harmonic 1"=u8 2 ("2A harmonic 4"), "Harmonic 2"=u8 3 ("2A harmonic 3"), "error in (no error)"=w127) -> ("VISA resource name out"=w128:refnum<visa-resource-name>, "error out"=w126:errorcluster)  [unwired: 13 in]
                  n94 = local read "Enable Sync Filter A (open when f<200Hz)"() -> (w98:bool)
                  n95 = call "OE1022D_Configure Sine Out.vi"("VISA resource name"=w128, "SineOut Mode"=w113, "OE1022D A/B"=w104, "Sine Output Amplitude (V)"=sgl 0.0, "error in (no error)"=w126) -> ("VISA resource name out"=w134:refnum<visa-resource-name>, "error out"=w133:errorcluster)  [unwired: 9 in]
                  n96 = call "OE1022D_Configure Frequency.vi"("VISA resource name"=w134, "OE1022D A/B"=w104, "Internal Frequency(Hz)"=w99, "error in (no error)"=w133) -> ("VISA resource name out"=w124:refnum<visa-resource-name>, "error out"=w121:errorcluster)  [unwired: 14 in]
                  n97 = call "OE1022D_Configure Ref Phase Channel A.vi"("VISA resource name"=w124, "Reference Source"=w120, "External Ref Trigger"=w100, "Internal Frequency(Hz)"=w99, "Auto Phase (T: Enabled)"=TRUE ("auto phase 2A 2"), "error in (no error)"=w121, "Manual Phase  (degree)"=0.0 ("2A reference Manual Phase 2")) -> ("VISA resource name out"=w123:refnum<visa-resource-name>, "error out"=w122:errorcluster)  [unwired: 11 in]
                  n98 = call "OE1022D_Configure_Acquisition.vi"("VISA resource name"=w123, "OE1022D A/B"=w104, "Sample time (s)"=0.001 ("2A Sample time (s) 2"), "error in (no error)"=w122, "Sample Mode (Single/Loop)"=w101) -> ("VISA resource name out"=w107:refnum<visa-resource-name>, "error out"=w106:errorcluster)  [unwired: 3 in]
                  n99 = call "OE1022D_Configure Sensitivity.vi"("VISA resource name"=w107, "OE1022D A/B"=w104, "Sensitivity"="R1 Current sensitivity", "error in (no error)"=w106) -> ("VISA resource name out"=w111:refnum<visa-resource-name>, "error out"=w110:errorcluster)  [unwired: 14 in]
                  n100 = call "OE1022D_Configure Filter.vi"("Low Pass Filter Slope (1: 12dB/oct)"=w102, "Time Constant (8: 100ms)"="R1 Current T Constant", "error in (no error)"=w110, "Enable Sync Filter (F: Disable)"=w98, "OE1022D A/B"=w104, "VISA resource name"=w111) -> ("error out"=w108:errorcluster, "VISA resource name out"=w109:refnum<visa-resource-name>)  [unwired: 4 in]
                  n101 = call "OE1022D_Configure Input Filter.vi"("VISA resource name"=w109, "Input Source"=w135, "OE1022D A/B"=w104, "error in (no error)"=w108) -> ("VISA resource name out"=w114:refnum<visa-resource-name>, "error out"=w125:errorcluster)  [unwired: 10 in]
                }
                frame #1 {
                  n102 = local read "System Stablization (s)"() -> (w138:dbl)
                  n103 = Multiply(x=w138, y=1000) -> (x*y=w140:dbl)
                  n104 = Wait (ms)(milliseconds to wait=w140) -> ()  [unwired: 1 out]
                }
                frame #2 {
                  w147 = u8 2 items=["6 dB/oct", "12 dB/oct", "18 db/oct", "24 dB/oct"] ("2B Low Pass Filter Slope 2")
                  w181 = u16 1 items=["Single-Ended Voltage", "Differential Voltage", "1 MOhm Current Gain", "100 MOhm Current Gain"] ("2B Input Connection (0: Single-Ended) 2")
                  w168 = u8 0 items=["External", "Internal", "Internal Sweep", "Channel-A"] ("2B Reference Source 2")
                  w146 = u8 1 items=["Single", "Loop"] ("Sample Mode (Single/Loop)")
                  w148 = u8 2 items=["TTL Pos", "TTL Neg", "Sine Zero Crossing"] ("External Ref Trigger")
                  w159 = u8 0 items=["Fixed", "Linear", "Log"] ("SineOut Mode")
                  w165 = u16 0 items=["Internal", "External"] ("Trigger Source (0: Internal)")
                  w151 = u8 1 items=["Channel A", "Channel B"] ("OE1022D A/B")
                  n105 = call "OE1022D_Configure Trigger.vi"("Trigger Source (0: Internal)"=w165, "error in (no error)   2"=w164, "OE1022D A/B"=w151, "VISA resource name   2"=w162) -> ("error out   2"=w177:errorcluster, "VISA resource name out   2"=w178:refnum<visa-resource-name>)
                  n106 = call "OE1022D_Configure Reference Source.vi"("VISA resource name"=w178, "OE1022D A/B"=w151, "error in (no error)"=w177) -> ("VISA resource name out"=w176:refnum<visa-resource-name>, "error out"=w174:errorcluster)  [unwired: 15 in]
                  n107 = local read "Start Value (Hz)"() -> (w144:dbl)
                  n108 = call "OE1022D_Configure Harmonic.vi"("VISA resource name"=w176, "OE1022D A/B"=w151, "Harmonic 1"=u8 2 ("2B harmonic 4"), "Harmonic 2"=u8 3 ("2B harmonic 3"), "error in (no error)"=w174) -> ("VISA resource name out"=w175:refnum<visa-resource-name>, "error out"=w173:errorcluster)  [unwired: 13 in]
                  n109 = call "OE1022D_Configure Sine Out.vi"("VISA resource name"=w175, "SineOut Mode"=w159, "OE1022D A/B"=w151, "Sine Output Amplitude (V)"=sgl 0.0, "error in (no error)"=w173) -> ("VISA resource name out"=w180:refnum<visa-resource-name>, "error out"=w179:errorcluster)  [unwired: 9 in]
                  n110 = call "OE1022D_Configure Frequency.vi"("VISA resource name"=w180, "OE1022D A/B"=w151, "Internal Frequency(Hz)"=w144, "error in (no error)"=w179) -> ("VISA resource name out"=w172:refnum<visa-resource-name>, "error out"=w169:errorcluster)  [unwired: 14 in]
                  n111 = local read "Enable Sync Filter 2A (open when f<200Hz)"() -> (w143:bool)
                  n112 = call "OE1022D_Configure Ref Phase Channel B.vi"("VISA resource name"=w172, "Reference Source"=w168, "External Ref Trigger"=w148, "Internal Frequency(Hz)"=w144, "Auto Phase (T: Enabled)"=TRUE ("auto phase 2B 2"), "error in (no error)"=w169, "Manual Phase  (degree)"=0.0 ("2B reference Manual Phase 2")) -> ("VISA resource name out"=w171:refnum<visa-resource-name>, "error out"=w170:errorcluster)  [unwired: 11 in]
                  n113 = call "OE1022D_Configure_Acquisition.vi"("VISA resource name"=w171, "OE1022D A/B"=w151, "Sample time (s)"=0.001 ("2B Sample time (s) 2"), "error in (no error)"=w170, "Sample Mode (Single/Loop)"=w146) -> ("VISA resource name out"=w152:refnum<visa-resource-name>, "error out"=w153:errorcluster)  [unwired: 3 in]
                  n114 = call "OE1022D_Configure Sensitivity.vi"("VISA resource name"=w152, "OE1022D A/B"=w151, "Sensitivity"="R2 Sensitivity", "error in (no error)"=w153) -> ("VISA resource name out"=w156:refnum<visa-resource-name>, "error out"=w155:errorcluster)  [unwired: 14 in]
                  n115 = call "OE1022D_Configure Filter.vi"("Low Pass Filter Slope (1: 12dB/oct)"=w147, "Time Constant (8: 100ms)"="R2 Current T Constant", "error in (no error)"=w155, "Enable Sync Filter (F: Disable)"=w143, "OE1022D A/B"=w151, "VISA resource name"=w156) -> ("error out"=w154:errorcluster, "VISA resource name out"=w145:refnum<visa-resource-name>)  [unwired: 4 in]
                  n116 = call "OE1022D_Configure Input Filter.vi"("VISA resource name"=w145, "Input Source"=w181, "OE1022D A/B"=w151, "error in (no error)"=w154) -> ("error out"=w163:errorcluster)  [unwired: 10 in, 1 out]
                }
                frame #3 {
                  n117 = local read "System Stablization (s)"() -> (w182:dbl)
                  n118 = Multiply(x=w182, y=1000) -> (x*y=w184:dbl)
                  n119 = Wait (ms)(milliseconds to wait=w184) -> ()  [unwired: 1 out]
                }
              }
            }
          }
        }
        frame #1 {
          n120 = local read "Start Value (Hz)"() -> (w367:dbl)
          n121 = Logarithm Base 10(1:w367) -> (0:w370:dbl)
          n122 = Round Toward -Infinity(1:w370) -> (0:w369:dbl)
          n123 = Power Of 10(x=w369) -> (10^x=w368:dbl)
          n124 = Subtract(x=w367, y=w368) -> (x-y=w366:dbl)
          n125 = while {
            tunnel: w373 -> [w393]
            tunnel: w372 -> [w392]
            tunnel: w371 -> [w391]
            shift-right: [w387] -> _
            shift-left: w366 -> [w386]
            stop <- w385 stop-if-true
            n126 = Logarithm Base 10(1:w386) -> (0:w390:dbl)
            n127 = Round Toward -Infinity(1:w390) -> (0:w389:dbl)
            n128 = Power Of 10(x=w389) -> (10^x=w383:dbl)
            n129 = Multiply(x="Log Step", y=w383) -> (x*y=w381:dbl)
            n130 = Add(x=w386, y=w381) -> (x+y=w388:dbl)
            n131 = Absolute Value(x=w388) -> (abs(x)=w394:dbl)
            n132 = stacked-sequence {
              tunnel: w394 -> [w396 _ _]
              tunnel: w393 -> [_ _ w407]
              tunnel: w392 -> [_ _ w406]
              tunnel: w391 -> [_ _ w405]
              tunnel: [w396 _ _] -> w387
              frame #0 {
                w398 = u8 0 items=["Channel A", "Channel B"] ("OE1022D A/B")
                n133 = local read "LOCKIN1 address"() -> (w397:refnum<visa-resource-name>)
                n134 = local read "Two Devices ?"() -> (w395:bool)
                n135 = case shown="True" w395 {
                  tunnel: w396 -> [_ w399]
                  frame False {
                  }
                  frame True {
                    w401 = u8 0 items=["Channel A", "Channel B"] ("OE1022D A/B")
                    n136 = local read "LOCKIN2 address"() -> (w400:refnum<visa-resource-name>)
                    n137 = call "OE1022D_Configure Frequency.vi"("VISA resource name"=w400, "OE1022D A/B"=w401, "Internal Frequency(Hz)"=w399) -> ()  [unwired: 15 in, 2 out]
                  }
                }
                n138 = call "OE1022D_Configure Frequency.vi"("VISA resource name"=w397, "OE1022D A/B"=w398, "Internal Frequency(Hz)"=w396) -> ()  [unwired: 15 in, 2 out]
                "Frequency" <- w396
              }
              frame #1 {
                n139 = local read "System Stablization (s)"() -> (w402:dbl)
                n140 = Multiply(x=w402, y=1000) -> (x*y=w404:dbl)
                n141 = Wait (ms)(milliseconds to wait=w404) -> ()  [unwired: 1 out]
              }
              frame #2 {
                n142 = local read "V Loop#"() -> (w408:i32)
                n143 = for {
                  N: w408 -> [_]
                  shift-right: [w442] -> _
                  shift-left: _ -> [w441]
                  shift-right: [w443] -> _
                  shift-left: _ -> [w440]
                  shift-right: [w439] -> _
                  shift-left: _ -> [w437]
                  shift-right: [w438] -> _
                  shift-left: _ -> [w436]
                  shift-right: [w435] -> _
                  shift-left: _ -> [w431]
                  shift-right: [w434] -> _
                  shift-left: _ -> [w430]
                  shift-right: [w433] -> _
                  shift-left: _ -> [w429]
                  shift-right: [w432] -> _
                  shift-left: _ -> [w428]
                  tunnel: w407 -> [w427]
                  tunnel: w406 -> [w426]
                  tunnel: w405 -> [w425]
                  shift-right: [w423] -> _
                  shift-left: _ -> [w421]
                  shift-right: [w424] -> _
                  shift-left: _ -> [w422]
                  shift-right: [w419] -> _
                  shift-left: _ -> [w417]
                  shift-right: [w420] -> _
                  shift-left: _ -> [w418]
                  shift-right: [w416] -> _
                  shift-left: _ -> [w415]
                  shift-right: [w414] -> _
                  shift-left: _ -> [w413]
                  shift-right: [w412] -> _
                  shift-left: _ -> [w411]
                  shift-right: [w410] -> _
                  shift-left: _ -> [w409]
                  i -> [w456]
                  n144 = local read "V Step(mV)"() -> (w444:i32)
                  n145 = Add(x=1, y=w456) -> (x+y=→"V Loop Run T":i32)
                  n146 = local read "High Value (V)"() -> (w446:dbl)
                  n147 = local read "Low Value (V)"() -> (w445:dbl)
                  n148 = Subtract(x=w446, y=w445) -> (x-y=w451:dbl)
                  n149 = Divide(x=w444, y=1000) -> (x/y=w448:dbl)
                  n150 = Divide(x=w451, y=w448) -> (x/y=w447:dbl)
                  n151 = Multiply(x=2, y=w447) -> (x*y=w450:dbl)
                  n152 = Increment(x=w450) -> (x+1=w449:dbl)
                  n153 = for {
                    N: w449 -> [_]
                    tunnel: w448 -> [w516]
                    tunnel: w447 -> [w518]
                    shift-right: [w505] -> _
                    shift-left: _ -> [w502]
                    shift-right: [w503] -> w442
                    shift-left: w441 -> [w501]
                    shift-right: [w504] -> w443
                    shift-left: w440 -> [w500]
                    shift-right: [w499] -> w439
                    shift-left: w437 -> [w497]
                    shift-right: [w498] -> w438
                    shift-left: w436 -> [w496]
                    shift-right: [w495] -> _
                    shift-left: _ -> [w494]
                    shift-right: [w493] -> w435
                    shift-left: w431 -> [w489]
                    shift-right: [w492] -> w434
                    shift-left: w430 -> [w486]
                    shift-right: [w491] -> w433
                    shift-left: w429 -> [w488]
                    shift-right: [w490] -> w432
                    shift-left: w428 -> [w487]
                    tunnel: w427 -> [w485]
                    tunnel: w426 -> [w484]
                    tunnel: w425 -> [w483]
                    shift-right: [w479] -> w423
                    shift-left: w421 -> [w478]
                    shift-right: [w480] -> w424
                    shift-left: w422 -> [w477]
                    shift-right: [w471] -> w419
                    shift-left: w417 -> [w470]
                    shift-right: [w472] -> w420
                    shift-left: w418 -> [w469]
                    shift-right: [w464] -> w416
                    shift-left: w415 -> [w463]
                    shift-right: [w462] -> w414
                    shift-left: w413 -> [w461]
                    shift-right: [w460] -> w412
                    shift-left: w411 -> [w459]
                    shift-right: [w458] -> w410
                    shift-left: w409 -> [w457]
                    i -> [w517]
                    n154 = local read "High Value (V)"() -> (w520:dbl)
                    n155 = local read "Low Value (V)"() -> (w521:dbl)
                    n156 = Less Or Equal?(x=w517, y=w518) -> (x <= y?=w519:bool)
                    n157 = case shown="False" w519 {
                      tunnel: w521 -> [w1087 w1115]
                      tunnel: w517 -> [w1096 w1114]
                      tunnel: w516 -> [w1095 w1113]
                      tunnel: [w1093 w1111] -> w515
                      tunnel: w520 -> [w1094 _]
                      tunnel: w518 -> [w1089 _]
                      tunnel: w517 -> [w1092 _]
                      frame False {
                        n158 = Multiply(x=w1089, y=2) -> (x*y=w1088:dbl)
                        n159 = Less Or Equal?(x=w1092, y=w1088) -> (x <= y?=w1090:bool)
                        n160 = case shown="False" w1090 {
                          tunnel: w1096 -> [w1103 w1110]
                          tunnel: w1095 -> [w1101 w1108]
                          tunnel: w1094 -> [_ w1106]
                          tunnel: [w1099 w1105] -> w1093
                          tunnel: w1089 -> [_ w1104]
                          tunnel: w1088 -> [w1098 _]
                          tunnel: w1087 -> [w1097 _]
                          frame False {
                            n161 = Subtract(x=w1103, y=w1098) -> (x-y=w1102:dbl)
                            n162 = Multiply(x=w1101, y=w1102) -> (x*y=w1100:dbl)
                            n163 = Add(x=w1097, y=w1100) -> (x+y=w1099:dbl)
                          }
                          frame True {
                            n164 = Subtract(x=w1110, y=w1104) -> (x-y=w1109:dbl)
                            n165 = Multiply(x=w1108, y=w1109) -> (x*y=w1107:dbl)
                            n166 = Subtract(x=w1106, y=w1107) -> (x-y=w1105:dbl)
                          }
                        }
                      }
                      frame True {
                        n167 = Multiply(x=w1113, y=w1114) -> (x*y=w1112:dbl)
                        n168 = Add(x=w1115, y=w1112) -> (x+y=w1111:dbl)
                      }
                    }
                    n169 = Absolute Value(x=w515) -> (abs(x)=w514:dbl)
                    n170 = stacked-sequence {
                      tunnel: w514 -> [w525 _ _ _]
                      tunnel: [_ _ w596 _] -> w513
                      tunnel: [_ _ w595 _] -> w512
                      tunnel: [_ _ w594 _] -> w511
                      tunnel: [_ _ w593 _] -> w510
                      tunnel: [_ _ w592 _] -> w509
                      tunnel: [_ _ w591 _] -> w508
                      tunnel: [_ _ w590 _] -> w507
                      tunnel: [_ _ w589 _] -> w506
                      tunnel: [_ _ w587 _] -> w505
                      tunnel: [_ _ w586 _] -> w504
                      tunnel: [_ _ w585 _] -> w503
                      tunnel: w502 -> [_ _ w584 w1063]
                      tunnel: w501 -> [_ _ w583 _]
                      tunnel: w500 -> [_ _ w582 _]
                      tunnel: [_ _ w581 _] -> w499
                      tunnel: [_ _ w580 _] -> w498
                      tunnel: w497 -> [_ _ w579 _]
                      tunnel: w496 -> [_ _ w578 _]
                      tunnel: [_ _ w577 _] -> w495
                      tunnel: w494 -> [_ _ w576 _]
                      tunnel: [_ _ w575 _] -> w493
                      tunnel: [_ _ w574 _] -> w492
                      tunnel: [_ _ w573 _] -> w491
                      tunnel: [_ _ w572 _] -> w490
                      tunnel: w489 -> [_ _ w571 _]
                      tunnel: w488 -> [_ _ w570 _]
                      tunnel: w487 -> [_ _ w569 _]
                      tunnel: w486 -> [_ _ w568 _]
                      tunnel: [_ _ w555 _] -> w482
                      tunnel: [_ _ w554 _] -> w481
                      tunnel: [_ _ w553 _] -> w480
                      tunnel: [_ _ w552 _] -> w479
                      tunnel: w478 -> [_ _ w550 _]
                      tunnel: w477 -> [_ _ w551 _]
                      tunnel: [_ _ w549 _] -> w476
                      tunnel: [_ _ w548 _] -> w475
                      tunnel: [_ _ w545 _] -> w474
                      tunnel: [_ _ w544 _] -> w473
                      tunnel: [_ _ w539 _] -> w472
                      tunnel: [_ _ w538 _] -> w471
                      tunnel: w470 -> [_ _ w536 _]
                      tunnel: w469 -> [_ _ w537 _]
                      tunnel: [_ _ _ w1062] -> w468
                      tunnel: [_ _ _ w1065] -> w467
                      tunnel: [_ _ _ w1064] -> w466
                      tunnel: [_ _ _ w1061] -> w465
                      tunnel: [_ _ _ w1059] -> w464
                      tunnel: w463 -> [_ _ _ w1058]
                      tunnel: [_ _ _ w1057] -> w462
                      tunnel: w461 -> [_ _ _ w1056]
                      tunnel: [_ _ _ w1055] -> w460
                      tunnel: w459 -> [_ _ _ w1054]
                      tunnel: [_ _ _ w1053] -> w458
                      tunnel: w457 -> [_ _ _ w1052]
                      frame #0 {
                        n171 = Format Into String(format string="SLVLD1,%.3f;", w525) -> (resulting string=w526:string)  [unwired: 2 in, 1 out]
                        n172 = local read "LOCKIN1 address"() -> (w524:refnum<visa-resource-name>)
                        n173 = Concatenate Strings(w526, "\r") -> (w522:string)
                        n174 = VISA Write(VISA resource name=w524, write buffer=w522) -> ()  [unwired: 1 in, 3 out]
                        n175 = local read "Two Devices ?"() -> (w523:bool)
                        n176 = case shown="True" w523 {
                          tunnel: w522 -> [_ w530]
                          frame False {
                          }
                          frame True {
                            n177 = local read "LOCKIN2 address"() -> (w529:refnum<visa-resource-name>)
                            n178 = VISA Write(VISA resource name=w529, write buffer=w530) -> ()  [unwired: 1 in, 3 out]
                          }
                        }
                        "Sine voltage T" <- w525
                      }
                      frame #1 {
                        n179 = local read "System Stablization (s)"() -> (w531:dbl)
                        n180 = Multiply(x=w531, y=1000) -> (x*y=w533:dbl)
                        n181 = Wait (ms)(milliseconds to wait=w533) -> ()  [unwired: 1 out]
                      }
                      frame #2 {
                        n182 = local read "Sine voltage T"() -> (w588:dbl)
                        n183 = local read "Two Devices ?"() -> (w597:bool)
                        n184 = local read "Current measurement?"() -> (w535:bool)
                        n185 = local read "LOCKIN1 address"() -> (w567:refnum<visa-resource-name>)
                        n186 = local read "LOCKIN3 address"() -> (w534:refnum<visa-resource-name>)
                        n187 = case shown="True" w597 {
                          tunnel: w588 -> [_ w736]
                          tunnel: [w693 w735] -> w596
                          tunnel: [w693 w734] -> w595
                          tunnel: [w693 w733] -> w594
                          tunnel: [w693 w732] -> w593
                          tunnel: [w696 w731] -> w572
                          tunnel: [w698 w730] -> w577
                          tunnel: w576 -> [w698 w729]
                          tunnel: w569 -> [w696 w726]
                          tunnel: [w697 w728] -> w575
                          tunnel: w571 -> [w697 w727]
                          tunnel: [w695 w725] -> w573
                          tunnel: w570 -> [w695 w724]
                          tunnel: [w694 w723] -> w574
                          tunnel: w568 -> [w694 w722]
                          tunnel: [w693 w708] -> w555
                          tunnel: [w693 w707] -> w554
                          tunnel: [w692 w704] -> w553
                          tunnel: [w691 w703] -> w552
                          tunnel: w551 -> [w692 w702]
                          tunnel: w550 -> [w691 w699]
                          frame False {
                            w693 = nan
                          }
                          frame True {
                            n188 = flat-sequence {
                              tunnel: w736 -> [w813]
                              tunnel: w729 -> [w786]
                              tunnel: [w811] -> w785
                              tunnel: [w804] -> w784
                              tunnel: [w805] -> w783
                              tunnel: [w802] -> w782
                              tunnel: [w805] -> w781
                              tunnel: [w805] -> w780
                              tunnel: [w805] -> w779
                              tunnel: [w805] -> w778
                              tunnel: [w804] -> w777
                              tunnel: [w803] -> w776
                              tunnel: [w802] -> w775
                              tunnel: [w801] -> w774
                              tunnel: ["T Clear Plot 2B"] -> w773
                              tunnel: ["T Clear Plot 2A"] -> w772
                              tunnel: [w792] -> w771
                              tunnel: [w794] -> w770
                              tunnel: [w793] -> w769
                              tunnel: [w798] -> w768
                              tunnel: [w797] -> w767
                              tunnel: w727 -> [w788]
                              tunnel: w724 -> [w787]
                              tunnel: w785 -> [w835]
                              tunnel: [w835] -> w766
                              tunnel: w784 -> [w834]
                              tunnel: [w834] -> w765
                              tunnel: w783 -> [w833]
                              tunnel: [w833] -> w764
                              tunnel: w782 -> [w832]
                              tunnel: [w832] -> w763
                              tunnel: w781 -> [w831]
                              tunnel: [w831] -> w762
                              tunnel: w780 -> [w830]
                              tunnel: [w830] -> w761
                              tunnel: w779 -> [w829]
                              tunnel: [w829] -> w760
                              tunnel: w778 -> [w828]
                              tunnel: [w828] -> w759
                              tunnel: w777 -> [w827]
                              tunnel: [w827] -> w758
                              tunnel: w776 -> [w826]
                              tunnel: [w826] -> w757
                              tunnel: w775 -> [w825]
                              tunnel: [w825] -> w756
                              tunnel: w774 -> [w824]
                              tunnel: [w824] -> w755
                              tunnel: w773 -> [w823]
                              tunnel: [w823] -> w754
                              tunnel: w772 -> [w822]
                              tunnel: [w822] -> w753
                              tunnel: w771 -> [w821]
                              tunnel: [w821] -> w752
                              tunnel: w770 -> [w820]
                              tunnel: [w820] -> w751
                              tunnel: w769 -> [w819]
                              tunnel: [w819] -> w750
                              tunnel: w768 -> [w818]
                              tunnel: [w818] -> w749
                              tunnel: w767 -> [w817]
                              tunnel: [w817] -> w748
                              tunnel: w766 -> [w843]
                              tunnel: w765 -> [w873]
                              tunnel: w764 -> [w872]
                              tunnel: w763 -> [w871]
                              tunnel: w762 -> [w837]
                              tunnel: w761 -> [w869]
                              tunnel: w760 -> [w867]
                              tunnel: w759 -> [w865]
                              tunnel: w758 -> [w862]
                              tunnel: w757 -> [w861]
                              tunnel: w756 -> [w858]
                              tunnel: w755 -> [w857]
                              tunnel: w754 -> [w836]
                              tunnel: w722 -> [w854]
                              tunnel: w753 -> [w853]
                              tunnel: w752 -> [w849]
                              tunnel: w751 -> [w838]
                              tunnel: w750 -> [w848]
                              tunnel: w749 -> [w845]
                              tunnel: w748 -> [w844]
                              tunnel: [w843] -> w747
                              tunnel: [w860] -> w746
                              tunnel: [w873] -> w745
                              tunnel: [w872] -> w744
                              tunnel: [w841] -> w743
                              tunnel: [w842] -> w742
                              tunnel: [w863] -> w741
                              tunnel: [w859] -> w740
                              tunnel: [w856] -> w739
                              tunnel: [w871] -> w738
                              tunnel: [w847] -> w737
                              tunnel: w726 -> [w839]
                              tunnel: [w838] -> w710
                              tunnel: [w837] -> w705
                              tunnel: [w836] -> w700
                              tunnel: w747 -> [w888]
                              tunnel: w746 -> [w887]
                              tunnel: w745 -> [w877]
                              tunnel: w744 -> [w886]
                              tunnel: w743 -> [w885]
                              tunnel: w742 -> [w884]
                              tunnel: w741 -> [w883]
                              tunnel: w740 -> [w882]
                              tunnel: w739 -> [w881]
                              tunnel: w738 -> [w880]
                              tunnel: w737 -> [w879]
                              tunnel: [w888] -> w721
                              tunnel: [w887] -> w720
                              tunnel: [w886] -> w719
                              tunnel: [w885] -> w718
                              tunnel: [w884] -> w717
                              tunnel: [w883] -> w716
                              tunnel: [w882] -> w715
                              tunnel: [w881] -> w714
                              tunnel: [w880] -> w713
                              tunnel: [w879] -> w712
                              tunnel: [w877] -> w711
                              tunnel: w710 -> [w876]
                              tunnel: [w876] -> w709
                              tunnel: [w875] -> w706
                              tunnel: w705 -> [w875]
                              tunnel: [w874] -> w701
                              tunnel: w700 -> [w874]
                              tunnel: [w910] -> w735
                              tunnel: [w911] -> w732
                              tunnel: [w912] -> w734
                              tunnel: [w913] -> w725
                              tunnel: [w914] -> w731
                              tunnel: [w915] -> w723
                              tunnel: [w916] -> w733
                              tunnel: [w917] -> w730
                              tunnel: [w918] -> w728
                              tunnel: w721 -> [w909]
                              tunnel: w720 -> [w918]
                              tunnel: w719 -> [w917]
                              tunnel: w718 -> [w916]
                              tunnel: w717 -> [w894]
                              tunnel: w716 -> [w915]
                              tunnel: w715 -> [w914]
                              tunnel: w714 -> [w913]
                              tunnel: w713 -> [w912]
                              tunnel: w712 -> [w911]
                              tunnel: w711 -> [w910]
                              tunnel: w709 -> [w908]
                              tunnel: [w901] -> w708
                              tunnel: [w891] -> w707
                              tunnel: w706 -> [w900]
                              tunnel: [w899] -> w704
                              tunnel: [w898] -> w703
                              tunnel: w702 -> [w897]
                              tunnel: w701 -> [w896]
                              tunnel: w699 -> [w895]
                              frame #0 {
                                w794 = u8 1 items=["Channel A", "Channel B"] ("Channel A/B for Parameter1")
                                w797 = u8 0 items=["Channel A", "Channel B"] ("Channel A/B for Parameter1")
                                n189 = local read "LOCKIN2 address"() -> (w789:refnum<visa-resource-name>)
                                n190 = Format Into String(0) -> (error out=w812:errorcluster)  [unwired: 3 in, 1 out]
                                n191 = Format Into String(0) -> (error out=w795:errorcluster)  [unwired: 3 in, 1 out]
                                n192 = call "OE1022D_Read 1 parameter_mean.vi"("错误输入（无错误）"=w812, "Parameter"="Parameter 2A", "Channel (0: A)"=w797, "VISA resource name"=w789) -> ("error out"=w798:errorcluster, "Measurement"=w806:dbl, "VISA resource name out"=w811:refnum<visa-resource-name>)  [unwired: 5 in]
                                n193 = call "OE1022D_Read 1 parameter_mean.vi"("Parameter 2"="Parameter 2B", "错误输入（无错误）"=w795, "Channel (0: A)"=w794, "VISA resource name"=w789) -> ("error out"=w792:errorcluster, "Measurement"=w791:dbl, "VISA resource name out"=w793:refnum<visa-resource-name>)  [unwired: 5 in]
                                n194 = Multiply(x=w806, y=1000.0) -> (x*y=w804:dbl)
                                "Vaa_2(1w)/mV" <- w804
                                n195 = Multiply(x=w791, y=1000000.0) -> (x*y=w802:dbl)
                                "para2B Measurement" <- w802
                                n196 = Build Array(w804) -> (w814:dbl[])
                                n197 = Build Array(w802) -> (w808:dbl[])
                                n198 = Select(t=w814, s="T Clear Plot 2A", f=w788) -> (s? t:f=w803:dbl[])
                                n199 = Select(t=w808, s="T Clear Plot 2B", f=w787) -> (s? t:f=w801:dbl[])
                                n200 = Build Array (concatenate)(w813, w786) -> (w805:dbl[])
                              }
                              frame #1 {
                                n201 = Wait (ms)(milliseconds to wait=u32 50) -> ()  [unwired: 1 out]
                              }
                              frame #2 {
                                n202 = Build Array (concatenate)(w858, w857) -> (w856:dbl[])
                                n203 = Build Array (concatenate)(w862, w861) -> (w860:dbl[])
                                n204 = Bundle(w867, w860) -> (→"Vaa_2/mV":cluster{dbl[], dbl[]})  [unwired: 1 in]
                                n205 = call "OE1022D_Read 1 parameter_mean.vi"("错误输入（无错误）"=w845, "Parameter"="Phase 2A", "Channel (0: A)"=w844, "VISA resource name"=w843) -> ("error out"=w842:errorcluster, "Measurement"=w841:dbl)  [unwired: 5 in, 1 out]
                                "phase Vaa_2" <- w841
                                n206 = Bundle(w869, w856) -> (→"R2B-T":cluster{dbl[], dbl[]})  [unwired: 1 in]
                                n207 = call "OE1022D_Read 1 parameter_mean.vi"("Parameter 2"="Phase 2B", "错误输入（无错误）"=w849, "Channel (0: A)"=w838, "VISA resource name"=w848) -> ("Measurement"=w847:dbl)  [unwired: 5 in, 2 out]
                                "phase 2B" <- w847
                                n208 = Build Array(w841) -> (w850:dbl[])
                                n209 = Build Array(w847) -> (w851:dbl[])
                                n210 = Select(t=w850, s=w853, f=w854) -> (s? t:f=w852:dbl[])
                                n211 = Select(t=w851, s=w836, f=w839) -> (s? t:f=w855:dbl[])
                                n212 = Build Array (concatenate)(w841, w852) -> (w863:dbl[])
                                n213 = Build Array (concatenate)(w847, w855) -> (w859:dbl[])
                                n214 = Bundle(w865, w863) -> (→"phase Vaa_2":cluster{dbl[], dbl[]})  [unwired: 1 in]
                                n215 = Bundle(w837, w859) -> (→"Phase2B-T":cluster{dbl[], dbl[]})  [unwired: 1 in]
                              }
                              frame #3 {
                                n216 = Wait (ms)(milliseconds to wait=u32 50) -> ()  [unwired: 1 out]
                              }
                              frame #4 {
                                n217 = call "OE1022D_Read 1 parameter_mean.vi"("Parameter 2"="Parameter 2B 1", "错误输入（无错误）"=w894, "Channel (0: A)"=w908, "VISA resource name"=w909) -> ("Measurement"=w892:dbl)  [unwired: 5 in, 2 out]
                                n218 = call "OE1022D_Read 1 parameter_mean.vi"("Parameter 2"="Phase 2B 1", "错误输入（无错误）"=w894, "Channel (0: A)"=w908, "VISA resource name"=w909) -> ("Measurement"=w901:dbl)  [unwired: 5 in, 2 out]
                                "phase Vab_2" <- w901
                                n219 = Multiply(x=1000.0, y=w892) -> (x*y=w891:dbl)
                                "Vab_2(1w)/mV" <- w891
                                n220 = Build Array(w891) -> (w907:dbl[])
                                n221 = Build Array(w901) -> (w904:dbl[])
                                n222 = Select(t=w907, s=w896, f=w895) -> (s? t:f=w906:dbl[])
                                n223 = Select(t=w904, s=w896, f=w897) -> (s? t:f=w903:dbl[])
                                n224 = Build Array (concatenate)(w891, w906) -> (w898:dbl[])
                                n225 = Build Array (concatenate)(w901, w903) -> (w899:dbl[])
                                n226 = Bundle(w900, w898) -> (→"Vab_2/mV":cluster{dbl[], dbl[]})  [unwired: 1 in]
                                n227 = Bundle(w900, w899) -> (→"phase Vab_2":cluster{dbl[], dbl[]})  [unwired: 1 in]
                              }
                            }
                          }
                        }
                        n228 = flat-sequence {
                          tunnel: w583 -> [w946]
                          tunnel: w584 -> [w945]
                          tunnel: w582 -> [w939]
                          tunnel: [w943] -> w646
                          tunnel: [w935] -> w645
                          tunnel: [w936] -> w644
                          tunnel: [w933] -> w643
                          tunnel: [w936] -> w642
                          tunnel: [w936] -> w641
                          tunnel: [w936] -> w640
                          tunnel: [w936] -> w639
                          tunnel: [w935] -> w638
                          tunnel: [w934] -> w637
                          tunnel: [w933] -> w636
                          tunnel: [w932] -> w635
                          tunnel: ["T Clear Plot 1B"] -> w634
                          tunnel: ["T Clear Plot 1A"] -> w633
                          tunnel: [w923] -> w632
                          tunnel: [w925] -> w631
                          tunnel: [w924] -> w630
                          tunnel: [w929] -> w629
                          tunnel: [w928] -> w628
                          tunnel: w588 -> [w920]
                          tunnel: w567 -> [w919]
                          tunnel: w646 -> [w968]
                          tunnel: [w968] -> w627
                          tunnel: w645 -> [w967]
                          tunnel: [w967] -> w626
                          tunnel: w644 -> [w966]
                          tunnel: [w966] -> w625
                          tunnel: w643 -> [w965]
                          tunnel: [w965] -> w624
                          tunnel: w642 -> [w964]
                          tunnel: [w964] -> w623
                          tunnel: w641 -> [w963]
                          tunnel: [w963] -> w622
                          tunnel: w640 -> [w962]
                          tunnel: [w962] -> w621
                          tunnel: w639 -> [w961]
                          tunnel: [w961] -> w620
                          tunnel: w638 -> [w960]
                          tunnel: [w960] -> w619
                          tunnel: w637 -> [w959]
                          tunnel: [w959] -> w618
                          tunnel: w636 -> [w958]
                          tunnel: [w958] -> w617
                          tunnel: w635 -> [w957]
                          tunnel: [w957] -> w616
                          tunnel: w634 -> [w956]
                          tunnel: [w956] -> w615
                          tunnel: w633 -> [w955]
                          tunnel: [w955] -> w614
                          tunnel: w632 -> [w954]
                          tunnel: [w954] -> w613
                          tunnel: w631 -> [w953]
                          tunnel: [w953] -> w612
                          tunnel: w630 -> [w952]
                          tunnel: [w952] -> w611
                          tunnel: w629 -> [w951]
                          tunnel: [w951] -> w610
                          tunnel: w628 -> [w950]
                          tunnel: [w950] -> w609
                          tunnel: w627 -> [w975]
                          tunnel: w626 -> [w1006]
                          tunnel: w625 -> [w1005]
                          tunnel: w624 -> [w1004]
                          tunnel: w623 -> [w1003]
                          tunnel: w622 -> [w1001]
                          tunnel: w621 -> [w999]
                          tunnel: w620 -> [w970]
                          tunnel: w619 -> [w995]
                          tunnel: w618 -> [w994]
                          tunnel: w617 -> [w991]
                          tunnel: w616 -> [w990]
                          tunnel: w578 -> [w988]
                          tunnel: w615 -> [w969]
                          tunnel: w579 -> [w986]
                          tunnel: w614 -> [w985]
                          tunnel: w613 -> [w981]
                          tunnel: w612 -> [w971]
                          tunnel: w611 -> [w980]
                          tunnel: w610 -> [w977]
                          tunnel: w609 -> [w976]
                          tunnel: [w975] -> w608
                          tunnel: [w993] -> w607
                          tunnel: [w1006] -> w606
                          tunnel: [w1005] -> w605
                          tunnel: [w973] -> w604
                          tunnel: [w974] -> w603
                          tunnel: [w996] -> w602
                          tunnel: [w992] -> w601
                          tunnel: [w989] -> w600
                          tunnel: [w1004] -> w599
                          tunnel: [w979] -> w598
                          tunnel: [w971] -> w546
                          tunnel: [w970] -> w542
                          tunnel: [w969] -> w540
                          tunnel: w608 -> [w1021]
                          tunnel: w607 -> [w1020]
                          tunnel: w606 -> [w1019]
                          tunnel: w605 -> [w1018]
                          tunnel: w604 -> [w1017]
                          tunnel: w603 -> [w1016]
                          tunnel: w602 -> [w1015]
                          tunnel: w601 -> [w1014]
                          tunnel: w600 -> [w1013]
                          tunnel: w599 -> [w1012]
                          tunnel: w598 -> [w1011]
                          tunnel: [w1021] -> w566
                          tunnel: [w1020] -> w565
                          tunnel: [w1019] -> w564
                          tunnel: [w1018] -> w563
                          tunnel: [w1017] -> w562
                          tunnel: [w1016] -> w561
                          tunnel: [w1015] -> w560
                          tunnel: [w1014] -> w559
                          tunnel: [w1013] -> w558
                          tunnel: [w1012] -> w557
                          tunnel: [w1011] -> w556
                          tunnel: [w1009] -> w547
                          tunnel: w546 -> [w1009]
                          tunnel: [w1008] -> w543
                          tunnel: w542 -> [w1008]
                          tunnel: [w1007] -> w541
                          tunnel: w540 -> [w1007]
                          tunnel: [w1043] -> w590
                          tunnel: [w1044] -> w591
                          tunnel: [w1045] -> w586
                          tunnel: [w1046] -> w580
                          tunnel: [w1047] -> w581
                          tunnel: [w1048] -> w589
                          tunnel: [w1049] -> w587
                          tunnel: [w1050] -> w592
                          tunnel: [w1051] -> w585
                          tunnel: w566 -> [w1042]
                          tunnel: w565 -> [w1051]
                          tunnel: w564 -> [w1050]
                          tunnel: w563 -> [w1049]
                          tunnel: w562 -> [w1048]
                          tunnel: w561 -> [w1041]
                          tunnel: w560 -> [w1047]
                          tunnel: w559 -> [w1046]
                          tunnel: w558 -> [w1045]
                          tunnel: w557 -> [w1044]
                          tunnel: w556 -> [w1043]
                          tunnel: w547 -> [w1040]
                          tunnel: [w1023] -> w545
                          tunnel: [w1032] -> w544
                          tunnel: w543 -> [w1031]
                          tunnel: w541 -> [w1030]
                          tunnel: [w1029] -> w539
                          tunnel: [w1028] -> w538
                          tunnel: w537 -> [w1027]
                          tunnel: w536 -> [w1026]
                          frame #0 {
                            w925 = u8 1 items=["Channel A", "Channel B"] ("Channel A/B for Parameter1")
                            w928 = u8 0 items=["Channel A", "Channel B"] ("Channel A/B for Parameter1")
                            n229 = Format Into String(0) -> (error out=w926:errorcluster)  [unwired: 3 in, 1 out]
                            n230 = Format Into String(0) -> (error out=w944:errorcluster)  [unwired: 3 in, 1 out]
                            n231 = call "OE1022D_Read 1 parameter_mean.vi"("Parameter 2"="Parameter 1B", "错误输入（无错误）"=w926, "Channel (0: A)"=w925, "VISA resource name"=w919) -> ("error out"=w923:errorcluster, "Measurement"=w922:dbl, "VISA resource name out"=w924:refnum<visa-resource-name>)  [unwired: 5 in]
                            n232 = call "OE1022D_Read 1 parameter_mean.vi"("错误输入（无错误）"=w944, "Parameter"="Parameter 1A", "Channel (0: A)"=w928, "VISA resource name"=w919) -> ("error out"=w929:errorcluster, "Measurement"=w937:dbl, "VISA resource name out"=w943:refnum<visa-resource-name>)  [unwired: 5 in]
                            n233 = Multiply(x=w922, y=1000000.0) -> (x*y=w933:dbl)
                            "para1B Measurement" <- w933
                            n234 = Multiply(x=w937, y=1000.0) -> (x*y=w935:dbl)
                            "Vaa_1(1w)/mV" <- w935
                            n235 = Build Array(w933) -> (w940:dbl[])
                            n236 = Build Array(w935) -> (w947:dbl[])
                            n237 = Build Array (concatenate)(w920, w945) -> (w936:dbl[])
                            n238 = Select(t=w940, s="T Clear Plot 1B", f=w939) -> (s? t:f=w932:dbl[])
                            n239 = Select(t=w947, s="T Clear Plot 1A", f=w946) -> (s? t:f=w934:dbl[])
                          }
                          frame #1 {
                            n240 = Wait (ms)(milliseconds to wait=u32 50) -> ()  [unwired: 1 out]
                          }
                          frame #2 {
                            n241 = Build Array (concatenate)(w995, w994) -> (w993:dbl[])
                            n242 = Build Array (concatenate)(w991, w990) -> (w989:dbl[])
                            n243 = Bundle(w999, w993) -> (→"Vaa_1/mV":cluster{dbl[], dbl[]})  [unwired: 1 in]
                            n244 = Bundle(w1001, w989) -> (→"R1B-T":cluster{dbl[], dbl[]})  [unwired: 1 in]
                            n245 = call "OE1022D_Read 1 parameter_mean.vi"("Parameter 2"="Phase 1B", "错误输入（无错误）"=w981, "Channel (0: A)"=w971, "VISA resource name"=w980) -> ("Measurement"=w979:dbl)  [unwired: 5 in, 2 out]
                            "phase 1B" <- w979
                            n246 = Build Array(w979) -> (w983:dbl[])
                            n247 = call "OE1022D_Read 1 parameter_mean.vi"("错误输入（无错误）"=w977, "Parameter"="Phase 1A", "Channel (0: A)"=w976, "VISA resource name"=w975) -> ("error out"=w974:errorcluster, "Measurement"=w973:dbl)  [unwired: 5 in, 1 out]
                            "phase Vaa_1" <- w973
                            n248 = Select(t=w983, s=w969, f=w988) -> (s? t:f=w987:dbl[])
                            n249 = Build Array (concatenate)(w979, w987) -> (w992:dbl[])
                            n250 = Build Array(w973) -> (w982:dbl[])
                            n251 = Select(t=w982, s=w985, f=w986) -> (s? t:f=w984:dbl[])
                            n252 = Bundle(w1003, w992) -> (→"Phase1B-T":cluster{dbl[], dbl[]})  [unwired: 1 in]
                            n253 = Build Array (concatenate)(w973, w984) -> (w996:dbl[])
                            n254 = Bundle(w970, w996) -> (→"phase Vaa_1":cluster{dbl[], dbl[]})  [unwired: 1 in]
                          }
                          frame #3 {
                            n255 = Wait (ms)(milliseconds to wait=u32 50) -> ()  [unwired: 1 out]
                          }
                          frame #4 {
                            n256 = call "OE1022D_Read 1 parameter_mean.vi"("Parameter 2"="Phase 1B 1", "错误输入（无错误）"=w1041, "Channel (0: A)"=w1040, "VISA resource name"=w1042) -> ("Measurement"=w1032:dbl)  [unwired: 5 in, 2 out]
                            "phase Vab_1" <- w1032
                            n257 = call "OE1022D_Read 1 parameter_mean.vi"("错误输入（无错误）"=w1041, "Parameter"="Parameter 1B 1", "Channel (0: A)"=w1040, "VISA resource name"=w1042) -> ("Measurement"=w1024:dbl)  [unwired: 5 in, 2 out]
                            n258 = Build Array(w1024) -> (w1037:dbl[])
                            n259 = Build Array(w1032) -> (w1038:dbl[])
                            n260 = Multiply(x=1000.0 ("y"), y=w1024) -> (x*y=w1023:dbl)
                            "Vab_1(1w)/mV" <- w1023
                            n261 = Select(t=w1037, s=w1030, f=w1026) -> (s? t:f=w1033:dbl[])
                            n262 = Select(t=w1038, s=w1030, f=w1027) -> (s? t:f=w1036:dbl[])
                            n263 = Build Array (concatenate)(w1023, w1033) -> (w1028:dbl[])
                            n264 = Build Array (concatenate)(w1032, w1036) -> (w1029:dbl[])
                            n265 = Bundle(w1031, w1028) -> (→"Vab_1/mV":cluster{dbl[], dbl[]})  [unwired: 1 in]
                            n266 = Bundle(w1031, w1029) -> (→"phase Vab_1":cluster{dbl[], dbl[]})  [unwired: 1 in]
                          }
                        }
                        n267 = case shown="True" w535 {
                          tunnel: w534 -> [_ w655]
                          frame False {
                          }
                          frame True {
                            n268 = flat-sequence {
                              tunnel: w655 -> [w669]
                              tunnel: [w668] -> w653
                              tunnel: [w667] -> w652
                              tunnel: [w666] -> w649
                              tunnel: [w665] -> w647
                              tunnel: [w678] -> w654
                              tunnel: w653 -> [w678]
                              tunnel: w652 -> [w677]
                              tunnel: [w677] -> w651
                              tunnel: [w676] -> w650
                              tunnel: w649 -> [w676]
                              tunnel: [w675] -> w648
                              tunnel: w647 -> [w675]
                              tunnel: w654 -> [w689]
                              tunnel: w651 -> [w688]
                              tunnel: w650 -> [w687]
                              tunnel: w648 -> [w686]
                              frame #0 {
                                w662 = u16 2 items=["X", "Y", "R", "Theta", "Frequency", "Noise", "Xh1", "Yh1", "Rh1", "Theta h1", "Xh2", "Yh2", "Rh2", "Theta h2"] ("Parameter 2")
                                w663 = u16 2 items=["X", "Y", "R", "Theta", "Frequency", "Noise", "Xh1", "Yh1", "Rh1", "Theta h1", "Xh2", "Yh2", "Rh2", "Theta h2"] ("Parameter")
                                w664 = u16 1 items=["Channel A", "Channel B", "ADC"] ("Channel (0: A)")
                                w670 = u16 0 items=["Channel A", "Channel B", "ADC"] ("Channel (0: A)")
                                n269 = Format Into String(0) -> (error out=w672:errorcluster)  [unwired: 3 in, 1 out]
                                n270 = Format Into String(0) -> (error out=w671:errorcluster)  [unwired: 3 in, 1 out]
                                n271 = call "OE1022D_Read 1 parameter_mean.vi"("错误输入（无错误）"=w672, "Parameter"=w663, "Channel (0: A)"=w670, "VISA resource name"=w669) -> ("error out"=w667:errorcluster, "Measurement"=w661:dbl, "VISA resource name out"=w668:refnum<visa-resource-name>)  [unwired: 5 in]
                                n272 = call "OE1022D_Read 1 parameter_mean.vi"("Parameter 2"=w662, "错误输入（无错误）"=w671, "Channel (0: A)"=w664, "VISA resource name"=w669) -> ("error out"=w665:errorcluster, "Measurement"=w658:dbl, "VISA resource name out"=w666:refnum<visa-resource-name>)  [unwired: 5 in]
                                n273 = local read "R2(Kohm)"() -> (w659:dbl)
                                n274 = local read "R1(Kohm)"() -> (w660:dbl)
                                n275 = Divide(x=w658, y=w659) -> (x/y=→"Device2 Current(mA)":dbl)
                                n276 = Divide(x=w661, y=w660) -> (x/y=→"Device1 Current(mA)":dbl)
                              }
                              frame #1 {
                                n277 = Wait (ms)(milliseconds to wait=u32 50) -> ()  [unwired: 1 out]
                              }
                              frame #2 {
                                w682 = u16 3 items=["X", "Y", "R", "Theta", "Frequency", "Noise", "Xh1", "Yh1", "Rh1", "Theta h1", "Xh2", "Yh2", "Rh2", "Theta h2"] ("Parameter 2")
                                w683 = u16 1 items=["Channel A", "Channel B", "ADC"] ("Channel (0: A)")
                                w684 = u16 3 items=["X", "Y", "R", "Theta", "Frequency", "Noise", "Xh1", "Yh1", "Rh1", "Theta h1", "Xh2", "Yh2", "Rh2", "Theta h2"] ("Parameter")
                                w685 = u16 0 items=["Channel A", "Channel B", "ADC"] ("Channel (0: A)")
                                n278 = call "OE1022D_Read 1 parameter_mean.vi"("错误输入（无错误）"=w688, "Parameter"=w684, "Channel (0: A)"=w685, "VISA resource name"=w689) -> ("Measurement"=→"Device 1 phase":dbl)  [unwired: 5 in, 2 out]
                                n279 = call "OE1022D_Read 1 parameter_mean.vi"("Parameter 2"=w682, "错误输入（无错误）"=w686, "Channel (0: A)"=w683, "VISA resource name"=w687) -> ("Measurement"=→"Device 2 phase":dbl)  [unwired: 5 in, 2 out]
                              }
                              frame #3 {
                                n280 = Wait (ms)(milliseconds to wait=u32 50) -> ()  [unwired: 1 out]
                              }
                            }
                          }
                        }
                        n281 = local read "Sine voltage T"() -> (w549:dbl)
                        n282 = local read "Frequency"() -> (w548:dbl)
                      }
                      frame #3 {
                        n283 = local read "Sine voltage T"() -> (w1070:dbl)
                        n284 = local read "Device1 Current(mA)"() -> (w1085:dbl)
                        n285 = local read "Vaa_1(1w)/mV"() -> (w1086:dbl)
                        n286 = local read "Vaa_2(1w)/mV"() -> (w1084:dbl)
                        n287 = local read "Device2 Current(mA)"() -> (w1083:dbl)
                        n288 = Build Array (concatenate)(w1070, w1063) -> (w1060:dbl[])
                        n289 = Divide(x=w1086, y=w1085) -> (x/y=w1062:dbl)
                        "Ri_1(Ohm)" <- w1062
                        n290 = Divide(x=w1084, y=w1083) -> (x/y=w1061:dbl)
                        "Ri_2(Ohm)" <- w1061
                        n291 = local read "T Clear Plot 2A"() -> (w1067:bool)
                        n292 = local read "T Clear Plot 1A"() -> (w1066:bool)
                        n293 = Build Array(w1061) -> (w1081:dbl[])
                        n294 = Build Array(w1062) -> (w1082:dbl[])
                        n295 = Select(t=w1081, s=w1067, f=w1054) -> (s? t:f=w1071:dbl[])
                        n296 = Select(t=w1082, s=w1066, f=w1058) -> (s? t:f=w1078:dbl[])
                        n297 = Build Array (concatenate)(w1061, w1071) -> (w1055:dbl[])
                        n298 = Build Array (concatenate)(w1062, w1078) -> (w1059:dbl[])
                        n299 = Bundle(w1060, w1055) -> (→"Ri_2":cluster{dbl[], dbl[]})  [unwired: 1 in]
                        n300 = Bundle(w1060, w1059) -> (→"Ri_1":cluster{dbl[], dbl[]})  [unwired: 1 in]
                        n301 = local read "T Clear Plot 1B"() -> (w1069:bool)
                        n302 = local read "T Clear Plot 2B"() -> (w1068:bool)
                        n303 = local read "Device 1 phase"() -> (w1065:dbl)
                        n304 = local read "Device 2 phase"() -> (w1064:dbl)
                        n305 = Build Array(w1065) -> (w1077:dbl[])
                        n306 = Build Array(w1064) -> (w1074:dbl[])
                        n307 = Select(t=w1077, s=w1069, f=w1056) -> (s? t:f=w1075:dbl[])
                        n308 = Select(t=w1074, s=w1068, f=w1052) -> (s? t:f=w1072:dbl[])
                        n309 = Build Array (concatenate)(w1065, w1075) -> (w1057:dbl[])
                        n310 = Build Array (concatenate)(w1064, w1072) -> (w1053:dbl[])
                        n311 = Bundle(w1060, w1057) -> (→"Ri_1 phase":cluster{dbl[], dbl[]})  [unwired: 1 in]
                        n312 = Bundle(w1060, w1053) -> (→"Ri_2 phase":cluster{dbl[], dbl[]})  [unwired: 1 in]
                      }
                    }
                    n313 = case shown="True" w485 {
                      tunnel: w475 -> [_ w1131]
                      tunnel: w508 -> [_ w1136]
                      tunnel: w509 -> [_ w1137]
                      tunnel: w506 -> [_ w1135]
                      tunnel: w507 -> [_ w1134]
                      tunnel: w476 -> [_ w1133]
                      tunnel: w513 -> [_ w1130]
                      tunnel: w512 -> [_ w1129]
                      tunnel: w511 -> [_ w1128]
                      tunnel: w510 -> [_ w1127]
                      tunnel: w476 -> [_ w1126]
                      tunnel: w484 -> [_ w1124]
                      tunnel: w483 -> [_ w1125]
                      tunnel: w482 -> [_ w1123]
                      tunnel: w481 -> [_ w1122]
                      tunnel: w474 -> [_ w1121]
                      tunnel: w473 -> [_ w1120]
                      tunnel: w468 -> [_ w1119]
                      tunnel: w467 -> [_ w1118]
                      tunnel: w466 -> [_ w1117]
                      tunnel: w465 -> [_ w1116]
                      frame False {
                      }
                      frame True {
                        n314 = Build Array(w1131, w1133, w1137, w1135, w1136, w1134, w1121, w1120, w1119, w1118) -> (w1139:dbl[])
                        n315 = local read "Two Devices ?"() -> (w1132:bool)
                        n316 = call-poly <vilib>:"Write Delimited Spreadsheet.vi"("file path (dialog if empty)"=w1124, "format (%.3f)"="%.10f", "1D data"=w1139, "append to file? (new file:F)"=TRUE) -> ()  [unwired: 10 in, 2 out]
                        n317 = case shown="True" w1132 {
                          tunnel: w1131 -> [_ w1151]
                          tunnel: w1130 -> [_ w1150]
                          tunnel: w1129 -> [_ w1149]
                          tunnel: w1128 -> [_ w1148]
                          tunnel: w1127 -> [_ w1147]
                          tunnel: w1126 -> [_ w1146]
                          tunnel: w1125 -> [_ w1145]
                          tunnel: w1123 -> [_ w1144]
                          tunnel: w1122 -> [_ w1143]
                          tunnel: w1117 -> [_ w1142]
                          tunnel: w1116 -> [_ w1141]
                          frame False {
                          }
                          frame True {
                            n318 = Build Array(w1151, w1146, w1150, w1148, w1149, w1147, w1143, w1144, w1141, w1142) -> (w1153:dbl[])
                            n319 = call-poly <vilib>:"Write Delimited Spreadsheet.vi"("file path (dialog if empty)"=w1145, "format (%.3f)"="%.10f", "1D data"=w1153, "append to file? (new file:F)"=TRUE) -> ()  [unwired: 10 in, 2 out]
                          }
                        }
                      }
                    }
                  }
                }
              }
            }
            n320 = local read "End Value (Hz)"() -> (w378:dbl)
            n321 = local read "Frequency"() -> (w384:dbl)
            n322 = Logarithm Base 10(1:w378) -> (0:w379:dbl)
            n323 = Round Toward -Infinity(1:w379) -> (0:w377:dbl)
            n324 = local read "Log Step"() -> (w374:dbl)
            n325 = Power Of 10(x=w377) -> (10^x=w380:dbl)
            n326 = Multiply(x=w374, y=w380) -> (x*y=w376:dbl)
            n327 = Subtract(x=w378, y=w376) -> (x-y=w375:dbl)
            n328 = Greater Or Equal?(x=w384, y=w375) -> (x >= y?=w385:bool)
          }
        }
      }
    }
    frame #2 {
      n329 = local read "Instrument Ref Out"() -> (w1156:refnum<k24>)
      n330 = local read "error out"() -> (w1155:errorcluster)
      n331 = case shown="True" "Initialization?" {
        tunnel: w1155 -> [w1158 w1161]
        tunnel: w1156 -> [w1159 w1160]
        frame False {
          n332 = Close Reference(reference=w1159, error in (no error)=w1158) -> ()  [unwired: 1 out]
        }
        frame True {
          w1167 = 0 items=["Linear", "NoOvershoot", "Oscillate"] ("Approach")
          w1168 = 0 items=["Persistent", "Driven"] ("Mode")
          w1164 = 0 items=["FastSettle", "NoOvershoot"] ("Approach")
          n333 = call "SetTemperature.vi"("Approach"=w1164, "Rate"=20.0, "Temperature"=1.6, "error in (no error)"=w1161, "Instrument Ref In"=w1160) -> ("error out"=w1172:errorcluster, "Instrument Ref Out"=w1171:refnum<k24>)  [unwired: 2 in, 1 out]
          n334 = call "SetField.vi"("Mode"=w1168, "Approach"=w1167, "Rate"=200.0, "Field"=0.0, "error in (no error)"=w1172, "Instrument Ref In"=w1171) -> ("error out"=w1169:errorcluster, "Instrument Ref Out"=w1170:refnum<k24>)  [unwired: 1 in, 1 out]
          n335 = Close Reference(reference=w1170, error in (no error)=w1169) -> ()  [unwired: 1 out]
        }
      }
    }
  }
  n336 = local read "Temperature \n& Field Function"() -> (w21:bool)
  n337 = case shown="True" w21 {
    tunnel: [w1173 w1180] -> w15
    tunnel: [w1173 w1176] -> w16
    frame False {
      w1173 = ""
    }
    frame True {
      n338 = local read "Set F (Oe)"() -> (w1174:dbl)
      n339 = local read "Set  T  (K)"() -> (w1175:dbl)
      n340 = Format Into String(format string="%.0fOe", initial string="at", w1174) -> (resulting string=w1180:string)  [unwired: 1 in, 1 out]
      n341 = Format Into String(format string="%d", initial string="at", w1175) -> (resulting string=w1176:string)  [unwired: 1 in, 1 out]
    }
  }
  n342 = Format Into String(format string="%dKohm", "R1(Kohm)") -> (resulting string=w6:string)  [unwired: 2 in, 1 out]
  n343 = local read "Two Devices ?"() -> (w9:bool)
  n344 = case shown="True" w9 {
    tunnel: [w1182 w1183] -> w5
    tunnel: w6 -> [w1182 _]
    frame False {
    }
    frame True {
      n345 = Format Into String(format string="%dKohm", "R2(Kohm)") -> (resulting string=w1183:string)  [unwired: 2 in, 1 out]
    }
  }
  n346 = local read "End Value (Hz)"() -> (w3:dbl)
  n347 = local read "Start Value (Hz)"() -> (w20:dbl)
  n348 = Format Into String(format string="%fHz", initial string="from", w20) -> (resulting string=w14:string)  [unwired: 1 in, 1 out]
  n349 = Format Into String(format string="%fHz", initial string="to", w3) -> (resulting string=w1:string)  [unwired: 1 in, 1 out]
  n350 = Format Into String(initial string="path1 (folder + filename)", w16, w15, w14, w1, w5, w13) -> (resulting string=w24:string)  [unwired: 2 in, 1 out]
  n351 = String To Path(string=w24) -> (path=w12:path)
  n352 = Format Into String(initial string="path2 (folder + filename)", w16, w15, w14, w1, w5, w13) -> (resulting string=w23:string)  [unwired: 2 in, 1 out]
  n353 = String To Path(string=w23) -> (path=w11:path)
